vi "Striptest.vi"(1 "Simulation?":bool) -> ()   [LabVIEW 2018]
uses:
  InstrControl/ProbeStationControl/TeslaVelox/TeslaVeloxProbeStation.lvclass
  C:/Users/itkstriplabview4/Documents/itk-strip-sensor-qc/InstrControl/ProbeStationControl/ProbeStationControl.lvclass
  general_VIs/globals/QC_MeasurementSetup.vi
  striptest/ProbePlan/ProbePlanParams.vi
  general_VIs/globals/QC_RunInformation.vi
  InstrControl/InstrumentSetup.vi
  <vilib>/regexp/Match Regular Expression.xnode
  InstrControl/SupplyControl/SupplyControl.lvclass
  InstrControl/Switching/Switching.lvclass
  InstrControl/ProbeStationControl/ProbeStationControl.lvclass
  InstrControl/LCRControl/LCRControl.lvclass
  InstrControl/InstrControl.lvclass
  InstrControl/ArduinoControl/ArduinoControl.lvclass
  <vilib>/Analysis/NI_AALBase.lvlib
  InstrControl/ProbeStationControl/TeslaVelox/TeslaVelox_GlobalConfig.vi
  InstrControl/Switching/Pickering/Pickering.lvclass
  <instrlib>/CascadeProbestation/CascadeProbestation.lvlib
  C:/Users/itkstriplabview4/Documents/itk-strip-sensor-qc/InstrControl/Switching/Switching.lvclass
panel:
  in  "PreSave Data":bool
  out "RH [%]":dbl=35.18 format="%.2f"
  out "Temp [°C]":dbl=22.06 format="%.2f"
  in  "settling\ndelay [ms]":i32=1000
  in  "Auto quit &\nswitch off bias":bool
  in  "Rolling\nCurrent Readout":bool
  out "Status":string="Saving data for Segment\t3T"
  in  "Set display for:":u16(ring)=3
  out "Initiated:":string
  out "Defects":i32[][](graph)=[[0], [1], [1], [1], [1], [1], [1], [1], [1], [1], [1], [1], [1], [1], [1], [1], [1], [1], [1], [1], [1], [1], [1], [1], [1], [1], [1], [1], [1], [1], [1], [1], [1], [1], [1], [1], [1], [1], [1], [1], [1], [1], [1], [1], [1], [1], [1], [1], [1], [1], [1], [1], [1], [1], [1], [1], [1], [1], [1], [1], [1], [1], [1], [1], [1], [1], [1], [1], [1], [1], [1], [1], [1], [1], [1], [1], [1], [1], [1], [1], [1], [1], [1], [1], [1], [1], [1], [1], [1], [1], [1], [1], [1], [1], [1], [1], [1], [1], [1], [1], [1], [1], [1], [1], [1], [1], [1], [1], [1], [1], [1], [1], [1], [1], [1], [1], [1], [1], [1], [1], [1], [1], [1], [1], [1], [1], [1], [1], [1], [1], [1], [1], [1], [1], [1], [1], [1], [1], [1], [1], [1], [1], [1], [1], [1], [1], [1], [1], [1], [1], [1], [1], [1], [1], [1], [1], [1], [1], [1], [1], [1], [1], [1], [1], [1], [1], [1], [1], [1], [1], [1], [1], [1], [1], [1], [1], [1], [1], [1], [1], [1], [1], [1], [1], [1], [1], [1], [1], [1], [1], [1], [1], [1], [1], [1], [1], [1], [1], [1], [1], [1], [1], [1], [1], [1], [1], [1], [1], [1], [1], [1], [1], [1], [1], [1], [1], [1], [1], [1], [1], [1], [1], [1], [1], [1], [1], [1], [1], [1], [1], [1], [1], [1], [1], [1], [1], [1], [1], [1], [1], [1], [1], [1], [1], [1], [1], [1], [1], [1], [1], [1], [1], [1], [1], [1], [1], [1], [1], [1], [1], [1], [1], [1], [1], [1], [1], [1], [1], [1], [1], [1], [1], [1], [1], [1], [1], [1], [1], [1], [1], [1], [1], [1], [1], [1], [1], [1], [1], [1], [1], [1], [1], [1], [1], [1], [1], [1], [1], [1], [1], [1], [1], [1], [1], [1], [1], [1], [1], [1], [1], [1], [1], [1], [1], [1], [1], [1], [1], [1], [1], [1], [1], [1], [1], [1], [1], [1], [1], [1], [1], [1], [1], [1], [1], [1], [1], [1], [1], [1], [1], [1], [1], [1], [1], [1], [1], [1], [1], [1], [1], [1], [1], [1], [1], [1], [1], [1], [1], [1], [1], [1], [1], [1], [1], [1], [1], [1], [1], [1], [1], [1], [1], [1], [1], [1], [1], [1], [1], [1], [1], [1], [1], [1], [1], [1], [1], [1], [1], [1], [1], [1], [1], [1], [1], [1], [1], [1], [1], [1], [1], [1], [1], [1], [1], [1], [1], [1], [1], [1], [1], [1], [1], [1], [1], [1], [1], [1], [1], [1], [1], [1], [1], [1], [1], [1], [1], [1], [1], [1], [1], [1], [1], [1], [1], [1], [1], [1], [1], [1], [1], [1], [1], [1], [1], [1], [1], [1], [1], [1], [1], [1], [1], [1], [1], [1], [1], [1], [1], [1], [1], [1], [1], [1], [1], [1], [1], [1], [1], [1], [1], [1], [1], [1], [1], [1], [1], [1], [1], [1], [1], [1], [1], [1], [1], [1], [1], [1], [1], [1], [1], [1], [1], [1], [1], [1], [1], [1], [1], [1], [1], [1], [1], [1], [1], [1], [1], [1], [1], [1], [1], [1], [1], [1], [1], [1], [1], [1], [1], [1], [1], [1], [1], [1], [1], [1], [1], [1], [1], [1], [1], [1], [1], [1], [1], [1], [1], [1], [1], [1], [1], [1], [1], [1], [1], [1], [1], [1], [1], [1], [1], [1], [1], [1], [1], [1], [1], [1], [1], [1], [1], [1], [1], [1], [1], [1], [1], [1], [1], [1], [1], [1], [1], [1], [1], [1], [1], [1], [1], [1], [1], [1], [1], [1], [1], [1], [1], [1], [1], [1], [1], [1], [1], [1], [1], [1], [1], [1], [1], [1], [1], [1], [1], [1], [1], [1], [1], [1], [1], [1], [1], [1], [1], [1], [1], [1], [1], [1], [1], [1], [1], [1], [1], [1], [1], [1], [1], [1], [1], [1], [1], [1], [1], [1], [1], [1], [1], [1], [1], [1], [1], [1], [1], [1], [1], [1], [1], [1], [1], [1], [1], [1], [1], [1], [1], [1], [1], [1], [1], [1], [1], [1], [1], [1], [1], [1], [1], [1], [1], [1], [1], [1], [1], [1], [1], [1], [1], [1], [1], [1], [1], [1], [1], [1], [1], [1], [1], [1], [1], [1], [1], [1], [1], [1], [1], [1], [1], [1], [1], [1], [1], [1], [1], [1], [1], [1], [1], [1], [1], [1], [1], [1], [1], [1], [1], [1], [1], [1], [1], [1], [1], [1], [1], [1], [1], [1], [1], [1], [1], [1], [1], [1], [1], [1], [1], [1], [1], [1], [1], [1], [1], [1], [1], [1], [1], [1], [1], [1], [1], [1], [1], [1], [1], [1], [1], [1], [1], [1], [1], [1], [1], [1], [1], [1], [1], [1], [1], [1], [1], [1], [1], [1], [1], [1], [1], [1], [1], [1], [1], [1], [1], [1], [1], [1], [1], [1], [1], [1], [1], [1], [1], [1], [1], [1], [1], [1], [1], [1], [1], [1], [1], [1], [1], [1], [1], [1], [1], [1], [1], [1], [1], [1], [1], [1], [1], [1], [1], [1], [1], [1], [1], [1], [1], [1], [1], [1], [1], [1], [1], [1], [1], [1], [1], [1], [1], [1], [1], [1], [1], [1], [1], [1], [1], [1], [1], [1], [1], [1], [1], [1], [1], [1], [1], [1], [1], [1], [1], [1], [1], [1], [1], [1], [1], [1], [1], [1], [1], [1], [1], [1], [1], [1], [1], [1], [1], [1], [1], [1], [1], [1], [1], [1], [1], [1], [1], [1], [1], [1], [1], [1], [1], [1], [1], [1], [1], [1], [1], [1], [1], [1], [1], [1], [1], [1], [1], [1], [1], [1], [1], [1], [1], [1], [1], [1], [1], [1], [1], [1], [1], [1], [1], [1], [1], [1], [1], [1], [1], [1], [1], [1], [1], [1], [1], [1], [1], [1], [1], [1], [1], [1], [1], [1], [1], [1], [1], [1], [1], [1], [1], [1], [1], [1], [1], [1], [1], [1], [1], [1], [1], [1], [1], [1], [1], [1], [1], [1], [1], [1], [1], [1], [1], [1], [1], [1], [1], [1], [1], [1], [1], [1], [1], [1], [1], [1], [1], [1], [1], [1], [1], [1], [1], [1], [1], [1], [1], [1], [1], [1], [1], [1], [1], [1], [1], [1], [1], [1], [1], [1], [1], [1], [1], [1], [1], [1], [1], [1], [1], [1], [1], [1], [1], [1], [1], [1], [1], [1], [1], [1], [1], [1], [1], [1], [1], [1], [1], [1], [1], [1], [1], [1], [1], [1], [1], [1], [1], [1], [1], [1], [1], [1], [1], [1], [1], [1], [1], [1], [1], [1], [1], [1], [1], [1], [1], [1], [1], [1], [1], [1], [1], [1], [1], [1], [1], [1], [1], [1], [1], [1], [1], [1], [1], [1], [1], [1], [1], [1], [1], [1], [1], [1], [1], [1], [1], [1], [1], [1], [1], [1], [1], [1], [1], [1], [1], [1], [1], [1], [1], [1], [1], [1], [1], [1], [1], [1], [1], [1], [1], [1], [1], [1], [1], [1], [1], [1], [1], [1], [1], [1], [1], [1], [1], [1], [1], [1], [1], [1], [1], [1], [1], [1], [1], [1], [1], [1], [1], [1], [1], [1], [1], [1], [1], [1], [1], [1], [1], [1]]
  out "Bias On/Off:":bool=TRUE
  in  "Quit w/o saving":bool
  in  "Abort":bool
  in  "Save Data":bool=TRUE
  in  "ReCheck":bool
  in  "Auto ReCheck":bool
  out "Estimated Completion Time":string="20:44:26"
  out "Run Duration:":string="02:13:30"
  out "Last Probe at:":string="8:44:21 PM"
  out "Reistance [MW]:":dbl=1.4864199999999999
  out "Capacitance [pF]:":dbl=75.3359
  out "Current [nA]:":dbl=0.09
  out "Probe Point:":string="Strip\t1154"
  out "Probing Region:":string="Segment\t3T"
  out "% OK:":dbl=100.0
  out "# total defects:":i32
  out "# probed":i32=1154
  out "Stats:":string="Segment\t3T"
  in  "Display Stats":bool=TRUE
  out "Bad Strip List":i32[](array[numeric])=[-1, -1, -1, -1, -1, -1, -1, -1, -1, -1, -1, -1, -1, -1, -1, -1, -1, -1, -1, -1, -1, -1, -1, -1, -1, -1, -1, -1, -1, -1, -1, -1, -1, -1, -1, -1, -1, -1, -1, -1, -1, -1, -1, -1, -1, -1, -1, -1, -1, -1, -1, -1, -1, -1, -1, -1, -1, -1, -1, -1, -1, -1, -1, -1, -1, -1, -1, -1, -1, -1, -1, -1, -1, -1, -1, -1, -1, -1, -1, -1, -1, -1, -1, -1, -1, -1, -1, -1, -1, -1, -1, -1, -1, -1, -1, -1, -1, -1, -1, -1, -1, -1, -1, -1, -1, -1, -1, -1, -1, -1, -1, -1, -1, -1, -1, -1, -1, -1, -1, -1, -1, -1, -1, -1, -1, -1, -1, -1, -1, -1, -1, -1, -1, -1, -1, -1, -1, -1, -1, -1, -1, -1, -1, -1, -1, -1, -1, -1, -1, -1, -1, -1, -1, -1, -1, -1, -1, -1, -1, -1, -1, -1, -1, -1, -1, -1, -1, -1, -1, -1, -1, -1, -1, -1, -1, -1, -1, -1, -1, -1, -1, -1, -1, -1, -1, -1, -1, -1, -1, -1, -1, -1, -1, -1, -1, -1, -1, -1, -1, -1, -1, -1, -1, -1, -1, -1, -1, -1, -1, -1, -1, -1, -1, -1, -1, -1, -1, -1, -1, -1, -1, -1, -1, -1, -1, -1, -1, -1, -1, -1, -1, -1, -1, -1, -1, -1, -1, -1, -1, -1, -1, -1, -1, -1, -1, -1, -1, -1, -1, -1, -1, -1, -1, -1, -1, -1, -1, -1, -1, -1, -1, -1, -1, -1, -1, -1, -1, -1, -1, -1, -1, -1, -1, -1, -1, -1, -1, -1, -1, -1, -1, -1, -1, -1, -1, -1, -1, -1, -1, -1, -1, -1, -1, -1, -1, -1, -1, -1, -1, -1, -1, -1, -1, -1, -1, -1, -1, -1, -1, -1, -1, -1, -1, -1, -1, -1, -1, -1, -1, -1, -1, -1, -1, -1, -1, -1, -1, -1, -1, -1, -1, -1, -1, -1, -1, -1, -1, -1, -1, -1, -1, -1, -1, -1, -1, -1, -1, -1, -1, -1, -1, -1, -1, -1, -1, -1, -1, -1, -1, -1, -1, -1, -1, -1, -1, -1, -1, -1, -1, -1, -1, -1, -1, -1, -1, -1, -1, -1, -1, -1, -1, -1, -1, -1, -1, -1, -1, -1, -1, -1, -1, -1, -1, -1, -1, -1, -1, -1, -1, -1, -1, -1, -1, -1, -1, -1, -1, -1, -1, -1, -1, -1, -1, -1, -1, -1, -1, -1, -1, -1, -1, -1, -1, -1, -1, -1, -1, -1, -1, -1, -1, -1, -1, -1, -1, -1, -1, -1, -1, -1, -1, -1, -1, -1, -1, -1, -1, -1, -1, -1, -1, -1, -1, -1, -1, -1, -1, -1, -1, -1, -1, -1, -1, -1, -1, -1, -1, -1, -1, -1, -1, -1, -1, -1, -1, -1, -1, -1, -1, -1, -1, -1, -1, -1, -1, -1, -1, -1, -1, -1, -1, -1, -1, -1, -1, -1, -1, -1, -1, -1, -1, -1, -1, -1, -1, -1, -1, -1, -1, -1, -1, -1, -1, -1, -1, -1, -1, -1, -1, -1, -1, -1, -1, -1, -1, -1, -1, -1, -1, -1, -1, -1, -1, -1, -1, -1, -1, -1, -1, -1, -1, -1, -1, -1, -1, -1, -1, -1, -1, -1, -1, -1, -1, -1, -1, -1, -1, -1, -1, -1, -1, -1, -1, -1, -1, -1, -1, -1, -1, -1, -1, -1, -1, -1, -1, -1, -1, -1, -1, -1, -1, -1, -1, -1, -1, -1, -1, -1, -1, -1, -1, -1, -1, -1, -1, -1, -1, -1, -1, -1, -1, -1, -1, -1, -1, -1, -1, -1, -1, -1, -1, -1, -1, -1, -1, -1, -1, -1, -1, -1, -1, -1, -1, -1, -1, -1, -1, -1, -1, -1, -1, -1, -1, -1, -1, -1, -1, -1, -1, -1, -1, -1, -1, -1, -1, -1, -1, -1, -1, -1, -1, -1, -1, -1, -1, -1, -1, -1, -1, -1, -1, -1, -1, -1, -1, -1, -1, -1, -1, -1, -1, -1, -1, -1, -1, -1, -1, -1, -1, -1, -1, -1, -1, -1, -1, -1, -1, -1, -1, -1, -1, -1, -1, -1, -1, -1, -1, -1, -1, -1, -1, -1, -1, -1, -1, -1, -1, -1, -1, -1, -1, -1, -1, -1, -1, -1, -1, -1, -1, -1, -1, -1, -1, -1, -1, -1, -1, -1, -1, -1, -1, -1, -1, -1, -1, -1, -1, -1, -1, -1, -1, -1, -1, -1, -1, -1, -1, -1, -1, -1, -1, -1, -1, -1, -1, -1, -1, -1, -1, -1, -1, -1, -1, -1, -1, -1, -1, -1, -1, -1, -1, -1, -1, -1, -1, -1, -1, -1, -1, -1, -1, -1, -1, -1, -1, -1, -1, -1, -1, -1, -1, -1, -1, -1, -1, -1, -1, -1, -1, -1, -1, -1, -1, -1, -1, -1, -1, -1, -1, -1, -1, -1, -1, -1, -1, -1, -1, -1, -1, -1, -1, -1, -1, -1, -1, -1, -1, -1, -1, -1, -1, -1, -1, -1, -1, -1, -1, -1, -1, -1, -1, -1, -1, -1, -1, -1, -1, -1, -1, -1, -1, -1, -1, -1, -1, -1, -1, -1, -1, -1, -1, -1, -1, -1, -1, -1, -1, -1, -1, -1, -1, -1, -1, -1, -1, -1, -1, -1, -1, -1, -1, -1, -1, -1, -1, -1, -1, -1, -1, -1, -1, -1, -1, -1, -1, -1, -1, -1, -1, -1, -1, -1, -1, -1, -1, -1, -1, -1, -1, -1, -1, -1, -1, -1, -1, -1, -1, -1, -1, -1, -1, -1, -1, -1, -1, -1, -1, -1, -1, -1, -1, -1, -1, -1, -1, -1, -1, -1, -1, -1, -1, -1, -1, -1, -1, -1, -1, -1, -1, -1, -1, -1, -1, -1, -1, -1, -1, -1, -1, -1, -1, -1, -1, -1, -1, -1, -1, -1, -1, -1, -1, -1, -1, -1, -1, -1, -1, -1, -1, -1, -1, -1, -1, -1, -1, -1, -1, -1, -1, -1, -1, -1, -1, -1, -1, -1, -1, -1, -1, -1, -1, -1, -1, -1, -1, -1, -1, -1, -1, -1, -1, -1, -1, -1, -1, -1, -1, -1, -1, -1, -1, -1, -1, -1, -1, -1, -1, -1, -1, -1, -1, -1, -1, -1, -1, -1, -1, -1, -1, -1, -1, -1, -1, -1, -1, -1, -1, -1, -1, -1, -1, -1, -1, -1, -1, -1, -1, -1, -1, -1, -1, -1, -1, -1, -1, -1, -1, -1, -1, -1, -1, -1, -1, -1, -1, -1, -1, -1, -1, -1, -1, -1, -1, -1, -1, -1, -1, -1, -1, -1, -1, -1, -1, -1, -1, -1, -1, -1, -1, -1, -1, -1, -1, -1, -1, -1, -1, -1, -1, -1, -1, -1, -1, -1, -1, -1, -1, -1, -1, -1, -1, -1, -1, -1, -1, -1, -1, -1, -1, -1, -1, -1, -1, -1, -1, -1, -1, -1, -1, -1, -1, -1, -1, -1, -1, -1, -1, -1, -1, -1, -1, -1, -1, -1]
  out "defect type array":i32[](array[numeric])
  out "Probe Card Channels":i32=1
  out "Measurement Details:":string="Striptest"
  out "Operator:":string="Jiri Kv"
  out "DataBase Serial No.:":string="a"
  out "Manufacturer:":string="d"
  out "Device Category:":string="R0"
  out "Manufacturer Serial No.:":string="b56"
  in  "Thresholds":T1={"Current [nA]"=200.0, "Cap_Lo"=40.0, "Cap_Hi"=80.0, "Res_Hi"=1.6, "Res_Lo"=1.4}
  in  "Measurement Parameters":T2={"Base Bias [V]"=10.0, "Base Ramp\n[V/step]"=10.0, "High Bias [V]"=100.0, "High Ramp\n[V/step]"=1000.0, "High Step [ms]"=1000, "Base Step [ms]"=100}
  out "Resistance [MW]":cluster{u32, i32, "Array OUT":dbl[]}(graph)={1, 1, "Array OUT"=[1.52711, 1.52293, 1.52396, 1.52393, 1.5222499999999999, 1.5242, 1.52345, 1.52379, 1.5258099999999999, 1.52363, 1.52382, 1.52563, 1.52209, 1.52356, 1.5226, 1.52237, 1.52264, 1.52417, 1.52287, 1.52781, 1.52466, 1.52754, 1.52693, 1.52583, 1.5253299999999999, 1.52555, 1.52378, 1.52531, 1.5234699999999999, 1.52473, 1.52406, 1.52083, 1.5228, 1.5237399999999999, 1.52483, 1.52155, 1.52711, 1.5725, 1.52568, 1.5246899999999999, 1.5252999999999999, 1.5269, 1.5268199999999998, 1.5264, 1.52649, 1.5247899999999999, 1.52447, 1.52505, 1.52399, 1.52457, 1.52419, 1.52563, 1.52305, 1.52407, 1.5251, 1.52517, 1.52196, 1.52287, 1.52304, 1.52307, 1.52585, 1.5247, 1.52393, 1.52498, 1.52514, 1.52678, 1.52718, 1.52566, 1.52664, 1.5249199999999998, 1.5240099999999999, 1.52674, 1.52684, 1.5244099999999998, 1.5229899999999998, 1.52558, 1.52237, 1.5219399999999998, 1.52393, 1.52315, 1.5225, 1.52606, 1.52349, 1.52693, 1.5254699999999999, 1.52466, 1.5230899999999998, 1.5267899999999999, 1.52634, 1.5265499999999999, 1.52695, 1.5251299999999999, 1.52395, 1.52422, 1.5228199999999998, 1.52664, 1.52495, 1.5229, 1.52515, 1.52393, 1.52352, 1.5228, 1.5234299999999998, 1.52583, 1.52295, 1.52514, 1.5268, 1.5242, 1.52545, 1.5270199999999998, 1.5259099999999999, 1.5259699999999998, 1.54271, 1.52552, 1.5227, 1.5281, 1.52463, 1.52464, 1.5264799999999998, 1.52609, 1.5209599999999999, 1.52386, 1.52439, 1.52639, 1.52341, 1.52294, 1.52338, 1.5223099999999998, 1.52507, 1.5209, 1.5222099999999998, 1.5207499999999998, 1.52485, 1.52223, 1.52216, 1.5245499999999998, 1.5260399999999998, 1.5242099999999998, 1.52745, 1.52773, 1.52415, 1.52264, 1.5251899999999998, 1.52207, 1.5241399999999998, 1.5226, 1.52488, 1.52449, 1.52287, 1.51996, 1.52356, 1.52298, 1.52267, 1.52371, 1.5223799999999998, 1.52657, 1.52752, 1.52758, 1.52738, 1.52563, 1.5270199999999998, 1.52887, 1.52856, 1.5271299999999999, 1.52711, 1.5279699999999998, 1.52781, 1.52986, 1.53087, 1.5320099999999999, 1.5314599999999998, 1.52973, 1.5300799999999999, 1.5303099999999998, 1.53172, 1.5296299999999998, 1.52942, 1.53273, 1.52961, 1.53105, 1.53148, 1.53159, 1.5341, 1.5340099999999999, 1.53294, 1.5323, 1.5328, 1.5339, 1.5311299999999999, 1.5308199999999998, 1.53015, 1.53073, 1.53318, 1.53013, 1.5296699999999999, 1.52894, 1.53203, 1.5299099999999999, 1.53131, 1.53183, 1.5292999999999999, 1.52925, 1.53122, 1.53223, 1.5324799999999998, 1.52837, 1.5303, 1.5288, 1.52874, 1.53083, 1.53181, 1.53003, 1.53168, 1.53304, 1.53063, 1.5310599999999999, 1.53121, 1.53237, 1.53049, 1.53103, 1.53493, 1.53358, 1.53548, 1.53132, 1.5336699999999999, 1.53063, 1.5296699999999999, 1.53317, 1.53117, 1.5313299999999999, 1.52937, 1.52901, 1.52925, 1.52634, 1.52782, 1.5267, 1.5264799999999998, 1.52729, 1.52748, 1.52995, 1.5287899999999999, 1.52555, 1.5282099999999998, 1.52718, 1.52576, 1.52704, 1.52409, 1.52451, 1.5255699999999999, 1.52257, 1.5258699999999998, 1.52406, 1.5243499999999999, 1.52426, 1.52274, 1.52356, 1.52338, 1.52331, 1.522, 1.52202, 1.52307, 1.52338, 1.52565, 1.52312, 1.52087, 1.51999, 1.52071, 1.5174699999999999, 1.51796, 1.51366, 1.5166899999999999, 1.5127899999999999, 1.51336, 1.50841, 1.51291, 1.5096399999999999, 1.5083799999999998, 1.5052999999999999, 1.50748, 1.5097699999999998, 1.50946, 1.51003, 1.5098699999999998, 1.5087, 1.50634, 1.5081, 1.5090299999999999, 1.5063, 1.5092999999999999, 1.5080799999999999, 1.5074299999999998, 1.50707, 1.57999, 1.50362, 1.50529, 1.50658, 1.50779, 1.50758, 1.50799, 1.5098099999999999, 1.50819, 1.50905, 1.51168, 1.50891, 1.50972, 1.51217, 1.5129, 1.5113699999999999, 1.50936, 1.5114299999999998, 1.5125499999999998, 1.51078, 1.5129199999999998, 1.51341, 1.51379, 1.5104, 1.5128899999999998, 1.51014, 1.5134299999999998, 1.5145199999999999, 1.514, 1.51525, 1.5172599999999998, 1.51597, 1.51571, 1.51427, 1.51488, 1.51644, 1.51407, 1.5120399999999998, 1.51273, 1.51392, 1.51595, 1.5161099999999998, 1.51633, 1.51965, 1.5172599999999998, 1.5179799999999999, 1.51799, 1.5188199999999998, 1.51914, 1.51786, 1.51834, 1.51976, 1.51839, 1.5182499999999999, 1.51898, 1.51978, 1.5194699999999999, 1.51667, 1.5179099999999999, 1.51999, 1.5191999999999999, 1.51666, 1.51779, 1.51376, 1.5134299999999998, 1.51349, 1.51329, 1.51227, 1.51044, 1.51378, 1.51471, 1.51599, 1.5194299999999998, 1.5183499999999999, 1.51982, 1.5186, 1.51922, 1.52583, 1.52491, 1.52379, 1.52362, 1.5221799999999999, 1.5227499999999998, 1.52322, 1.52405, 1.52335, 1.5232299999999999, 1.5224199999999999, 1.52363, 1.5244799999999998, 1.52302, 1.5259, 1.5284799999999998, 1.52976, 1.5301099999999999, 1.52951, 1.52878, 1.53294, 1.52972, 1.53206, 1.53054, 1.5354599999999998, 1.53063, 1.5310899999999998, 1.5319099999999999, 1.53439, 1.53165, 1.53467, 1.5302399999999998, 1.53, 1.53139, 1.5327199999999999, 1.53351, 1.5343099999999998, 1.53287, 1.53162, 1.5316999999999998, 1.5326, 1.53118, 1.53334, 1.53165, 1.53324, 1.5285199999999999, 1.5309599999999999, 1.52897, 1.53257, 1.5269599999999999, 1.5299699999999998, 1.53046, 1.53073, 1.52849, 1.5309899999999999, 1.52796, 1.53138, 1.5318699999999998, 1.52911, 1.52971, 1.5297699999999999, 1.52961, 1.52998, 1.5322, 1.53225, 1.5276699999999999, 1.53051, 1.53019, 1.53134, 1.5285799999999998, 1.5326799999999998, 1.53067, 1.5337699999999999, 1.52961, 1.53212, 1.53144, 1.53505, 1.53078, 1.5301, 1.52973, 1.5320799999999999, 1.53054, 1.53423, 1.52982, 1.52979, 1.53137, 1.53301, 1.53049, 1.52979, 1.5332599999999998, 1.5341, 1.53134, 1.52999, 1.53229, 1.5299, 1.5324799999999998, 1.52986, 1.53139, 1.53105, 1.52996, 1.52965, 1.53098, 1.5302099999999998, 1.5309, 1.53225, 1.53107, 1.52939, 1.53046, 1.52887, 1.52887, 1.529, 1.52903, 1.52883, 1.52868, 1.52895, 1.52989, 1.5298699999999998, 1.5296699999999999, 1.5280799999999999, 1.52701, 1.52766, 1.52786, 1.52829, 1.52842, 1.5264199999999999, 1.5279, 1.525, 1.5284, 1.52836, 1.5268199999999998, 1.52388, 1.52829, 1.5239699999999998, 1.52605, 1.52633, 1.52876, 1.52843, 1.5287, 1.5261, 1.52915, 1.5281099999999999, 1.5282799999999999, 1.52576, 1.5301399999999998, 1.52681, 1.52989, 1.52483, 1.5289199999999998, 1.5269899999999998, 1.52504, 1.5237999999999998, 1.52859, 1.52579, 1.52737, 1.52276, 1.52663, 1.52415, 1.52566, 1.52354, 1.52704, 1.52142, 1.52566, 1.5228899999999999, 1.5238699999999998, 1.52005, 1.5251899999999998, 1.521, 1.52346, 1.5200799999999999, 1.5226499999999998, 1.52141, 1.52166, 1.52129, 1.52267, 1.5204499999999999, 1.5217399999999999, 1.5204499999999999, 1.52291, 1.51851, 1.52084, 1.51993, 1.5236999999999998, 1.5180399999999998, 1.52, 1.5205, 1.52264, 1.51959, 1.52417, 1.52156, 1.5224, 1.52027, 1.52254, 1.51938, 1.52234, 1.5196999999999998, 1.52522, 1.52324, 1.52551, 1.52128, 1.52369, 1.52307, 1.5224, 1.52322, 1.52464, 1.52407, 1.52545, 1.52119, 1.52678, 1.5225199999999999, 1.52806, 1.5246899999999999, 1.5235999999999998, 1.5213999999999999, 1.52344, 1.51834, 1.52315, 1.52093, 1.5207199999999998, 1.51985, 1.5229, 1.5197699999999998, 1.52274, 1.5184199999999999, 1.5231, 1.52249, 1.5208899999999999, 1.52205, 1.52223, 1.5195699999999999, 1.52301, 1.51938, 1.5247499999999998, 1.52098, 1.52088, 1.51834, 1.5220399999999998, 1.51802, 1.5206899999999999, 1.51844, 1.51993, 1.51932, 1.52105, 1.51812, 1.51995, 1.51941, 1.52233, 1.51866, 1.52152, 1.51813, 1.52267, 1.52284, 1.5215999999999998, 1.52358, 1.52351, 1.52006, 1.52152, 1.52118, 1.51979, 1.52135, 1.51918, 1.5230899999999998, 1.52308, 1.52046, 1.52599, 1.52078, 1.5223499999999999, 1.52033, 1.52163, 1.52227, 1.5230899999999998, 1.524, 1.5248199999999998, 1.5252299999999999, 1.5232299999999999, 1.52247, 1.52478, 1.52368, 1.52327, 1.52223, 1.52206, 1.52362, 1.52379, 1.5254699999999999, 1.5223799999999998, 1.52849, 1.52609, 1.5252599999999998, 1.52535, 1.5263, 1.5269599999999999, 1.52664, 1.52881, 1.52935, 1.5265199999999999, 1.52996, 1.52815, 1.52603, 1.52761, 1.52843, 1.52859, 1.5258099999999999, 1.52664, 1.52893, 1.52571, 1.52775, 1.5261399999999998, 1.52705, 1.52524, 1.52529, 1.51883, 1.52246, 1.5214699999999999, 1.51878, 1.52056, 1.5214999999999999, 1.52063, 1.52192, 1.52081, 1.5201799999999999, 1.51918, 1.52114, 1.5199799999999999, 1.52144, 1.52196, 1.52216, 1.52171, 1.52047, 1.52209, 1.5247, 1.5230899999999998, 1.52491, 1.52081, 1.52294, 1.52068, 1.52361, 1.5221799999999999, 1.52449, 1.52247, 1.52318, 1.52002, 1.52511, 1.52243, 1.5215699999999999, 1.52178, 1.5226499999999998, 1.5216399999999999, 1.52195, 1.5205, 1.5203799999999998, 1.52003, 1.5227499999999998, 1.52068, 1.5231999999999999, 1.5211299999999999, 1.52363, 1.52229, 1.52322, 1.51942, 1.5211599999999998, 1.51734, 1.5224, 1.51993, 1.52066, 1.52, 1.5183, 1.5174999999999998, 1.51968, 1.51674, 1.51891, 1.51595, 1.51481, 1.5157399999999999, 1.51877, 1.51497, 1.5165199999999999, 1.51588, 1.5143799999999998, 1.51338, 1.51243, 1.51163, 1.5106, 1.50938, 1.51104, 1.50946, 1.50907, 1.5068899999999998, 1.50711, 1.50763, 1.50492, 1.5090599999999998, 1.5064499999999998, 1.5069, 1.50785, 1.50578, 1.50701, 1.5041, 1.50535, 1.5068, 1.50392, 1.50475, 1.5028199999999998, 1.50023, 1.49949, 1.50206, 1.5008899999999998, 1.5008, 1.4994399999999999, 1.4993299999999998, 1.501, 1.50064, 1.50129, 1.5021, 1.50373, 1.50542, 1.5032999999999999, 1.50623, 1.5056399999999999, 1.50814, 1.50623, 1.50734, 1.5057, 1.50512, 1.5046599999999999, 1.5038399999999998, 1.5016399999999999, 1.4990999999999999, 1.49776, 1.49857, 1.49423, 1.4946, 1.49524, 1.49776, 1.4951599999999998, 1.4971999999999999, 1.49343, 1.49705, 1.49446, 1.4919399999999998, 1.49162, 1.4912699999999999, 1.4884, 1.4895399999999999, 1.48565, 1.48603, 1.4886199999999998, 1.48939, 1.48861, 1.48836, 1.48868, 1.48806, 1.48616, 1.48451, 1.48194, 1.48244, 1.4832299999999998, 1.48067, 1.48094, 1.48253, 1.47816, 1.47758, 1.4764599999999999, 1.47821, 1.4795, 1.4781199999999999, 1.47826, 1.4771999999999998, 1.4752399999999999, 1.47424, 1.4751699999999999, 1.4743899999999999, 1.47447, 1.4751699999999999, 1.47016, 1.4728299999999999, 1.47281, 1.47325, 1.47074, 1.4701199999999999, 1.46904, 1.4720499999999999, 1.46976, 1.4730299999999998, 1.47126, 1.47244, 1.4701499999999998, 1.4744899999999999, 1.4715399999999998, 1.47184, 1.4743199999999999, 1.4747899999999998, 1.47399, 1.47288, 1.47375, 1.47426, 1.47291, 1.47538, 1.47491, 1.47184, 1.47367, 1.47433, 1.5337699999999999, 1.47133, 1.47206, 1.47257, 1.4750299999999998, 1.47372, 1.4762, 1.4777099999999999, 1.47634, 1.47834, 1.47881, 1.47908, 1.48031, 1.47967, 1.48104, 1.4784199999999998, 1.47994, 1.47844, 1.47933, 1.47777, 1.4798799999999999, 1.4792399999999999, 1.48219, 1.47874, 1.4792299999999998, 1.4787299999999999, 1.4790999999999999, 1.48038, 1.4798799999999999, 1.48007, 1.47729, 1.4773699999999999, 1.4807599999999999, 1.47996, 1.48281, 1.4807599999999999, 1.48016, 1.48054, 1.4810699999999999, 1.48092, 1.48068, 1.48155, 1.48376, 1.48454, 1.4829999999999999, 1.48363, 1.48365, 1.48438, 1.4802499999999998, 1.48396, 1.48122, 1.48295, 1.4825899999999999, 1.48338, 1.50033, 1.48145, 1.48336, 1.4813699999999999, 1.4820099999999998, 1.48003, 1.4795399999999999, 1.4816099999999999, 1.4823, 1.48179, 1.47878, 1.4785, 1.4790999999999999, 1.48121, 1.47872, 1.4807, 1.47878, 1.48053, 1.47783, 1.48169, 1.47877, 1.48085, 1.4804899999999999, 1.4793999999999998, 1.47877, 1.48118, 1.4807299999999999, 1.48095, 1.4795099999999999, 1.4822199999999999, 1.4790999999999999, 1.47986, 1.48091, 1.48055, 1.4809599999999998, 1.4785599999999999, 1.48116, 1.47972, 1.4798799999999999, 1.4775099999999999, 1.4767899999999998, 1.47952, 1.4775699999999998, 1.4775099999999999, 1.4782899999999999, 1.4763499999999998, 1.47603, 1.47848, 1.47714, 1.47857, 1.4758099999999998, 1.4778799999999999, 1.47723, 1.4792699999999999, 1.4779099999999998, 1.47996, 1.4777, 1.47892, 1.4780099999999998, 1.4760799999999998, 1.47972, 1.4804, 1.4804599999999999, 1.4793699999999999, 1.4797, 1.47833, 1.47773, 1.47884, 1.47573, 1.4773399999999999, 1.47884, 1.47499, 1.47755, 1.47521, 1.47687, 1.47434, 1.4767299999999999, 1.47516, 1.47614, 1.47531, 1.4738, 1.47494, 1.4742899999999999, 1.47609, 1.47819, 1.47467, 1.4781499999999999, 1.47576, 1.47593, 1.47366, 1.4740499999999999, 1.4751699999999999, 1.47305, 1.47325, 1.47068, 1.4741, 1.4704899999999999, 1.47373, 1.47159, 1.4714699999999998, 1.47057, 1.47001, 1.46894, 1.46945, 1.4702199999999999, 1.54735, 1.46894, 1.46956, 1.47001, 1.46821, 1.46906, 1.46865, 1.46899, 1.4718799999999999, 1.47009, 1.4674399999999999, 1.46655, 1.46948, 1.46728, 1.4676, 1.4667599999999998, 1.46935, 1.46753, 1.4677399999999998, 1.4665599999999999, 1.46441, 1.46587, 1.46606, 1.46715, 1.46538, 1.4665199999999998, 1.4654099999999999, 1.46687, 1.46488, 1.4675099999999999, 1.46589, 1.4659499999999999, 1.46482, 1.46522, 1.4646299999999999, 1.4654, 1.46418, 1.4683199999999998, 1.4665599999999999, 1.4638499999999999, 1.46624, 1.4648999999999999, 1.46572, 1.46367, 1.46291, 1.46474, 1.4639499999999999, 1.4627, 1.46279, 1.46311, 1.4623, 1.46301, 1.46932, 1.4654399999999999, 1.4651399999999999, 1.46759, 1.46372, 1.4657799999999999, 1.52171, 1.46444, 1.4655099999999999, 1.46807, 1.46461, 1.46423, 1.46867, 1.46684, 1.4688299999999999, 1.47026, 1.46662, 1.46804, 1.47, 1.46946, 1.4686299999999999, 1.4682199999999999, 1.46689, 1.4688999999999999, 1.4671299999999998, 1.46977, 1.47145, 1.46905, 1.47112, 1.47238, 1.47528, 1.47672, 1.47502, 1.4771999999999998, 1.47851, 1.47853, 1.55694, 1.47845, 1.47782, 1.47695, 1.47521, 1.4773699999999999, 1.4753699999999998, 1.47511, 1.48021, 1.4780799999999998, 1.48004, 1.4767899999999998, 1.4750999999999999, 1.48217, 1.4817099999999999, 1.4794699999999998, 1.48141, 1.48061, 1.48187, 1.4776399999999998, 1.47759, 1.4766, 1.47444, 1.47542, 1.4759099999999998, 1.4770299999999998, 1.47536, 1.47404, 1.4754099999999999, 1.4765199999999998, 1.4771699999999999, 1.47925, 1.47853, 1.48094, 1.48116, 1.48647, 1.48116, 1.4864199999999999]}
  out "Capacitance [pF]":cluster{u32, i32, "Array OUT":dbl[]}(graph)={1, 1, "Array OUT"=[78.2209, 77.9252, 78.32770000000001, 77.88539999999999, 78.2512, 77.9528, 78.3006, 77.9378, 78.2109, 77.8529, 78.2129, 77.8404, 78.2108, 77.8278, 78.1837, 77.8529, 78.24080000000001, 77.89150000000001, 78.2397, 77.8195, 78.1539, 77.7573, 78.1866, 77.7789, 78.1768, 77.77210000000001, 78.0845, 77.7162, 78.0454, 77.7192, 78.03009999999999, 77.68830000000001, 78.0875, 77.6277, 78.00540000000001, 77.6648, 78.0889, 77.6065, 77.98249999999999, 77.6073, 77.9807, 77.66499999999999, 78.0153, 77.6588, 78.03609999999999, 77.6417, 78.0979, 77.5894, 77.9482, 77.7332, 77.9853, 77.6366, 77.9385, 77.6673, 77.90350000000001, 77.53229999999999, 77.90639999999999, 77.52749999999999, 77.8685, 77.5809, 77.849, 77.4997, 77.9096, 77.57, 77.92370000000001, 77.54780000000001, 77.8275, 77.4745, 77.8372, 77.51549999999999, 77.8856, 77.4494, 77.8745, 77.53, 77.92569999999999, 77.4515, 77.89800000000001, 77.5569, 77.9251, 77.4756, 77.86880000000001, 77.4476, 77.8666, 77.4453, 77.85749999999999, 77.4517, 77.8706, 77.4824, 77.8431, 77.484, 77.8082, 77.499, 77.8552, 77.48780000000001, 77.8117, 77.4026, 77.7512, 77.4247, 77.733, 77.4631, 77.816, 77.4425, 77.8178, 77.3586, 77.7935, 77.40599999999999, 77.705, 77.40520000000001, 77.7598, 77.3942, 77.7013, 77.3463, 77.8239, 77.41199999999999, 77.7495, 77.3603, 77.7026, 77.3866, 77.6905, 77.38149999999999, 77.76249999999999, 77.3254, 77.7549, 77.3361, 77.661, 77.381, 77.7512, 77.3806, 77.81200000000001, 77.3156, 77.70439999999999, 77.3634, 77.64670000000001, 77.284, 77.7017, 77.3621, 77.7239, 77.3762, 77.7148, 77.3079, 77.6194, 77.2645, 77.6006, 77.344, 77.6185, 77.3121, 77.6067, 77.27619999999999, 77.66250000000001, 77.2496, 77.66329999999999, 77.2154, 77.65350000000001, 77.25, 77.66499999999999, 77.2506, 77.5924, 77.2399, 77.599, 77.2507, 77.594, 77.2025, 77.55879999999999, 77.2075, 77.57039999999999, 77.1956, 77.6203, 77.15809999999999, 77.51679999999999, 77.1955, 77.5834, 77.24080000000001, 77.6185, 77.2339, 77.5749, 77.2397, 77.5926, 77.14519999999999, 77.5595, 77.2499, 77.6012, 77.25389999999999, 77.5459, 77.15910000000001, 77.5226, 77.2292, 77.4983, 77.19449999999999, 77.4729, 77.16669999999999, 77.5119, 77.18509999999999, 77.4763, 77.16839999999999, 77.4846, 77.13550000000001, 77.41709999999999, 77.1081, 77.4749, 77.0975, 77.5149, 77.06880000000001, 77.448, 77.07910000000001, 77.4818, 77.157, 77.4534, 77.06670000000001, 77.4792, 77.04379999999999, 77.44900000000001, 77.07870000000001, 77.4483, 77.0942, 77.426, 77.06219999999999, 77.43209999999999, 77.1544, 77.4774, 77.0874, 77.43379999999999, 77.0613, 77.4451, 77.1253, 77.4765, 77.0413, 77.4088, 77.09309999999999, 77.4692, 77.0898, 77.3933, 77.1312, 77.40440000000001, 77.06139999999999, 77.3968, 77.1167, 77.381, 77.0138, 77.3755, 77.03960000000001, 77.4353, 77.0102, 77.3629, 77.03150000000001, 77.41510000000001, 77.0286, 77.3661, 77.05030000000001, 77.31739999999999, 77.0385, 77.3246, 77.0522, 77.34030000000001, 76.95219999999999, 77.3151, 76.93090000000001, 77.37950000000001, 76.932, 77.3181, 77.024, 77.3656, 76.9723, 77.3453, 76.9617, 77.2657, 76.97109999999999, 77.316, 76.89989999999999, 77.26480000000001, 76.9031, 77.2587, 76.83019999999999, 77.2268, 76.8764, 77.2554, 76.874, 77.19239999999999, 76.8456, 77.2372, 76.9592, 77.1974, 76.8763, 77.2203, 76.90589999999999, 77.20179999999999, 76.865, 77.24080000000001, 76.8344, 77.1738, 76.8697, 77.154, 76.835, 77.14949999999999, 76.93169999999999, 77.1352, 76.956, 77.2452, 76.7964, 77.2113, 76.7853, 77.1517, 76.7801, 77.1653, 76.7761, 77.1281, 76.7763, 77.16810000000001, 76.7409, 77.1978, 76.7519, 77.1213, 76.7722, 77.131, 76.828, 77.1285, 76.8086, 77.09779999999999, 76.8172, 77.0908, 76.82480000000001, 77.1066, 76.81410000000001, 77.1619, 76.7745, 77.0801, 76.7827, 77.1781, 76.8344, 77.0974, 76.8163, 77.09609999999999, 76.69850000000001, 77.14989999999999, 76.8077, 77.0989, 76.7735, 77.1764, 76.7677, 77.1341, 76.7588, 77.0758, 76.7226, 77.03580000000001, 76.7739, 77.0769, 76.7794, 77.0402, 76.76350000000001, 77.1208, 76.791, 77.0995, 76.6888, 77.1061, 76.7203, 77.02810000000001, 76.7311, 77.0952, 76.7152, 77.0098, 76.7396, 77.0823, 76.7401, 77.02080000000001, 76.7537, 77.075, 76.7567, 77.03309999999999, 76.6583, 77.07469999999999, 76.6684, 77.02449999999999, 76.69069999999999, 76.9815, 76.68430000000001, 77.01180000000001, 76.69879999999999, 77.03779999999999, 76.6288, 77.0723, 76.6717, 77.05550000000001, 76.6953, 76.9793, 76.6828, 76.9562, 76.70110000000001, 76.948, 76.6196, 76.9749, 76.65650000000001, 77.0583, 76.6013, 77.0119, 76.6879, 76.9997, 76.6293, 76.9896, 76.6329, 76.9876, 76.6923, 77.0078, 76.66749999999999, 76.9888, 76.6107, 77.0115, 76.6437, 76.9653, 76.6478, 77.0068, 76.5904, 76.9856, 76.67, 77.0323, 76.7302, 77.0799, 76.5993, 76.9449, 76.6364, 77.0183, 76.58940000000001, 76.9676, 76.56219999999999, 77.0124, 76.57469999999999, 76.93419999999999, 76.5703, 76.9401, 76.56880000000001, 76.96679999999999, 76.55919999999999, 77.0051, 76.56389999999999, 76.9602, 76.5424, 76.9639, 76.5564, 76.91080000000001, 76.6437, 76.91720000000001, 76.5863, 76.8758, 76.5473, 76.9268, 76.5603, 76.8784, 76.5637, 76.92779999999999, 76.6144, 76.9137, 76.6066, 76.9888, 76.55879999999999, 76.9667, 76.5724, 76.897, 76.57480000000001, 76.8712, 76.5353, 76.9097, 76.56349999999999, 76.94109999999999, 76.5202, 76.8816, 76.60379999999999, 76.91460000000001, 76.5889, 76.8948, 76.57889999999999, 76.94080000000001, 76.54119999999999, 76.93639999999999, 76.57820000000001, 76.866, 76.56920000000001, 76.8592, 76.56620000000001, 76.9014, 76.48649999999999, 76.93440000000001, 76.56389999999999, 76.8644, 76.58789999999999, 76.8599, 76.58619999999999, 76.91810000000001, 76.4857, 76.8897, 76.5013, 76.915, 76.4869, 76.84970000000001, 76.4836, 76.8905, 76.4743, 76.80789999999999, 76.4987, 76.80850000000001, 76.44279999999999, 76.8074, 76.5488, 76.81089999999999, 76.46310000000001, 76.9088, 76.43220000000001, 76.8403, 76.4971, 76.773, 76.5169, 76.7679, 76.5146, 76.83319999999999, 76.53129999999999, 76.8183, 76.5002, 76.82979999999999, 76.4332, 76.7593, 76.42190000000001, 76.7967, 76.47640000000001, 76.855, 76.515, 76.7873, 76.4614, 76.7643, 76.4434, 76.7539, 76.4469, 76.80420000000001, 76.5054, 76.7596, 76.45519999999999, 76.8439, 76.4905, 76.84009999999999, 76.4083, 76.838, 76.497, 76.8233, 76.4791, 76.82780000000001, 76.409, 76.7394, 76.4921, 76.7535, 76.4919, 76.77980000000001, 76.4679, 76.7257, 76.4001, 76.767, 76.43759999999999, 76.7957, 76.4134, 76.72749999999999, 76.44760000000001, 76.7543, 76.4182, 76.7214, 76.4808, 76.7392, 76.3838, 76.70920000000001, 76.3756, 76.7814, 76.4087, 76.7579, 76.3266, 76.7709, 76.3343, 76.7255, 76.4027, 76.7246, 76.3657, 76.7173, 76.36319999999999, 76.70920000000001, 76.3618, 76.6836, 76.3685, 76.657, 76.3479, 76.665, 76.34280000000001, 76.7345, 76.3584, 76.6618, 76.3227, 76.7427, 76.3356, 76.65459999999999, 76.3206, 76.70920000000001, 76.30189999999999, 76.7299, 76.32130000000001, 76.6409, 76.3783, 76.70779999999999, 76.3534, 76.6643, 76.2786, 76.69, 76.31620000000001, 76.7205, 76.2918, 76.69749999999999, 76.38419999999999, 76.6203, 76.35419999999999, 76.6476, 76.2702, 76.6091, 76.32939999999999, 76.5967, 76.31490000000001, 76.57169999999999, 76.2366, 76.6634, 76.31150000000001, 76.6694, 76.2295, 76.5927, 76.3424, 76.67450000000001, 76.29329999999999, 76.616, 76.23410000000001, 76.58980000000001, 76.2852, 76.5371, 76.2629, 76.5943, 76.184, 76.5377, 76.20280000000001, 76.5363, 76.1935, 76.562, 76.2454, 76.56360000000001, 76.18329999999999, 76.6081, 76.18, 76.5814, 76.19149999999999, 76.5816, 76.21090000000001, 76.56, 76.1558, 76.4879, 76.19579999999999, 76.4923, 76.1383, 76.4765, 76.17299999999999, 76.552, 76.1141, 76.476, 76.18, 76.48179999999999, 76.1598, 76.4872, 76.142, 76.46390000000001, 76.11449999999999, 76.45609999999999, 76.1576, 76.5346, 76.18159999999999, 76.4646, 76.1104, 76.5033, 76.1653, 76.478, 76.0762, 76.492, 76.1351, 76.4846, 76.16699999999999, 76.4761, 76.09320000000001, 76.441, 76.09859999999999, 76.4832, 76.0476, 76.4128, 76.09819999999999, 76.40990000000001, 76.0654, 76.4263, 76.1396, 76.3874, 76.1324, 76.45909999999999, 76.0718, 76.4767, 76.1206, 76.3823, 76.0847, 76.3908, 76.0314, 76.3797, 76.0279, 76.3901, 76.1141, 76.46379999999999, 76.0943, 76.4494, 76.078, 76.4487, 76.1195, 76.374, 76.06620000000001, 76.4118, 76.0597, 76.4321, 76.08879999999999, 76.3564, 76.0158, 76.4212, 76.0367, 76.3387, 76.07159999999999, 76.4267, 76.0418, 76.4332, 75.98389999999999, 76.3903, 76.0104, 76.3984, 76.0633, 76.3322, 75.9841, 76.4054, 76.06230000000001, 76.34060000000001, 76.0391, 76.3739, 76.0634, 76.31559999999999, 76.0519, 76.3107, 75.975, 76.3871, 76.0035, 76.2962, 75.98689999999999, 76.34519999999999, 76.0367, 76.3766, 75.96560000000001, 76.33, 75.97789999999999, 76.4224, 75.97420000000001, 76.28920000000001, 75.9478, 76.34150000000001, 75.9411, 76.3348, 75.9919, 76.4045, 75.9674, 76.3078, 75.9957, 76.3464, 75.99719999999999, 76.3147, 76.0091, 76.3044, 75.9748, 76.2825, 75.9306, 76.3237, 75.9561, 76.35, 75.9348, 76.3558, 76.0395, 76.3414, 76.0185, 76.3604, 75.96350000000001, 76.2983, 75.9537, 76.3228, 75.9932, 76.3457, 76.041, 76.3846, 75.99780000000001, 76.32050000000001, 76.0628, 76.33359999999999, 75.9814, 76.3261, 76.0202, 76.34389999999999, 75.962, 76.45779999999999, 75.9533, 76.2897, 75.9524, 76.2898, 76.0161, 76.306, 75.9488, 76.3187, 76.0052, 76.3607, 75.9465, 76.3594, 76.0078, 76.287, 76.0306, 76.2721, 75.9588, 76.3384, 75.9414, 76.3297, 75.9971, 76.34989999999999, 76.0294, 76.3544, 76.0075, 76.3424, 75.98989999999999, 76.31559999999999, 75.981, 76.2599, 75.97890000000001, 76.2951, 75.97659999999999, 76.3001, 75.9974, 76.285, 75.9797, 76.2713, 75.9145, 76.293, 75.93629999999999, 76.3377, 75.9208, 76.30489999999999, 75.9135, 76.2631, 76.0009, 76.3098, 76.0135, 76.3258, 76.001, 76.3516, 76.0016, 76.3424, 75.9359, 76.2685, 75.9375, 76.379, 76.0071, 76.3701, 75.9145, 76.3231, 75.9353, 76.3813, 75.9149, 76.30330000000001, 75.93430000000001, 76.2729, 76.0903, 76.3054, 75.9538, 76.2588, 75.9923, 76.3172, 75.93759999999999, 76.263, 75.9679, 76.2483, 75.865, 76.2866, 75.9709, 76.31, 75.8553, 76.3048, 75.9349, 76.313, 75.9172, 76.2261, 75.9396, 76.2582, 75.8446, 76.2324, 75.8939, 76.1825, 75.8557, 76.20320000000001, 75.9213, 76.2654, 75.8308, 76.2714, 75.8258, 76.2748, 75.8038, 76.1834, 75.8374, 76.1634, 75.8357, 76.254, 75.7943, 76.2338, 75.9064, 76.2011, 75.7807, 76.1402, 75.8202, 76.215, 75.7963, 76.11250000000001, 75.7902, 76.1574, 75.7733, 76.20779999999999, 75.7376, 76.1411, 75.7736, 76.099, 75.7487, 76.1675, 75.7719, 76.0897, 75.7516, 76.08630000000001, 75.83330000000001, 76.1758, 75.7432, 76.07730000000001, 75.8053, 76.1455, 75.75019999999999, 76.10820000000001, 75.8053, 76.1547, 75.7854, 76.0617, 75.8067, 76.0753, 75.7789, 76.1487, 75.7488, 76.06960000000001, 75.71719999999999, 76.1758, 75.72070000000001, 76.16720000000001, 75.775, 76.04069999999999, 75.72579999999999, 76.1417, 75.6895, 76.0464, 75.789, 76.0496, 75.7584, 76.0711, 75.7044, 76.07090000000001, 75.6954, 76.0321, 75.7248, 76.1148, 75.7737, 76.1118, 75.7785, 76.1309, 75.68069999999999, 76.0236, 75.67660000000001, 76.0167, 75.72189999999999, 76.0266, 75.81960000000001, 76.1193, 75.6979, 76.0285, 75.6805, 76.0274, 75.7466, 76.0364, 75.7265, 76.1185, 75.71640000000001, 76.0783, 75.70689999999999, 76.0402, 75.7274, 76.0737, 75.7491, 76.0976, 75.63119999999999, 76.0427, 75.729, 75.974, 75.7244, 76.0908, 75.6779, 75.96900000000001, 75.6727, 76.0648, 75.6604, 76.0312, 75.6469, 75.9808, 75.6361, 75.94630000000001, 75.62490000000001, 76.0207, 75.59020000000001, 75.94189999999999, 75.6151, 75.95360000000001, 75.56790000000001, 76.0066, 75.6633, 75.9977, 75.6531, 76.0012, 75.5659, 76.0357, 75.5372, 75.91869999999999, 75.6642, 75.8988, 75.627, 75.8667, 75.5796, 75.8974, 75.5607, 75.89189999999999, 75.5945, 75.93759999999999, 75.4948, 75.9408, 75.5172, 75.86160000000001, 75.57969999999999, 75.8601, 75.5163, 75.9408, 75.52029999999999, 75.8917, 75.5272, 75.9167, 75.4891, 75.8223, 75.4769, 75.8952, 75.4701, 75.911, 75.5195, 75.8561, 75.50420000000001, 75.8421, 75.47269999999999, 75.8523, 75.5037, 75.8313, 75.4316, 75.8111, 75.4662, 75.85759999999999, 75.4525, 75.8717, 75.5051, 75.7492, 75.4008, 75.8024, 75.4439, 75.8288, 75.4594, 75.75789999999999, 75.4855, 75.82459999999999, 75.5121, 75.8208, 75.48270000000001, 75.8015, 75.4183, 75.84150000000001, 75.3978, 75.7833, 75.47540000000001, 75.8228, 75.4838, 75.7848, 75.4642, 75.8519, 75.4225, 75.76859999999999, 75.4511, 75.74990000000001, 75.393, 75.7552, 75.4464, 75.8017, 75.4394, 75.801, 75.4622, 75.7836, 75.35600000000001, 75.7104, 75.4245, 75.7071, 75.3424, 75.6658, 75.4251, 75.69829999999999, 75.3711, 75.6793, 75.3462, 75.70519999999999, 75.36449999999999, 75.71220000000001, 75.3234, 75.6762, 75.299, 75.6943, 75.28359999999999, 75.6483, 75.2813, 75.5441, 75.1941, 75.4721, 75.0783, 75.4709, 75.0247, 75.3853, 74.9382, 75.2681, 74.9164, 75.2881, 74.9225, 75.34129999999999, 74.9642, 75.2917, 75.0349, 75.2983, 74.98100000000001, 75.4195, 75.12360000000001, 75.46300000000001, 75.1888, 75.60119999999999, 75.3359]}
  out "Current [nA]":cluster{u32, i32, "Array OUT":dbl[]}(graph)={1, 1, "Array OUT"=[0.09, 0.09, 0.06, 0.08, 0.08, 0.08, 0.08, 0.08, 0.07, 0.06, 0.07, 0.07, 0.07, 0.07, 0.07, 0.07, 0.07, 0.07, 0.07, 0.07, 0.07, 0.07, 0.07, 0.07, 0.07, 0.07, 0.07, 0.07, 0.07, 0.07, 0.07, 0.07, 0.07, 0.07, 0.07, 0.08, 0.07, 0.07, 0.08, 0.07, 0.08, 0.05, 0.04, 0.06, 0.08, 0.07, 0.08, 0.06, 0.07, 0.08, 0.08, 0.07, 0.07, 0.07, 0.07, 0.05, 0.08, 0.05, 0.05, 0.07, 0.08, 0.07, 0.07, 0.07, 0.07, 0.08, 0.07, 0.08, 0.07, 0.08, 0.07, 0.08, 0.08, 0.08, 0.08, 0.07, 0.07, 0.07, 0.07, 0.07, 0.07, 0.07, 0.08, 0.07, 0.06, 0.08, 0.08, 0.07, 0.08, 0.07, 0.06, 0.07, 0.08, 0.07, 0.07, 0.08, 0.08, 0.08, 0.06, 0.08, 0.08, 0.08, 0.07, 0.07, 0.07, 0.07, 0.08, 0.08, 0.07, 0.07, 0.07, 0.07, 0.07, 0.07, 0.08, 0.07, 0.07, 0.07, 0.07, 0.07, 0.08, 0.07, 0.07, 0.07, 0.07, 0.08, 0.08, 0.08, 0.07, 0.07, 0.08, 0.08, 0.08, 0.07, 0.08, 0.08, 0.08, 0.08, 0.08, 0.08, 0.08, 0.07, 0.08, 0.07, 0.07, 0.08, 0.08, 0.08, 0.07, 0.07, 0.07, 0.08, 0.08, 0.08, 0.08, 0.07, 0.08, 0.08, 0.08, 0.08, 0.08, 0.08, 0.07, 0.07, 0.07, 0.07, 0.07, 0.08, 0.08, 0.08, 0.07, 0.08, 0.08, 0.08, 0.07, 0.08, 0.08, 0.07, 0.08, 0.09, 0.08, 0.07, 0.08, 0.08, 0.07, 0.08, 0.08, 0.07, 0.08, 0.08, 0.08, 0.08, 0.07, 0.08, 0.07, 0.08, 0.08, 0.08, 0.08, 0.07, 0.08, 0.07, 0.08, 0.08, 0.08, 0.08, 0.08, 0.07, 0.07, 0.08, 0.07, 0.08, 0.08, 0.07, 0.07, 0.08, 0.08, 0.07, 0.07, 0.07, 0.08, 0.07, 0.08, 0.07, 0.07, 0.07, 0.07, 0.08, 0.07, 0.08, 0.08, 0.08, 0.08, 0.08, 0.08, 0.08, 0.08, 0.07, 0.07, 0.08, 0.07, 0.07, 0.07, 0.07, 0.07, 0.08, 0.07, 0.07, 0.08, 0.08, 0.08, 0.08, 0.08, 0.07, 0.08, 0.08, 0.1, 0.07, 0.11, 0.08, 0.09, 0.09, 0.08, 0.09, 0.08, 0.08, 0.07, 0.1, 0.08, 0.08, 0.08, 0.08, 0.05, 0.06, 0.1, 0.06, 0.08, 0.08, 0.08, 0.08, 0.08, 0.08, 0.08, 0.08, 0.07, 0.08, 0.08, 0.06, 0.07, 0.07, 0.08, 0.07, 0.07, 0.07, 0.08, 0.07, 0.07, 0.07, 0.07, 0.07, 0.08, 0.08, 0.08, 0.07, 0.07, 0.07, 0.07, 0.07, 0.07, 0.07, 0.08, 0.08, 0.08, 0.07, 0.08, 0.08, 0.08, 0.07, 0.08, 0.07, 0.08, 0.08, 0.07, 0.08, 0.07, 0.08, 0.08, 0.08, 0.08, 0.08, 0.07, 0.07, 0.07, 0.07, 0.08, 0.08, 0.07, 0.08, 0.08, 0.08, 0.08, 0.08, 0.08, 0.07, 0.08, 0.08, 0.08, 0.08, 0.08, 0.07, 0.08, 0.08, 0.08, 0.08, 0.08, 0.07, 0.08, 0.08, 0.08, 0.08, 0.08, 0.07, 0.08, 0.07, 0.08, 0.08, 0.07, 0.08, 0.08, 0.08, 0.06, 0.07, 0.07, 0.07, 0.07, 0.08, 0.08, 0.08, 0.07, 0.07, 0.08, 0.08, 0.08, 0.08, 0.08, 0.07, 0.07, 0.06, 0.07, 0.04, 0.08, 0.07, 0.05, 0.07, 0.08, 0.08, 0.05, 0.08, 0.08, 0.07, 0.09, 0.08, 0.07, 0.08, 0.07, 0.07, 0.08, 0.08, 0.08, 0.07, 0.06, 0.07, 0.08, 0.09, 0.08, 0.07, 0.08, 0.08, 0.07, 0.07, 0.07, 0.08, 0.08, 0.07, 0.08, 0.07, 0.08, 0.06, 0.08, 0.06, 0.07, 0.09, 0.07, 0.08, 0.05, 0.08, 0.07, 0.08, 0.08, 0.08, 0.07, 0.08, 0.07, 0.07, 0.08, 0.08, 0.08, 0.08, 0.07, 0.08, 0.07, 0.07, 0.08, 0.07, 0.07, 0.07, 0.07, 0.08, 0.07, 0.08, 0.08, 0.07, 0.07, 0.07, 0.08, 0.08, 0.08, 0.07, 0.07, 0.08, 0.07, 0.08, 0.08, 0.08, 0.07, 0.07, 0.08, 0.07, 0.08, 0.05, 0.08, 0.07, 0.05, 0.08, 0.08, 0.1, 0.07, 0.09, 0.08, 0.08, 0.07, 0.08, 0.08, 0.08, 0.07, 0.07, 0.07, 0.08, 0.08, 0.08, 0.07, 0.08, 0.08, 0.09, 0.1, 0.1, 0.09, 0.09, 0.09, 0.08, 0.08, 0.07, 0.08, 0.08, 0.05, 0.08, 0.08, 0.08, 0.09, 0.08, 0.07, 0.07, 0.08, 0.08, 0.08, 0.08, 0.08, 0.07, 0.05, 0.07, 0.07, 0.05, 0.07, 0.07, 0.07, 0.08, 0.08, 0.07, 0.07, 0.07, 0.07, 0.07, 0.07, 0.06, 0.08, 0.08, 0.07, 0.07, 0.07, 0.08, 0.08, 0.07, 0.08, 0.08, 0.08, 0.07, 0.07, 0.06, 0.08, 0.07, 0.07, 0.08, 0.07, 0.08, 0.07, 0.07, 0.07, 0.08, 0.07, 0.08, 0.08, 0.08, 0.08, 0.08, 0.08, 0.08, 0.08, 0.08, 0.08, 0.08, 0.08, 0.08, 0.08, 0.07, 0.08, 0.07, 0.08, 0.07, 0.08, 0.07, 0.08, 0.08, 0.08, 0.07, 0.08, 0.08, 0.08, 0.07, 0.08, 0.07, 0.08, 0.08, 0.07, 0.08, 0.07, 0.07, 0.08, 0.1, 0.08, 0.08, 0.08, 0.08, 0.07, 0.08, 0.07, 0.08, 0.08, 0.08, 0.08, 0.08, 0.08, 0.08, 0.08, 0.07, 0.08, 0.08, 0.08, 0.07, 0.08, 0.07, 0.08, 0.07, 0.08, 0.08, 0.07, 0.07, 0.07, 0.07, 0.07, 0.08, 0.07, 0.07, 0.07, 0.08, 0.08, 0.08, 0.08, 0.07, 0.07, 0.07, 0.07, 0.08, 0.07, 0.08, 0.08, 0.08, 0.07, 0.07, 0.07, 0.07, 0.08, 0.08, 0.07, 0.07, 0.06, 0.07, 0.07, 0.07, 0.07, 0.07, 0.07, 0.07, 0.07, 0.07, 0.08, 0.07, 0.07, 0.07, 0.07, 0.08, 0.07, 0.07, 0.08, 0.07, 0.07, 0.08, 0.08, 0.05, 0.08, 0.08, 0.07, 0.07, 0.08, 0.07, 0.07, 0.07, 0.08, 0.08, 0.07, 0.07, 0.08, 0.07, 0.07, 0.07, 0.07, 0.07, 0.08, 0.06, 0.08, 0.07, 0.07, 0.07, 0.07, 0.08, 0.07, 0.07, 0.07, 0.07, 0.07, 0.07, 0.07, 0.07, 0.07, 0.07, 0.07, 0.07, 0.07, 0.07, 0.07, 0.07, 0.07, 0.05, 0.07, 0.07, 0.07, 0.07, 0.07, 0.07, 0.07, 0.07, 0.08, 0.07, 0.07, 0.07, 0.07, 0.07, 0.08, 0.07, 0.1, 0.07, 0.08, 0.07, 0.07, 0.07, 0.07, 0.07, 0.07, 0.08, 0.15, 0.07, 0.07, 0.07, 0.07, 0.07, 0.08, 0.07, 0.07, 0.07, 0.07, 0.07, 0.07, 0.07, 0.07, 0.07, 0.07, 0.08, 0.08, 0.08, 0.07, 0.07, 0.07, 0.06, 0.08, 0.07, 0.08, 0.08, 0.08, 0.07, 0.07, 0.07, 0.08, 0.08, 0.08, 0.07, 0.07, 0.07, 0.08, 0.08, 0.08, 0.07, 0.07, 0.08, 0.08, 0.07, 0.08, 0.07, 0.07, 0.08, 0.07, 0.09, 0.08, 0.08, 0.07, 0.07, 0.08, 0.07, 0.08, 0.08, 0.07, 0.07, 0.08, 0.08, 0.09, 0.07, 0.07, 0.08, 0.08, 0.08, 0.08, 0.07, 0.07, 0.08, 0.08, 0.08, 0.07, 0.07, 0.08, 0.07, 0.08, 0.08, 0.08, 0.07, 0.07, 0.07, 0.08, 0.07, 0.07, 0.07, 0.07, 0.08, 0.08, 0.07, 0.07, 0.07, 0.08, 0.07, 0.07, 0.08, 0.08, 0.08, 0.09, 0.07, 0.08, 0.07, 0.07, 0.08, 0.07, 0.08, 0.07, 0.07, 0.07, 0.08, 0.08, 0.08, 0.08, 0.07, 0.07, 0.07, 0.07, 0.07, 0.07, 0.07, 0.07, 0.07, 0.08, 0.08, 0.08, 0.08, 0.07, 0.08, 0.07, 0.08, 0.07, 0.07, 0.07, 0.07, 0.07, 0.07, 0.07, 0.07, 0.08, 0.07, 0.08, 0.09, 0.08, 0.07, 0.07, 0.07, 0.07, 0.07, 0.07, 0.07, 0.08, 0.07, 0.08, 0.07, 0.07, 0.08, 0.07, 0.07, 0.07, 0.07, 0.07, 0.07, 0.08, 0.08, 0.08, 0.07, 0.07, 0.07, 0.07, 0.07, 0.08, 0.07, 0.07, 0.07, 0.07, 0.07, 0.07, 0.07, 0.07, 0.07, 0.07, 0.07, 0.07, 0.07, 0.07, 0.07, 0.07, 0.07, 0.08, 0.08, 0.07, 0.08, 0.09, 0.07, 0.07, 0.08, 0.07, 0.07, 0.07, 0.07, 0.07, 0.07, 0.07, 0.07, 0.08, 0.09, 0.07, 0.07, 0.07, 0.07, 0.07, 0.08, 0.07, 0.07, 0.07, 0.07, 0.07, 0.07, 0.07, 0.07, 0.07, 0.07, 0.07, 0.07, 0.07, 0.07, 0.08, 0.08, 0.07, 0.08, 0.07, 0.07, 0.07, 0.07, 0.07, 0.1, 0.07, 0.08, 0.07, 0.08, 0.07, 0.1, 0.07, 0.07, 0.07, 0.07, 0.07, 0.07, 0.07, 0.07, 0.07, 0.08, 0.12, 0.07, 0.07, 0.07, 0.07, 0.07, 0.07, 0.08, 0.07, 0.09, 0.07, 0.07, 0.08, 0.07, 0.07, 0.07, 0.07, 0.07, 0.07, 0.07, 0.07, 0.07, 0.07, 0.07, 0.07, 0.07, 0.07, 0.07, 0.07, 0.07, 0.07, 0.06, 0.08, 0.07, 0.07, 0.06, 0.07, 0.07, 0.07, 0.09, 0.08, 0.07, 0.07, 0.07, 0.07, 0.07, 0.07, 0.07, 0.08, 0.07, 0.07, 0.07, 0.07, 0.07, 0.07, 0.07, 0.07, 0.07, 0.07, 0.07, 0.07, 0.07, 0.07, 0.07, 0.07, 0.07, 0.07, 0.07, 0.07, 0.08, 0.07, 0.07, 0.07, 0.07, 0.07, 0.07, 0.07, 0.07, 0.07, 0.07, 0.07, 0.07, 0.05, 0.07, 0.07, 0.07, 0.07, 0.07, 0.07, 0.07, 0.07, 0.08, 0.07, 0.05, 0.04, 0.07, 0.07, 0.07, 0.07, 0.07, 0.07, 0.07, 0.07, 0.07, 0.07, 0.07, 0.07, 0.07, 0.07, 0.07, 0.06, 0.07, 0.07, 0.07, 0.07, 0.07, 0.07, 0.06, 0.07, 0.07, 0.07, 0.07, 0.07, 0.07, 0.07, 0.07, 0.07, 0.08, 0.07, 0.08, 0.08, 0.07, 0.07, 0.08, 0.08, 0.08, 0.08, 0.08, 0.08, 0.09]}
  out "Current Reference 100V":dbl[](array[numeric])
  out "Current Reference 10V":dbl[](array[numeric])
  out "Single Needle":bool=TRUE
  out "Z profile":i32[][](array[numeric])
  out "Start Temperature [°C]":dbl
  out "Last Temperature [°C]":dbl=21.98
  out "disabled channels":i32[](array[numeric])
  out "Module failed/passed":bool=TRUE
  out "probe points per region":i32[](array[numeric])=[0, 0, 0, 1154]
  out "min scale array":i32[](array[numeric])=[-1, -1, -1, 0]
  out "max scale array":i32[](array[numeric])=[-1, -1, -1, 1153]
  out "total strip number":u32=1154
  out "Region Indices":i32[](array[numeric])=[0, 1, 2, 3]
  out "Current Bias Voltage [V]":dbl
  out "Temperature Progression":T3={"Time Array"=["00:00:03", "00:00:10", "00:00:17", "00:00:23", "00:00:30", "00:00:37", "00:00:44", "00:00:51", "00:00:58", "00:01:05", "00:01:12", "00:01:19", "00:01:25", "00:01:32", "00:01:39", "00:01:46", "00:01:53", "00:01:60", "00:02:07", "00:02:14", "00:02:21", "00:02:28", "00:02:35", "00:02:42", "00:02:48", "00:02:55", "00:03:02", "00:03:09", "00:03:16", "00:03:23", "00:03:30", "00:03:37", "00:03:44", "00:03:51", "00:03:58", "00:04:05", "00:04:11", "00:04:18", "00:04:25", "00:04:32", "00:04:39", "00:04:46", "00:04:52", "00:04:59", "00:05:07", "00:05:13", "00:05:20", "00:05:27", "00:05:34", "00:05:41", "00:05:48", "00:05:55", "00:06:01", "00:06:09", "00:06:15", "00:06:22", "00:06:29", "00:06:36", "00:06:43", "00:06:50", "00:06:57", "00:07:03", "00:07:11", "00:07:17", "00:07:24", "00:07:31", "00:07:38", "00:07:45", "00:07:52", "00:07:59", "00:08:06", "00:08:13", "00:08:19", "00:08:26", "00:08:33", "00:08:40", "00:08:47", "00:08:54", "00:09:01", "00:09:08", "00:09:15", "00:09:22", "00:09:28", "00:09:35", "00:09:42", "00:09:49", "00:09:56", "00:10:03", "00:10:10", "00:10:17", "00:10:24", "00:10:31", "00:10:37", "00:10:44", "00:10:51", "00:10:58", "00:11:05", "00:11:12", "00:11:19", "00:11:26", "00:11:32", "00:11:39", "00:11:46", "00:11:53", "00:12:00", "00:12:07", "00:12:14", "00:12:21", "00:12:27", "00:12:34", "00:12:41", "00:12:48", "00:12:55", "00:13:02", "00:13:09", "00:13:16", "00:13:22", "00:13:29", "00:13:36", "00:13:43", "00:13:50", "00:13:57", "00:14:04", "00:14:11", "00:14:18", "00:14:25", "00:14:31", "00:14:38", "00:14:45", "00:14:52", "00:14:59", "00:15:06", "00:15:13", "00:15:19", "00:15:26", "00:15:33", "00:15:40", "00:15:47", "00:15:54", "00:16:01", "00:16:08", "00:16:15", "00:16:22", "00:16:29", "00:16:35", "00:16:42", "00:16:49", "00:16:56", "00:17:03", "00:17:10", "00:17:17", "00:17:24", "00:17:31", "00:17:38", "00:17:45", "00:17:52", "00:17:58", "00:18:05", "00:18:12", "00:18:19", "00:18:26", "00:18:33", "00:18:40", "00:18:47", "00:18:54", "00:19:00", "00:19:07", "00:19:14", "00:19:21", "00:19:28", "00:19:35", "00:19:41", "00:19:48", "00:19:55", "00:20:02", "00:20:09", "00:20:16", "00:20:23", "00:20:30", "00:20:37", "00:20:44", "00:20:50", "00:20:57", "00:21:04", "00:21:11", "00:21:18", "00:21:25", "00:21:32", "00:21:39", "00:21:46", "00:21:52", "00:21:59", "00:22:06", "00:22:13", "00:22:20", "00:22:27", "00:22:33", "00:22:41", "00:22:47", "00:22:54", "00:23:01", "00:23:08", "00:23:15", "00:23:22", "00:23:29", "00:23:36", "00:23:43", "00:23:50", "00:23:57", "00:24:04", "00:24:11", "00:24:17", "00:24:24", "00:24:31", "00:24:38", "00:24:45", "00:24:53", "00:24:60", "00:25:07", "00:25:14", "00:25:20", "00:25:27", "00:25:34", "00:25:41", "00:25:48", "00:25:55", "00:26:02", "00:26:09", "00:26:16", "00:26:23", "00:26:30", "00:26:37", "00:26:43", "00:26:51", "00:26:57", "00:27:04", "00:27:11", "00:27:18", "00:27:25", "00:27:32", "00:27:39", "00:27:46", "00:27:53", "00:27:60", "00:28:07", "00:28:14", "00:28:20", "00:28:27", "00:28:34", "00:28:41", "00:28:48", "00:28:55", "00:29:02", "00:29:09", "00:29:16", "00:29:23", "00:29:30", "00:29:37", "00:29:44", "00:29:51", "00:29:58", "00:30:05", "00:30:11", "00:30:19", "00:30:25", "00:30:32", "00:30:39", "00:30:46", "00:30:53", "00:31:00", "00:31:07", "00:31:14", "00:31:21", "00:31:28", "00:31:35", "00:31:42", "00:31:49", "00:31:56", "00:32:03", "00:32:10", "00:32:17", "00:32:24", "00:32:31", "00:32:38", "00:32:45", "00:32:52", "00:32:58", "00:33:06", "00:33:12", "00:33:19", "00:33:26", "00:33:33", "00:33:40", "00:33:47", "00:33:54", "00:34:01", "00:34:08", "00:34:15", "00:34:22", "00:34:29", "00:34:35", "00:34:42", "00:34:50", "00:34:56", "00:35:03", "00:35:10", "00:35:17", "00:35:24", "00:35:31", "00:35:38", "00:35:45", "00:35:52", "00:35:59", "00:36:05", "00:36:12", "00:36:19", "00:36:26", "00:36:33", "00:36:40", "00:36:47", "00:36:54", "00:37:01", "00:37:08", "00:37:15", "00:37:22", "00:37:29", "00:37:36", "00:37:43", "00:37:50", "00:37:57", "00:38:04", "00:38:10", "00:38:18", "00:38:24", "00:38:31", "00:38:38", "00:38:45", "00:38:52", "00:38:59", "00:39:06", "00:39:13", "00:39:20", "00:39:27", "00:39:34", "00:39:41", "00:39:48", "00:39:55", "00:40:02", "00:40:08", "00:40:15", "00:40:22", "00:40:29", "00:40:36", "00:40:43", "00:40:50", "00:40:57", "00:41:04", "00:41:11", "00:41:18", "00:41:25", "00:41:32", "00:41:39", "00:41:46", "00:41:53", "00:41:59", "00:42:07", "00:42:14", "00:42:20", "00:42:27", "00:42:34", "00:42:41", "00:42:48", "00:42:55", "00:43:02", "00:43:09", "00:43:16", "00:43:23", "00:43:30", "00:43:37", "00:43:44", "00:43:51", "00:43:58", "00:44:04", "00:44:12", "00:44:18", "00:44:25", "00:44:33", "00:44:39", "00:44:46", "00:44:53", "00:44:60", "00:45:07", "00:45:14", "00:45:21", "00:45:28", "00:45:35", "00:45:42", "00:45:49", "00:45:56", "00:46:02", "00:46:09", "00:46:16", "00:46:23", "00:46:30", "00:46:37", "00:46:44", "00:46:51", "00:46:58", "00:47:05", "00:47:12", "00:47:19", "00:47:26", "00:47:33", "00:47:40", "00:47:47", "00:47:53", "00:48:00", "00:48:07", "00:48:14", "00:48:21", "00:48:28", "00:48:35", "00:48:42", "00:48:49", "00:48:56", "00:49:03", "00:49:10", "00:49:17", "00:49:24", "00:49:31", "00:49:37", "00:49:45", "00:49:52", "00:49:58", "00:50:05", "00:50:12", "00:50:19", "00:50:26", "00:50:33", "00:50:40", "00:50:47", "00:50:54", "00:51:01", "00:51:08", "00:51:15", "00:51:22", "00:51:29", "00:51:36", "00:51:43", "00:51:50", "00:51:56", "00:52:03", "00:52:10", "00:52:17", "00:52:24", "00:52:31", "00:52:38", "00:52:45", "00:52:52", "00:52:59", "00:53:06", "00:53:13", "00:53:20", "00:53:27", "00:53:34", "00:53:41", "00:53:47", "00:53:55", "00:54:01", "00:54:08", "00:54:15", "00:54:22", "00:54:29", "00:54:36", "00:54:43", "00:54:50", "00:54:57", "00:55:04", "00:55:11", "00:55:18", "00:55:25", "00:55:32", "00:55:39", "00:55:46", "00:55:52", "00:55:60", "00:56:06", "00:56:13", "00:56:20", "00:56:27", "00:56:34", "00:56:41", "00:56:48", "00:56:55", "00:57:02", "00:57:09", "00:57:16", "00:57:23", "00:57:30", "00:57:37", "00:57:44", "00:57:51", "00:57:57", "00:58:05", "00:58:11", "00:58:18", "00:58:25", "00:58:32", "00:58:39", "00:58:46", "00:58:53", "00:58:60", "00:59:07", "00:59:14", "00:59:21", "00:59:28", "00:59:35", "00:59:42", "00:59:49", "00:59:56", "01:00:02", "01:00:10", "01:00:17", "01:00:23", "01:00:30", "01:00:37", "01:00:44", "01:00:51", "01:00:58", "01:01:05", "01:01:12", "01:01:19", "01:01:26", "01:01:33", "01:01:39", "01:01:46", "01:01:54", "01:02:00", "01:02:07", "01:02:14", "01:02:21", "01:02:28", "01:02:35", "01:02:42", "01:02:49", "01:02:56", "01:03:03", "01:03:10", "01:03:17", "01:03:24", "01:03:31", "01:03:38", "01:03:45", "01:03:51", "01:03:59", "01:04:05", "01:04:12", "01:04:19", "01:04:26", "01:04:33", "01:04:40", "01:04:47", "01:04:54", "01:05:01", "01:05:08", "01:05:15", "01:05:22", "01:05:29", "01:05:36", "01:05:43", "01:05:50", "01:05:57", "01:06:04", "01:06:11", "01:06:17", "01:06:24", "01:06:31", "01:06:38", "01:06:45", "01:06:52", "01:06:59", "01:07:06", "01:07:13", "01:07:20", "01:07:27", "01:07:34", "01:07:41", "01:07:48", "01:07:54", "01:08:01", "01:08:08", "01:08:15", "01:08:22", "01:08:29", "01:08:36", "01:08:43", "01:08:50", "01:08:57", "01:09:04", "01:09:11", "01:09:18", "01:09:25", "01:09:32", "01:09:39", "01:09:46", "01:09:53", "01:09:60", "01:10:07", "01:10:14", "01:10:20", "01:10:27", "01:10:34", "01:10:41", "01:10:48", "01:10:55", "01:11:02", "01:11:09", "01:11:16", "01:11:23", "01:11:30", "01:11:37", "01:11:43", "01:11:50", "01:11:57", "01:12:04", "01:12:11", "01:12:18", "01:12:25", "01:12:32", "01:12:39", "01:12:46", "01:12:53", "01:13:00", "01:13:07", "01:13:14", "01:13:21", "01:13:28", "01:13:35", "01:13:42", "01:13:49", "01:13:56", "01:14:03", "01:14:10", "01:14:16", "01:14:23", "01:14:30", "01:14:37", "01:14:44", "01:14:51", "01:14:58", "01:15:05", "01:15:12", "01:15:19", "01:15:26", "01:15:33", "01:15:40", "01:15:47", "01:15:54", "01:16:01", "01:16:08", "01:16:15", "01:16:22", "01:16:29", "01:16:36", "01:16:43", "01:16:50", "01:16:57", "01:17:04", "01:17:11", "01:17:17", "01:17:24", "01:17:31", "01:17:38", "01:17:45", "01:17:52", "01:17:59", "01:18:06", "01:18:13", "01:18:20", "01:18:27", "01:18:34", "01:18:41", "01:18:48", "01:18:55", "01:19:02", "01:19:09", "01:19:16", "01:19:23", "01:19:30", "01:19:37", "01:19:44", "01:19:51", "01:19:58", "01:20:04", "01:20:11", "01:20:18", "01:20:25", "01:20:32", "01:20:39", "01:20:46", "01:20:53", "01:21:00", "01:21:07", "01:21:14", "01:21:21", "01:21:28", "01:21:35", "01:21:42", "01:21:49", "01:21:56", "01:22:03", "01:22:10", "01:22:17", "01:22:24", "01:22:30", "01:22:37", "01:22:44", "01:22:51", "01:22:58", "01:23:05", "01:23:12", "01:23:19", "01:23:26", "01:23:33", "01:23:40", "01:23:47", "01:23:54", "01:24:00", "01:24:08", "01:24:15", "01:24:22", "01:24:29", "01:24:35", "01:24:42", "01:24:49", "01:24:56", "01:25:03", "01:25:10", "01:25:17", "01:25:24", "01:25:31", "01:25:38", "01:25:45", "01:25:52", "01:25:59", "01:26:06", "01:26:13", "01:26:20", "01:26:26", "01:26:33", "01:26:40", "01:26:47", "01:26:54", "01:27:01", "01:27:08", "01:27:15", "01:27:22", "01:27:29", "01:27:36", "01:27:43", "01:27:50", "01:27:57", "01:28:04", "01:28:11", "01:28:18", "01:28:25", "01:28:31", "01:28:39", "01:28:45", "01:28:52", "01:28:59", "01:29:06", "01:29:13", "01:29:20", "01:29:27", "01:29:34", "01:29:41", "01:29:48", "01:29:55", "01:30:03", "01:30:10", "01:30:17", "01:30:24", "01:30:31", "01:30:38", "01:30:45", "01:30:52", "01:30:58", "01:31:06", "01:31:12", "01:31:19", "01:31:26", "01:31:33", "01:31:40", "01:31:47", "01:31:54", "01:32:01", "01:32:08", "01:32:15", "01:32:22", "01:32:29", "01:32:36", "01:32:43", "01:32:50", "01:32:57", "01:33:04", "01:33:11", "01:33:18", "01:33:25", "01:33:32", "01:33:39", "01:33:46", "01:33:53", "01:34:00", "01:34:07", "01:34:14", "01:34:21", "01:34:28", "01:34:35", "01:34:42", "01:34:49", "01:34:56", "01:35:03", "01:35:10", "01:35:17", "01:35:23", "01:35:30", "01:35:37", "01:35:44", "01:35:51", "01:35:58", "01:36:05", "01:36:12", "01:36:19", "01:36:26", "01:36:33", "01:36:40", "01:36:47", "01:36:54", "01:37:01", "01:37:08", "01:37:14", "01:37:21", "01:37:28", "01:37:35", "01:37:42", "01:37:49", "01:37:56", "01:38:03", "01:38:10", "01:38:17", "01:38:24", "01:38:31", "01:38:38", "01:38:45", "01:38:52", "01:38:59", "01:39:06", "01:39:13", "01:39:19", "01:39:26", "01:39:33", "01:39:40", "01:39:48", "01:39:54", "01:40:01", "01:40:08", "01:40:15", "01:40:22", "01:40:29", "01:40:36", "01:40:43", "01:40:50", "01:40:57", "01:41:04", "01:41:11", "01:41:18", "01:41:25", "01:41:32", "01:41:38", "01:41:45", "01:41:52", "01:41:59", "01:42:06", "01:42:13", "01:42:20", "01:42:27", "01:42:34", "01:42:41", "01:42:48", "01:42:55", "01:43:02", "01:43:08", "01:43:16", "01:43:22", "01:43:29", "01:43:36", "01:43:43", "01:43:50", "01:43:57", "01:44:04", "01:44:11", "01:44:18", "01:44:25", "01:44:32", "01:44:39", "01:44:46", "01:44:52", "01:44:59", "01:45:06", "01:45:13", "01:45:20", "01:45:27", "01:45:34", "01:45:41", "01:45:48", "01:45:55", "01:46:02", "01:46:09", "01:46:16", "01:46:23", "01:46:29", "01:46:36", "01:46:43", "01:46:50", "01:46:57", "01:47:04", "01:47:11", "01:47:18", "01:47:25", "01:47:32", "01:47:39", "01:47:46", "01:47:53", "01:47:60", "01:48:07", "01:48:14", "01:48:21", "01:48:28", "01:48:35", "01:48:42", "01:48:49", "01:48:56", "01:49:03", "01:49:10", "01:49:16", "01:49:23", "01:49:30", "01:49:37", "01:49:44", "01:49:51", "01:49:58", "01:50:05", "01:50:12", "01:50:19", "01:50:26", "01:50:33", "01:50:40", "01:50:47", "01:50:54", "01:51:01", "01:51:08", "01:51:15", "01:51:22", "01:51:28", "01:51:35", "01:51:42", "01:51:49", "01:51:56", "01:52:03", "01:52:10", "01:52:17", "01:52:24", "01:52:31", "01:52:38", "01:52:45", "01:52:52", "01:52:59", "01:53:06", "01:53:13", "01:53:20", "01:53:27", "01:53:34", "01:53:41", "01:53:48", "01:53:55", "01:54:02", "01:54:09", "01:54:16", "01:54:23", "01:54:30", "01:54:36", "01:54:43", "01:54:51", "01:54:57", "01:55:04", "01:55:11", "01:55:18", "01:55:25", "01:55:32", "01:55:39", "01:55:46", "01:55:53", "01:56:00", "01:56:07", "01:56:14", "01:56:21", "01:56:28", "01:56:35", "01:56:41", "01:56:49", "01:56:55", "01:57:02", "01:57:09", "01:57:16", "01:57:23", "01:57:30", "01:57:37", "01:57:44", "01:57:51", "01:57:58", "01:58:05", "01:58:12", "01:58:19", "01:58:26", "01:58:33", "01:58:40", "01:58:47", "01:58:54", "01:59:01", "01:59:08", "01:59:15", "01:59:22", "01:59:28", "01:59:36", "01:59:43", "01:59:49", "01:59:57", "02:00:03", "02:00:10", "02:00:17", "02:00:24", "02:00:31", "02:00:38", "02:00:45", "02:00:52", "02:00:59", "02:01:06", "02:01:13", "02:01:20", "02:01:27", "02:01:34", "02:01:42", "02:01:49", "02:01:56", "02:02:03", "02:02:10", "02:02:16", "02:02:24", "02:02:30", "02:02:37", "02:02:44", "02:02:51", "02:02:58", "02:03:05", "02:03:12", "02:03:19", "02:03:26", "02:03:33", "02:03:40", "02:03:47", "02:03:54", "02:04:00", "02:04:07", "02:04:14", "02:04:21", "02:04:28", "02:04:35", "02:04:42", "02:04:49", "02:04:56", "02:05:03", "02:05:10", "02:05:17", "02:05:24", "02:05:31", "02:05:38", "02:05:45", "02:05:52", "02:05:59", "02:06:06", "02:06:13", "02:06:20", "02:06:26", "02:06:33", "02:06:40", "02:06:47", "02:06:54", "02:07:01", "02:07:08", "02:07:15", "02:07:22", "02:07:29", "02:07:36", "02:07:43", "02:07:50", "02:07:57", "02:08:04", "02:08:11", "02:08:18", "02:08:25", "02:08:32", "02:08:39", "02:08:46", "02:08:53", "02:08:60", "02:09:06", "02:09:13", "02:09:21", "02:09:27", "02:09:34", "02:09:42", "02:09:48", "02:09:55", "02:10:03", "02:10:10", "02:10:16", "02:10:24", "02:10:30", "02:10:37", "02:10:44", "02:10:51", "02:10:58", "02:11:05", "02:11:12", "02:11:19", "02:11:26", "02:11:33", "02:11:40", "02:11:47", "02:11:54", "02:12:01", "02:12:08", "02:12:15", "02:12:21", "02:12:28", "02:12:35", "02:12:42", "02:12:49", "02:12:56", "02:13:03", "02:13:10", "02:13:17", "02:13:24", "02:13:30"], "Temperature Array [°C]"=array[1155 elements], "Humidity Array [RH %]"=array[1155 elements]}
  # "Striptest"
  # "Current [nA]"
  # "Capacitance [pF]"
  # "Resistance [MW]"
  # "Ok  Pinhole at base  Pinhole after ramp  Short  Open  Rbias"
  # "University of Cambridge"
  # "Current status"
  # "Statistical information"
  # "Measurement parameters"
  # "Pinholes:"
  # "Punchthroughs:"
  # "Shorts:"
  # "Opens:"
  # "Thresholds"
  # "Rpoly:"
  # "Current segment:"
  # "Implant:"
  # "DUT & test description"
  # "Current [nA]:"
  # "Capacitance [pF]:"
  # "Resistance [MW]:"
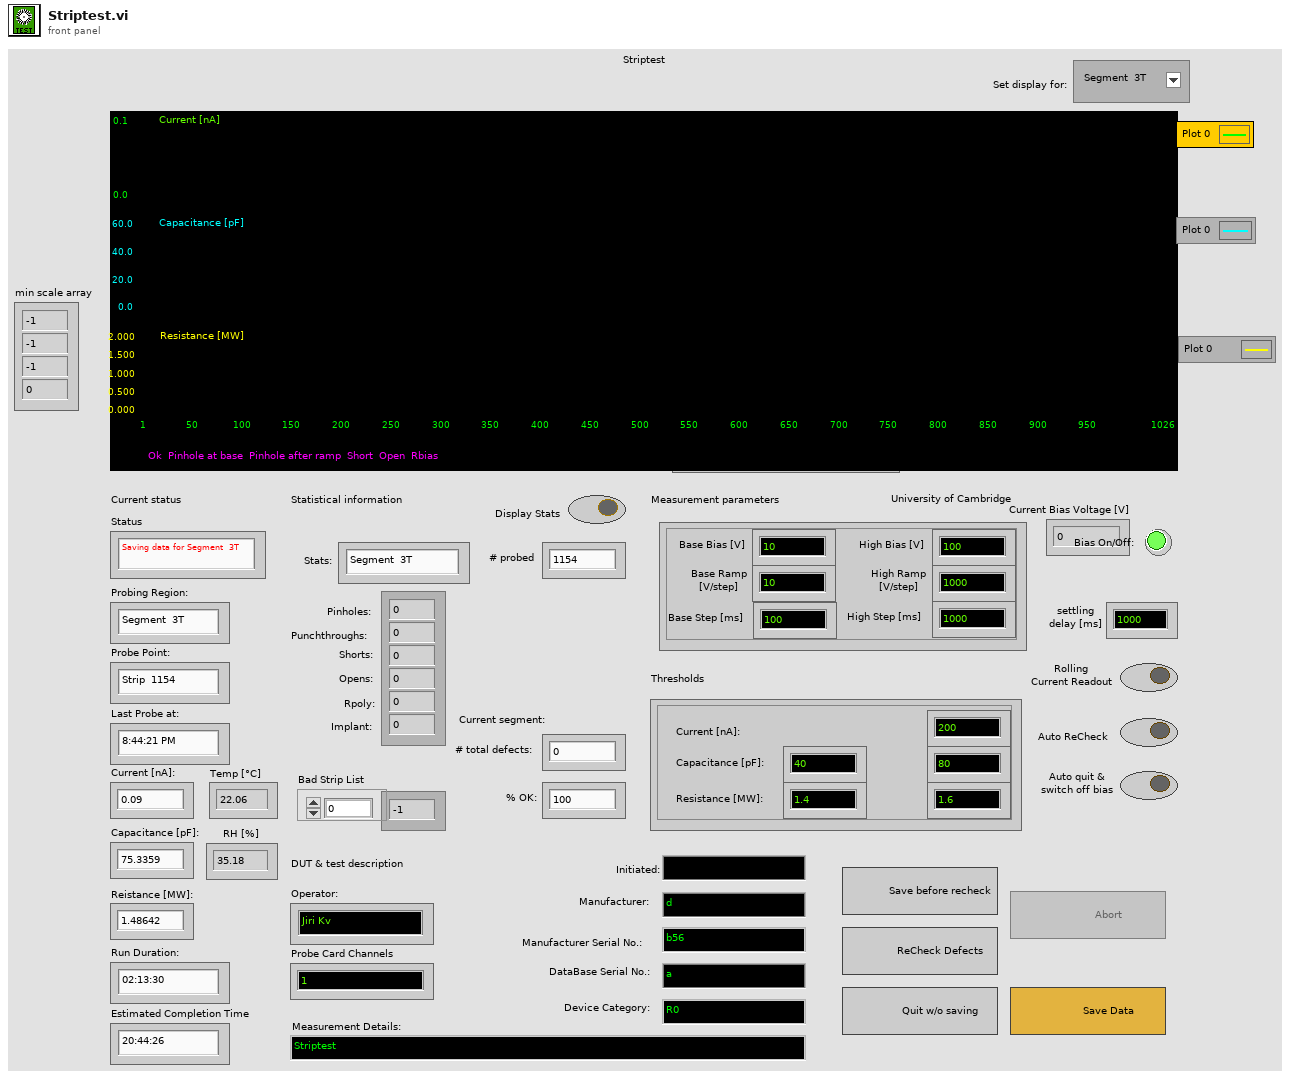
[diagram p1: front panel]
types:
  T1 = cluster{"Current [nA]":dbl, "Cap_Lo":dbl, "Cap_Hi":dbl, "Res_Hi":dbl, "Res_Lo":dbl}
  T2 = cluster{"Base Bias [V]":dbl, "Base Ramp\n[V/step]":dbl, "High Bias [V]":dbl, "High Ramp\n[V/step]":dbl, "High Step [ms]":i32, "Base Step [ms]":i32}
  T3 = cluster{"Time Array":string[], "Temperature Array [°C]":dbl[], "Humidity Array [RH %]":dbl[]}
  T4 = enum16{"Supply", "LCR", "Multimeter", "Switching"}
  T5 = enum16{"Reset", "Ground", "Striptest SMU", "Striptest LCR", "IV", "CV", "Interstrip Cap", "Interstrip Res"}
  T6 = enum16{"Reference measurement", "Baseline correcetion 10V", "Baseline correcetion 100V", "Nothing"}
  T7 = enum16{"Reset", "Read Array", "Read Element", "Write Element", "Write Array", "Add Element", "Add Array"}
  T8 = enum16{"open", "replace", "create", "open or create", "replace or create", "replace or create with confirmation"}
  T9 = cluster{"Bias Supply":refnum<class "SupplyControl.lvclass">, "SMU":refnum<class "SupplyControl.lvclass">, "LCR":refnum<class "LCRControl.lvclass">, "Probe Card Channels":i32, "Bias Voltage [V]":dbl, "First strip":i32, "Last strip":i32, "Base Voltage [V]":dbl, "Base Ramp Step [V]":dbl, "Base Ramp Interval [ms]":u32, "High Voltage [V]":dbl, "High Ramp Step [V]":dbl, "High Ramp Interval [ms]":u32, "Single Needle":bool, "Temperature Readout":enum16{"Read Arduino", "Enter manually"}, "Arduino":refnum<class "ArduinoControl.lvclass">, "Fraction of good strips [%]":dbl, "ProbeStation":refnum<class "ProbeStationControl.lvclass">, "AC frequency [Hz]":i32, "Switching":refnum<class "Switching.lvclass">, "Matrix used?":bool, "Matrix X Channels":cluster{"Bias Supply / SMU LO":i32, "Bias Supply / SMU HI":i32, "CV Box LO":i32, "CV Box HI":i32, "CV Box LO IN":i32, "CV Box HI IN":i32, "Volt meter LO":i32, "Volt meter HI":i32, "Mux1 C1":i32, "Mux1 C2":i32, "Mux2 C1":i32, "Mux2 C2":i32}, "Pinholes Y/N":bool, "Capacitance Y/N":bool, "Resistance Y/N":bool}
  T10 = cluster{"Strip Number OUT":i32, "X0":i32, "Y0":i32, "X1":i32, "Y1":i32, "Xref":dbl, "Yref":dbl, "ProbePlan type":u32, "Inner pads offset":ext, "Outer pads offset":ext, "l_inner":ext, "l_outer":ext, "strip numbering":u16, "Device Orientation":ext, "Stagger offset":i32, "Yoffset":dbl, "Strip pitch":dbl, "Fiducail separation":dbl, "Radius":ext, "Relative strip angles":dbl, "Probeplan description":string, "ProbePlan array":cluster{"Region":string, "ProbePoints":cluster{"X":dbl, "Y":dbl, "Label":string, "CardViable?":bool}[]}[], "Test ProbePoints":cluster{"Regions Enabled":bool[], "From index":u32[], "To index":u32[]}}
  T11 = cluster{"Region":string, "ProbePoints":cluster{"X":dbl, "Y":dbl, "Label":string, "CardViable?":bool}[]}[]
  T12 = cluster{"Sensor Serial No.:":string, "Wafer Serial No.:":string, "Batch:":string, "Manufacturer:":string, "Device Category:":string, "Database Serial No.:":string, "Initiated:":string, "Test":string, "Instruments used:":string, "Probeplan used:":string, "End of Run comment:":string, "User:":string}
  T13 = cluster{"VISA address":refnum<visa-resource-name>, "T sensor":enum16{"SHT", "DS"}, "Arduino":refnum<class "ArduinoControl.lvclass">}
  T14 = cluster{"X":dbl, "Y":dbl, "Label":string, "CardViable?":bool}[]
  T15 = cluster{"X":dbl, "Y":dbl, "Label":string, "CardViable?":bool}
  T16 = cluster{"pass Rate in %":dbl, "Bad channel list":i32[], "No of bad strips":i32, "Defect description list":i32[], "Number of defects per category":i32[], "Defect lists":string[], "No of channels":i32, "Defect Flag array OUT":i32[][]}
  T17 = cluster{"Hi Cap":dbl, "Lo Cap":dbl, "Current threshold":dbl, "Lo R":dbl, "Hi R":dbl}
  T18 = cluster{"Institute":string, "Manufacturers":string[], "Devices":string[], "Serialnumbers Lookup DB":string, "Data directory":string, "Backup & screenshot directory":string, "List of known users":string[]}
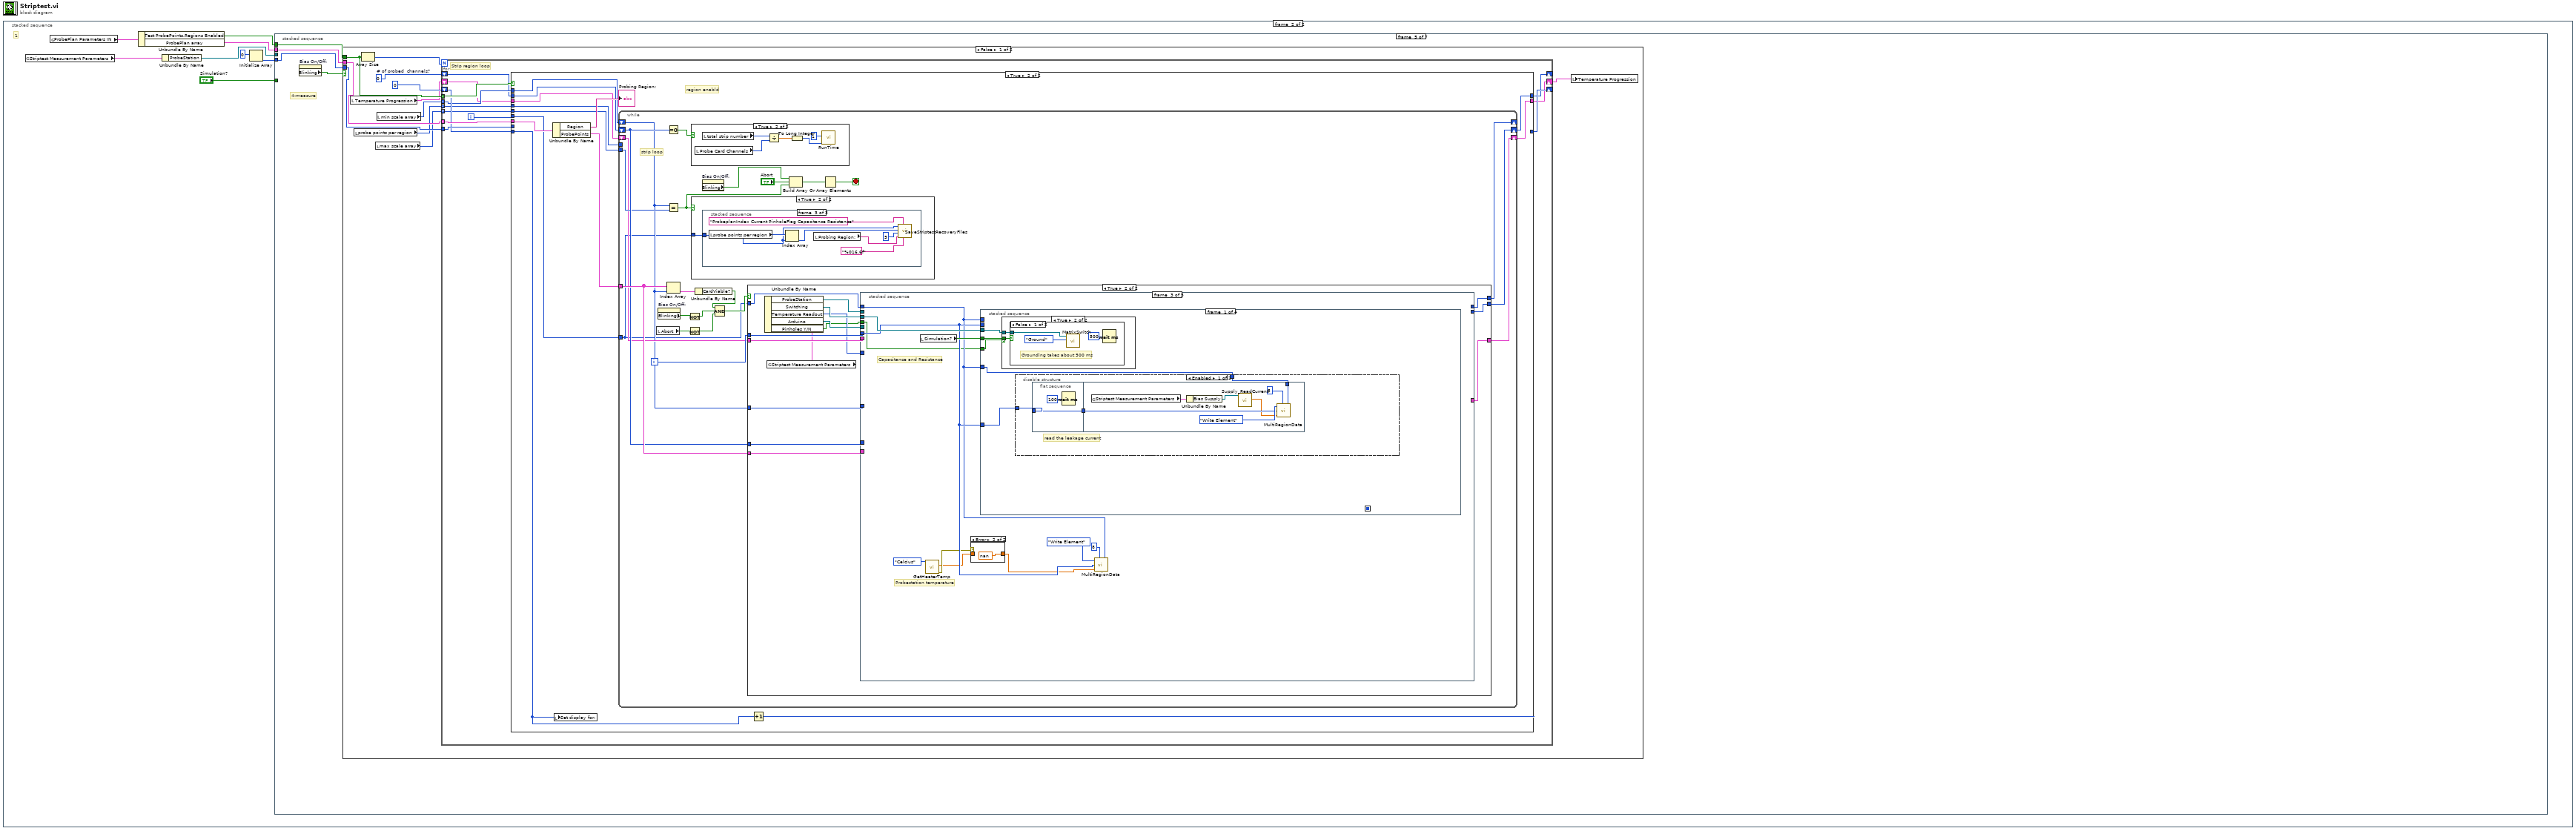
[diagram p0: block diagram]
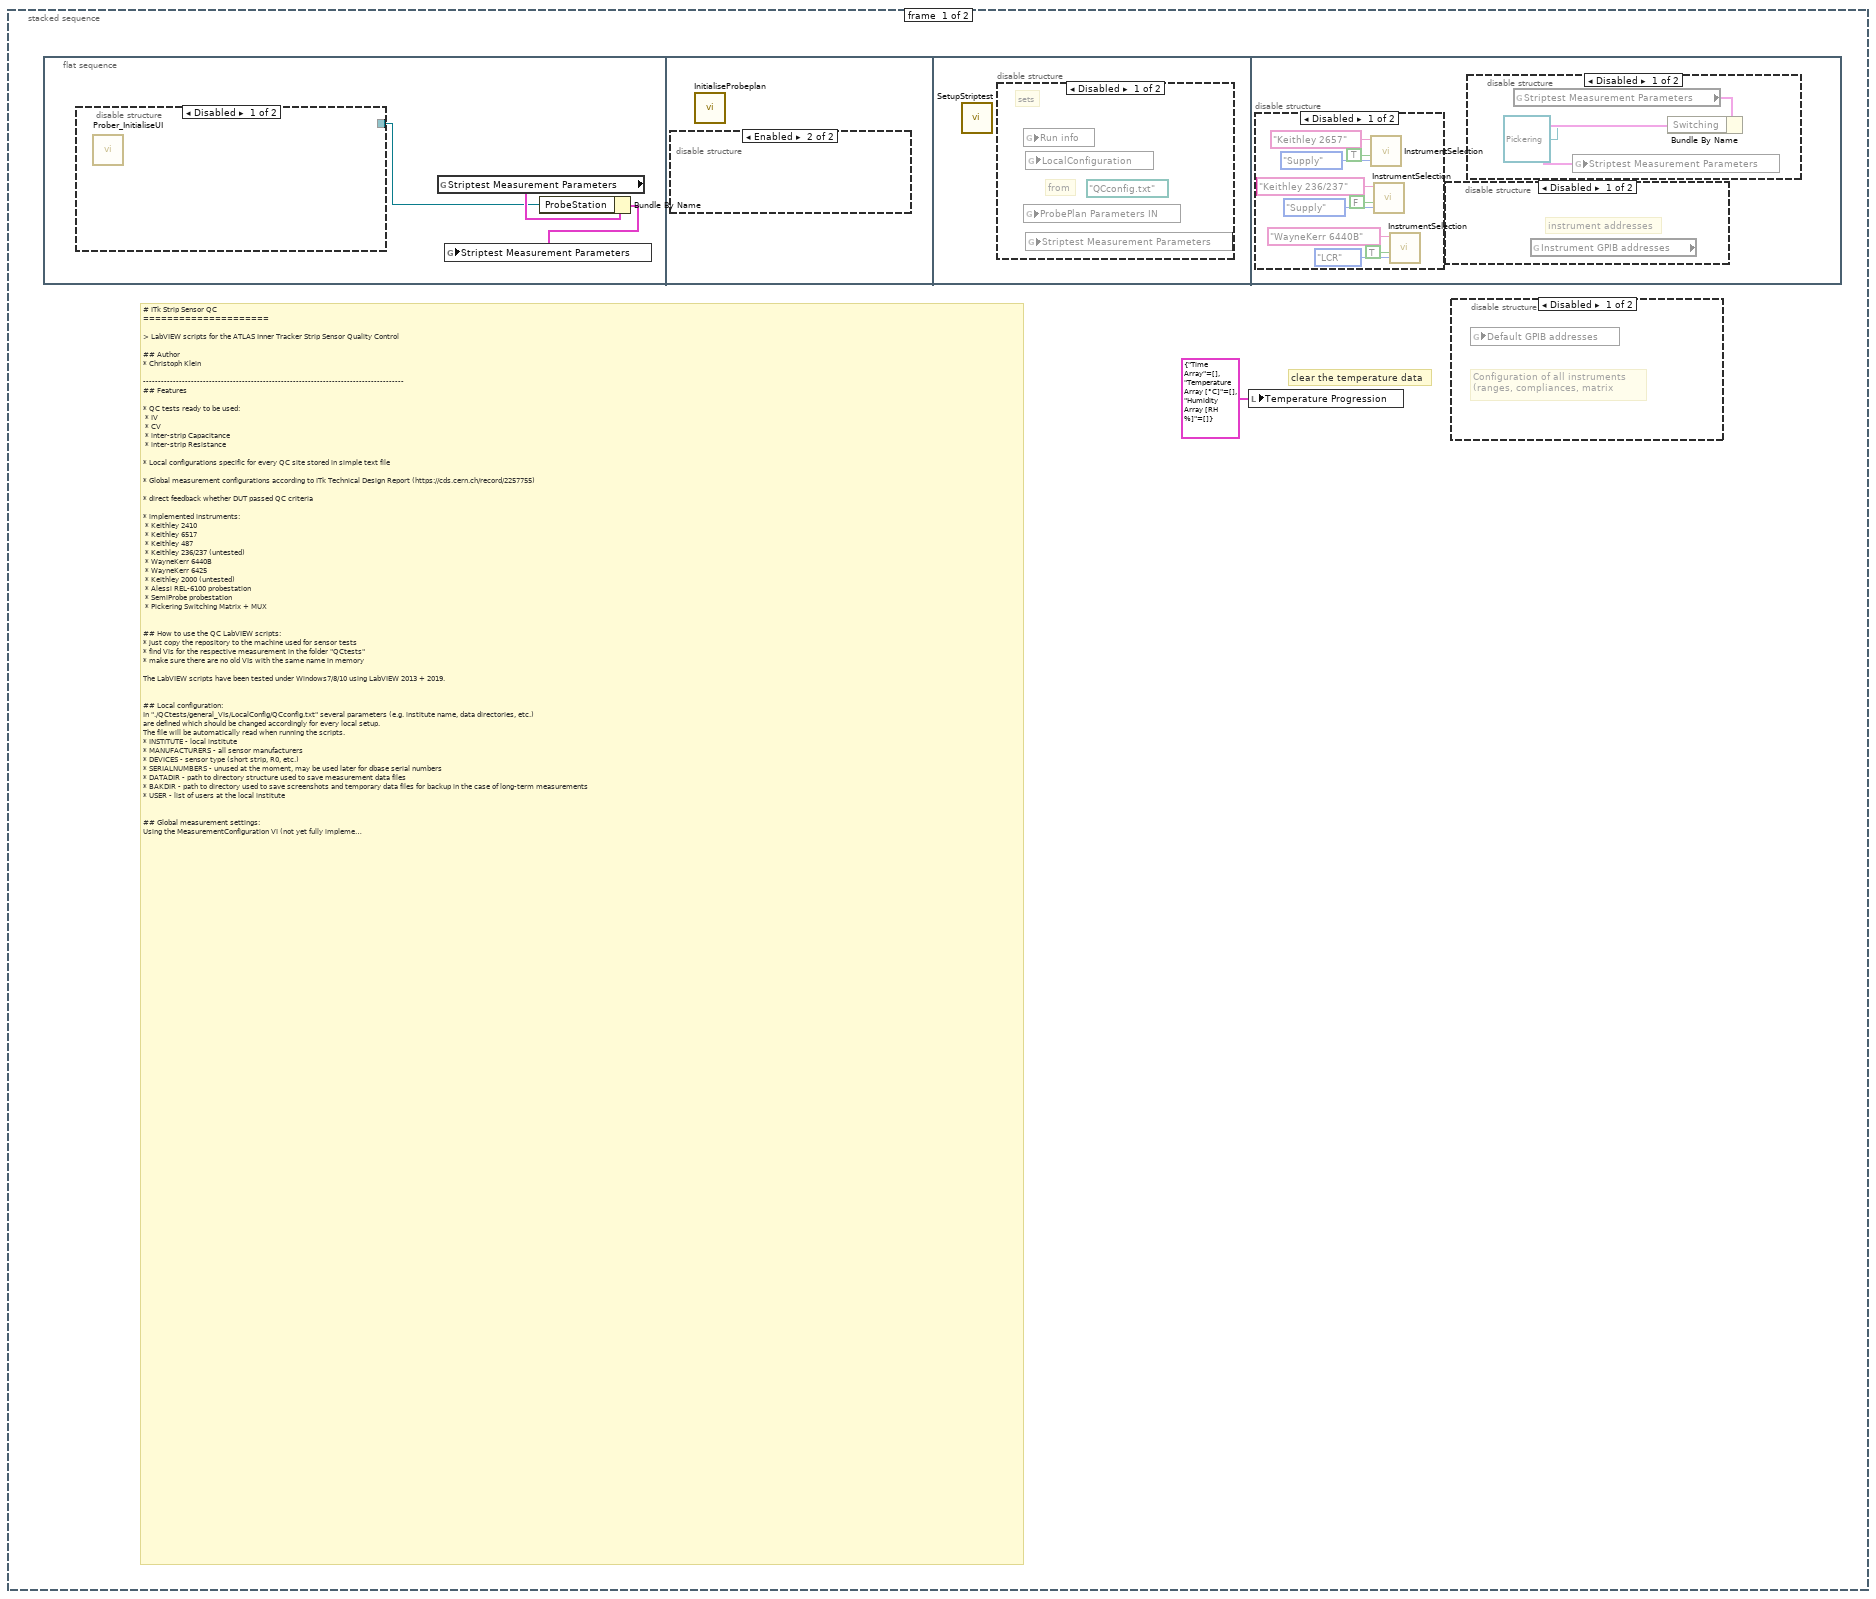
[diagram p2: hidden frame]
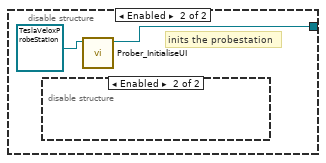
[diagram p4: hidden frame]
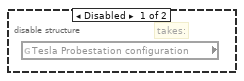
[diagram p5: hidden frame]
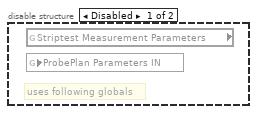
[diagram p6: hidden frame]
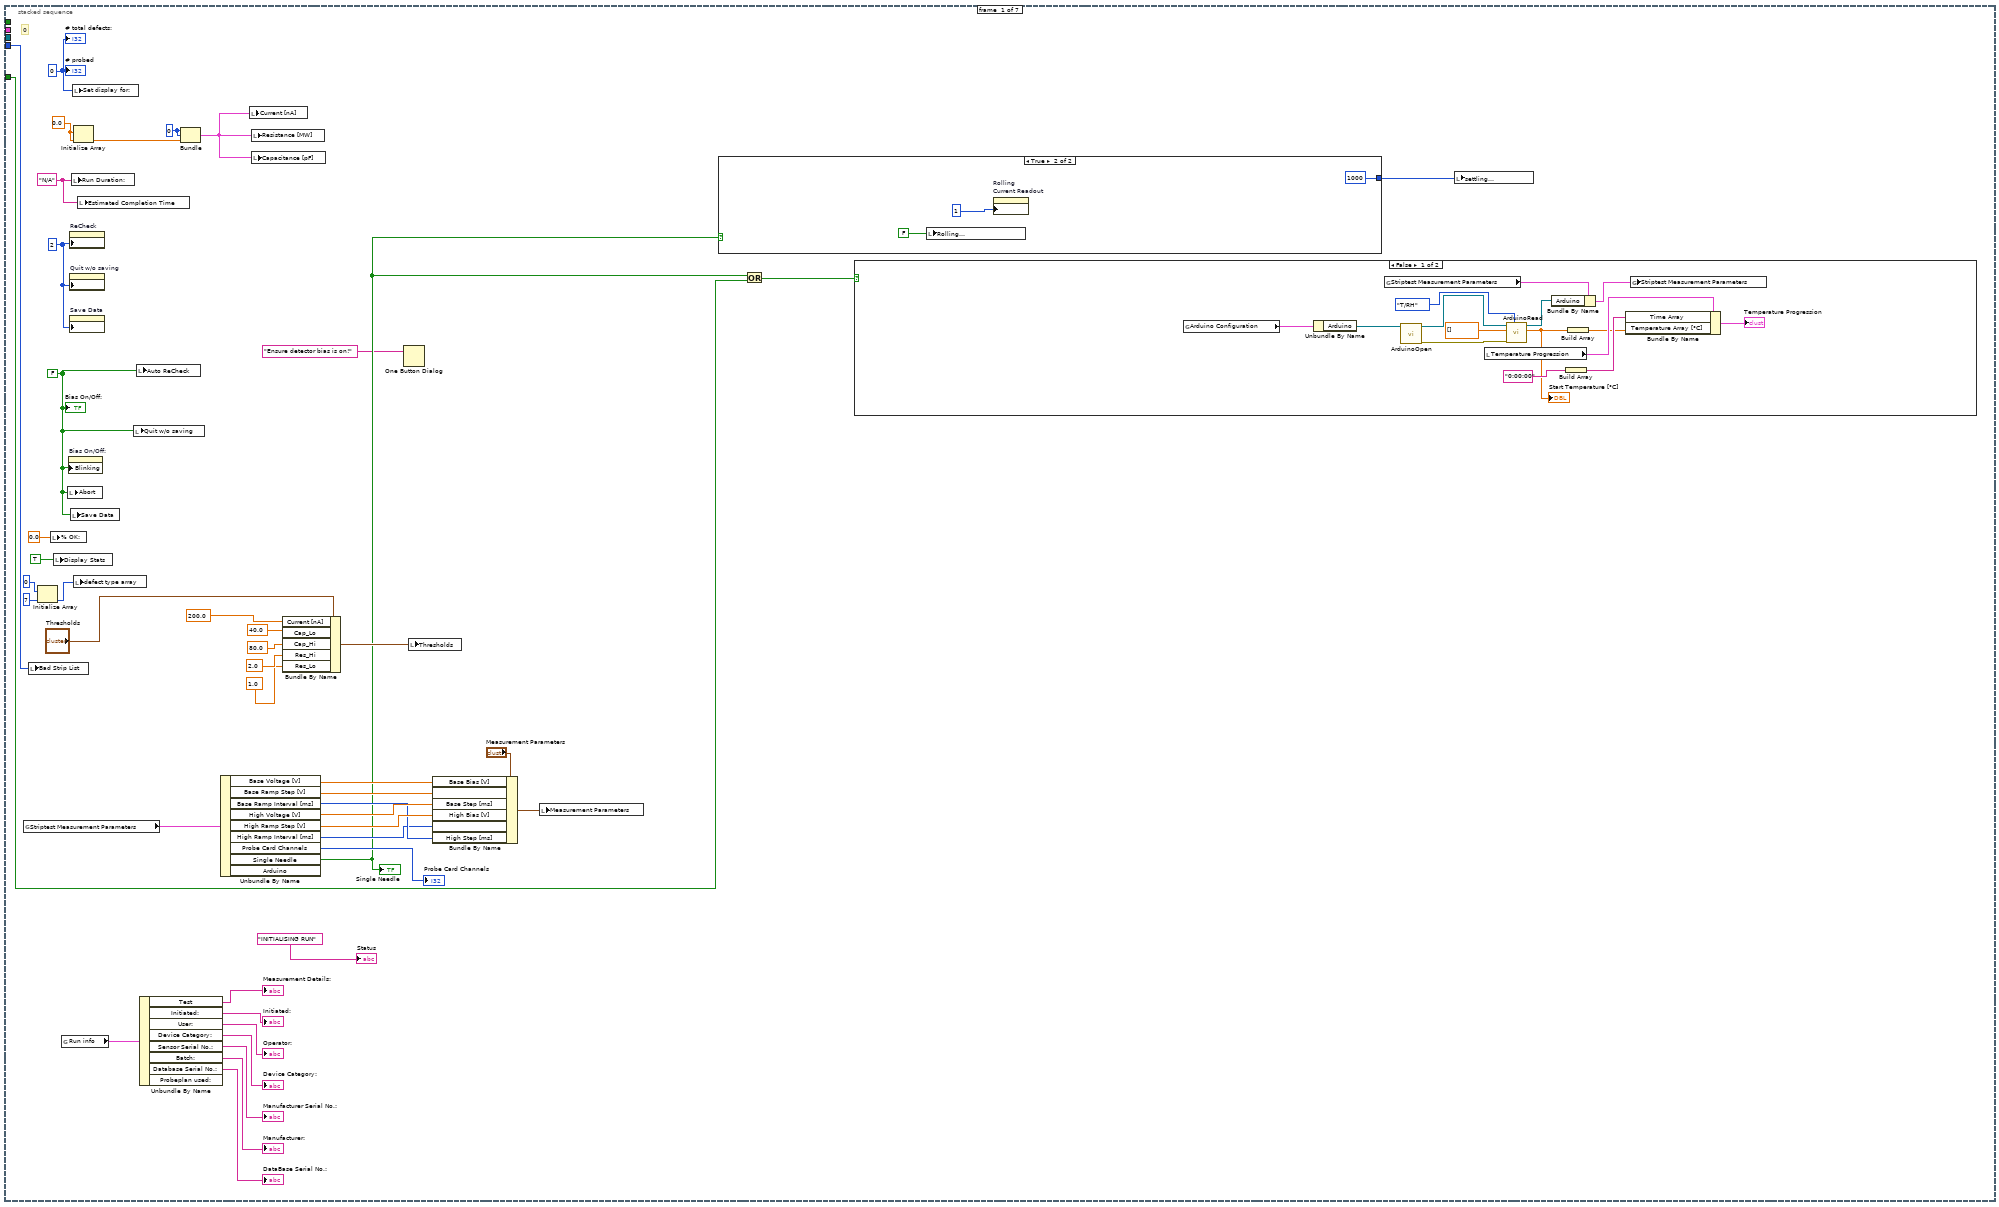
[diagram p11: hidden frame]
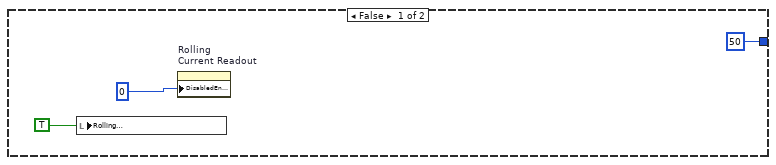
[diagram p12: hidden frame]
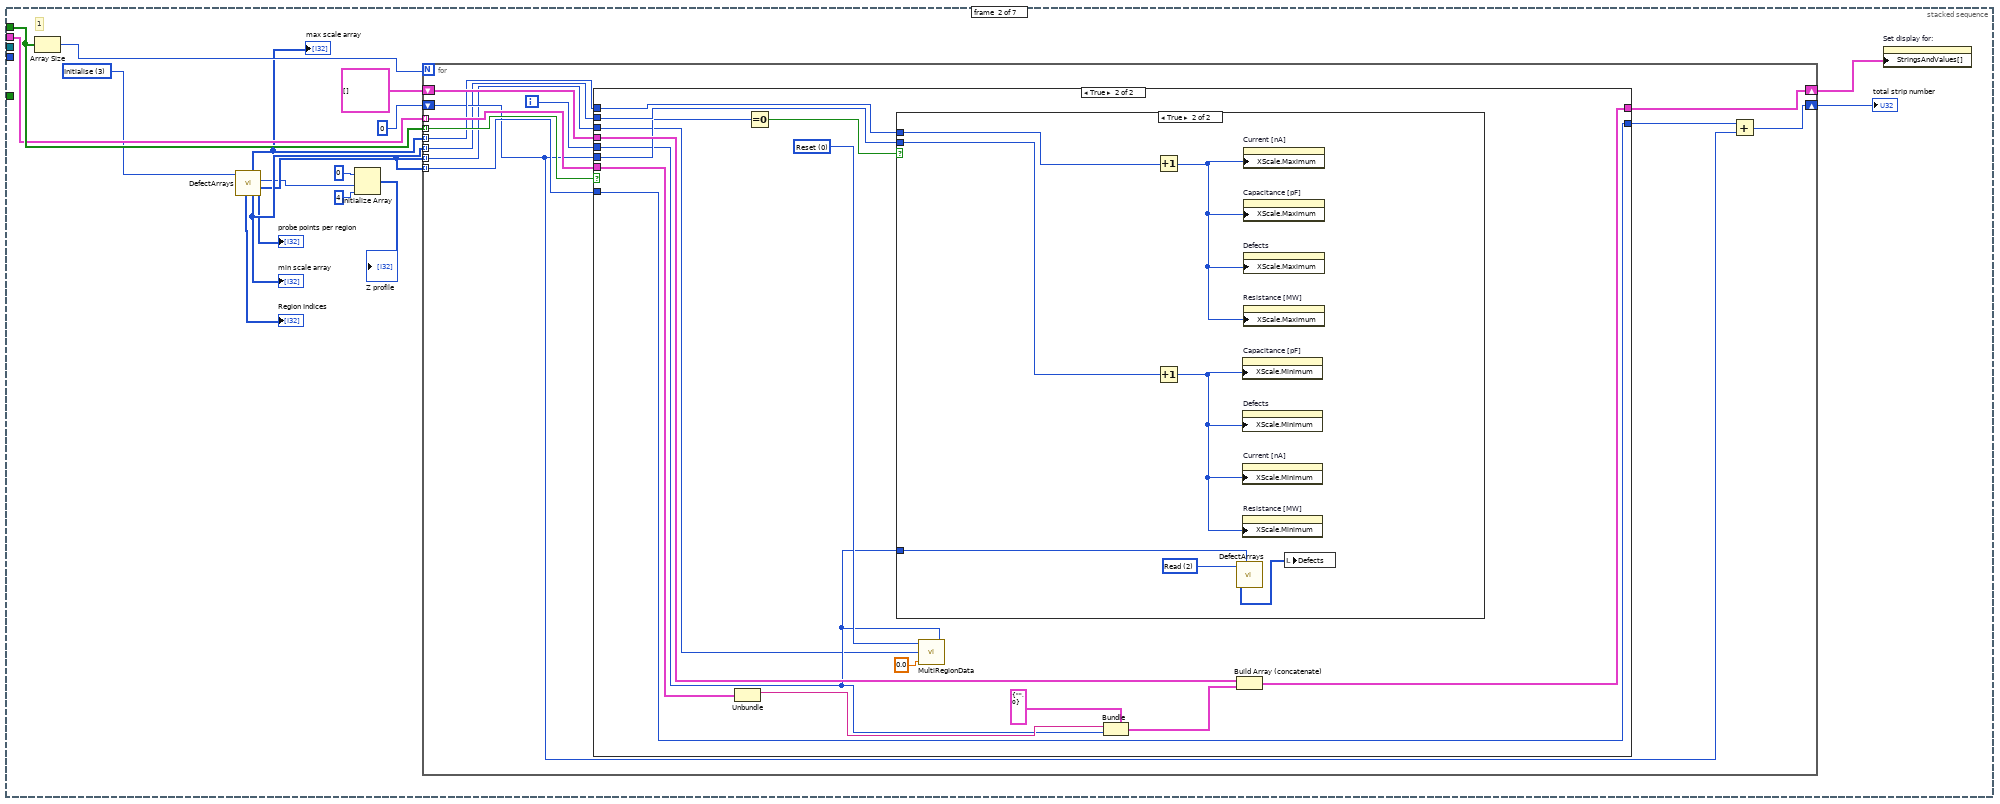
[diagram p14: hidden frame]
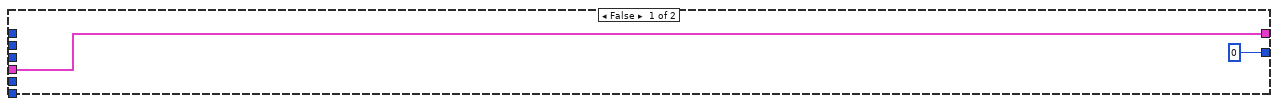
[diagram p15: hidden frame]
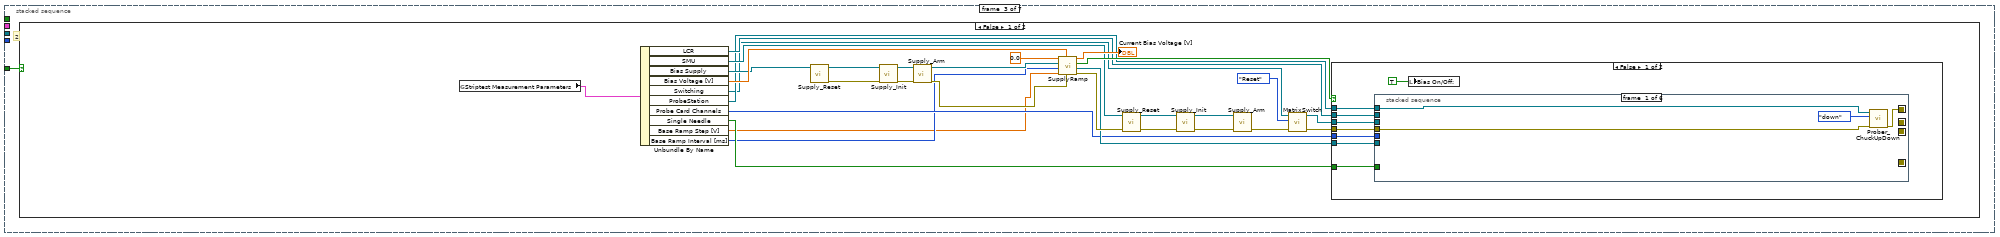
[diagram p17: hidden frame]
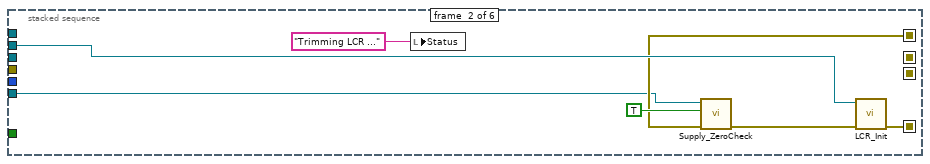
[diagram p18: hidden frame]
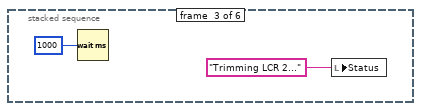
[diagram p19: hidden frame]
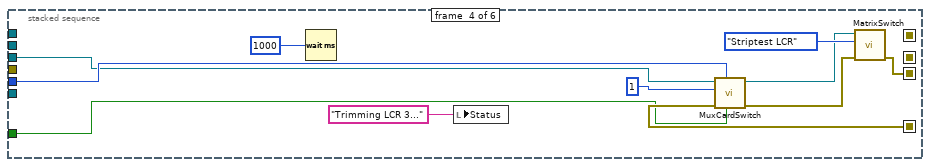
[diagram p20: hidden frame]
diagram:
  n1 = stacked-sequence {
    frame #0 {
      # "clear the temperature data"
      # "# ITk Strip Sensor QC\n=====================\n\n> LabVIEW scripts for the ATLAS Inner Tracker Strip Sensor Quality Control\n\n## Author\n*\tChristoph Klein\n\n---------------------------------------------------------------------------------------\n## Features\n\n*\tQC tests ready to be used: \n\t*\tIV\n\t*\tCV\n\t*\tinter-strip Capacitance\n\t*\tinter-strip Resistance\n\n*\tLocal configurations specific for every QC site stored in simple text file\n\n*\tGlobal measurement configurations according to ITk Technical Design Report (https://cds.cern.ch/record/2257755)\n\n*\tdirect feedback whether DUT passed QC criteria\n\n*\timplemented instruments:\n\t*\tKeithley 2410\n\t*\tKeithley 6517\n\t*\tKeithley 487\n\t*\tKeithley 236/237\t(untested)\n\t*\tWayneKerr 6440B\n\t*\tWayneKerr 6425\n\t*\tKeithley 2000\t(untested)\n\t*\tAlessi REL-6100 probestation\n\t*\tSemiProbe probestation\n\t*\tPickering Switching Matrix + MUX\n\t\n\n## How to use the QC LabVIEW scripts:\n*\tjust copy the repository to the machine used for sensor tests\n*\tfind VIs for the respective measurement in the folder \"QCtests\"\n*\tmake sure there are no old VIs with the same name in memory\n\nThe LabVIEW scripts have been tested under Windows7/8/10 using LabVIEW 2013 + 2019.\n\n\n## Local configuration:\nIn \"./QCtests/general_VIs/LocalConfig/QCconfig.txt\" several parameters (e.g. institute name, data directories, etc.) \nare defined which should be changed accordingly for every local setup.\nThe file will be automatically read when running the scripts.\n*\tINSTITUTE - local institute\n*\tMANUFACTURERS - all sensor manufacturers\n*\tDEVICES - sensor type (short strip, R0, etc.)\n*\tSERIALNUMBERS - unused at the moment, may be used later for dbase serial numbers\n*\tDATADIR - path to directory structure used to save measurement data files\n*\tBAKDIR - path to directory used to save screenshots and temporary data files for backup in the case of long-term measurements\n*\tUSER - list of users at the local institute\n\n\n## Global measurement settings:\nUsing the MeasurementConfiguration VI (not yet fully implemented) or the text files in \"./QCtests/general_VIs/globals/\" default measurement settings can be changed.\nHowever, do not alter crucial aspects of the measurement procedure during sensor QC unless approved or only if scripts are used for R&D purposes.\nWhen changing the default instrument, enter the name in the same way as in the list of implemented instruments above.\n\n## How to include new instrument types:\n*\topen \"InstrControl.lvproj\" from the \"InstrControl\" folder\n*\tcreate a new class (New -> Other Files -> Class) or copy an existing one (preferably of the same type as new instrument, e.g. supply) and \nthen add to the project (Right-click on existing class -> Save As... -> check \"add copy to InstrControl.lvproj\")\n*\tset inheritance appropriately (Right-click on new class -> Properties -> Inheritance)\n*\tadd/change VIs of new class and create global with instrument commands\n*\ttest that everything works properly (example test scripts available for most implemented intruments, just copy what has been done there)\n*\tadd instrument settings in global variable \"InstrControl.lvclass:InstrumentSetup.vi\"\n*\tadd case of new instrument in \"InstrControl.lvclass:InstrumentSelection.vi\"\n*\tadd tabs in \"HardwareConfiguration.vi\" and case in block diagram similar to existing instruments\n*\tmultiple instances of the same instrument (but with different GPIB addresses obviously) can be added by just creating an additional cluster with \ninstrument settings and add GPIB address in global \"InstrControl.lvclass:InstrumentSetup.vi\" + \nadding case in \"InstrControl.lvclass:InstrumentSelection.vi\"\n\n\n## Missing LabVIEW libraries in some versions\n*\tsome versions of LV do not have certain libraries included (anymore)\n*\tto date known issues arise for:\n\t*\tDDE communication protocol (needed for Alessi probestation)\n*\tcopies of missing libraries can be found in \"./InstrControl/additional LV libraries/\"\n*\tcopy files to\n\t*\tDDE: \"[LabVIEW version]/vi.lib/Platform/\""
      n2 = flat-sequence {
        frame #0 {
          n3 = disable-structure shown="Disabled" {
            disable-tunnel: [_ w5] -> w2
            frame Disabled {
              n4 = call-dynamic "Prober_InitialiseUI.vi"() -> ()  [unwired: 9 in, 3 out]
            }
            frame Enabled {
              # "inits the probestation"
              n5 = disable-structure shown="Enabled" {
                frame Disabled {
                  # "takes:"
                  n6 = global read "TeslaVelox_GlobalConfig.vi" "Tesla Probestation configuration"() -> ()  [unwired: 1 out]
                }
                frame Enabled {
                }
              }
              n7 = call-dynamic "Prober_InitialiseUI.vi"("TeslaVeloxProbeStation in"=refnum<class "TeslaVeloxProbeStation.lvclass"> refnum ("TeslaVeloxProbeStation.lvclass")) -> ("TeslaVeloxProbeStation out"=w5:refnum<class "TeslaVeloxProbeStation.lvclass">)  [unwired: 8 in, 2 out]
            }
          }
          n8 = global read "QC_MeasurementSetup.vi" "Striptest Measurement Parameters"() -> (w3:T9)
          n9 = Bundle By Name(cluster=w3, "ProbeStation"=w2) -> (w4:T9)
          n10 = global write "QC_MeasurementSetup.vi" "Striptest Measurement Parameters"(w4) -> ()
        }
        frame #1 {
          n11 = disable-structure shown="Enabled" {
            frame Disabled {
              # "uses following globals"
              n12 = global read "QC_MeasurementSetup.vi" "Striptest Measurement Parameters"() -> ()  [unwired: 1 out]
              n13 = global read "ProbePlanParams.vi" "ProbePlan Parameters IN"() -> ()  [unwired: 1 in]
            }
            frame Enabled {
            }
          }
          n14 = call "InitialiseProbeplan.vi"() -> ()  [unwired: 2 in]
        }
        frame #2 {
          n15 = call "SetupStriptest.vi"() -> ()  [unwired: 6 in, 1 out]
          n16 = disable-structure shown="Disabled" {
            frame Disabled {
              (unwired) path "QCconfig.txt"
              # "from"
              # "sets"
              n17 = global read "QC_RunInformation.vi" "Run info"() -> ()  [unwired: 1 in]
              n18 = global read "ProbePlanParams.vi" "ProbePlan Parameters IN"() -> ()  [unwired: 1 in]
              n19 = global read "QC_RunInformation.vi" "LocalConfiguration"() -> ()  [unwired: 1 in]
              n20 = global read "QC_MeasurementSetup.vi" "Striptest Measurement Parameters"() -> ()  [unwired: 1 in]
            }
            frame Enabled {
            }
          }
        }
        frame #3 {
          n21 = disable-structure shown="Disabled" {
            frame Disabled {
              n22 = call "InstrumentSelection.vi"("Verify GPIB address"=TRUE, "Instrument type"=T4."Supply", "Instrument name IN"="Keithley 2657") -> ()  [unwired: 3 in, 6 out]
              n23 = call "InstrumentSelection.vi"("Verify GPIB address"=FALSE, "Instrument type"=T4."Supply", "Instrument name IN"="Keithley 236/237") -> ()  [unwired: 3 in, 6 out]
              n24 = call "InstrumentSelection.vi"("Verify GPIB address"=TRUE, "Instrument type"=T4."LCR", "Instrument name IN"="WayneKerr 6440B") -> ()  [unwired: 3 in, 6 out]
            }
            frame Enabled {
            }
          }
          n25 = disable-structure shown="Disabled" {
            frame Disabled {
              # "instrument addresses"
              n26 = global read "InstrumentSetup.vi" "Instrument GPIB addresses"() -> ()  [unwired: 1 out]
            }
            frame Enabled {
            }
          }
          n27 = disable-structure shown="Disabled" {
            frame Disabled {
              n28 = global read "QC_MeasurementSetup.vi" "Striptest Measurement Parameters"() -> (w9:T9)
              n29 = Bundle By Name(cluster=w9, "Switching"=refnum<class "Pickering.lvclass"> refnum ("Pickering.lvclass")) -> (w8:T9)
              n30 = global write "QC_MeasurementSetup.vi" "Striptest Measurement Parameters"(w8) -> ()
            }
            frame Enabled {
            }
          }
        }
      }
      n31 = local write "Temperature Progression"(T3 {"Time Array"=[], "Temperature Array [°C]"=[], "Humidity Array [RH %]"=[]} ("Temperature Progression")) -> ()
      n32 = disable-structure shown="Disabled" {
        frame Disabled {
          # "Configuration of all instruments \n(ranges, compliances, matrix"
          n33 = global read "InstrumentSetup.vi" "Default GPIB addresses"() -> ()  [unwired: 1 in]
        }
        frame Enabled {
        }
      }
    }
    frame #1 {
      # "1"
      n34 = global read "QC_MeasurementSetup.vi" "Striptest Measurement Parameters"() -> (w19:T9)
      n35 = global read "ProbePlanParams.vi" "ProbePlan Parameters IN"() -> (w26:T10)
      n36 = Unbundle By Name(w26) -> ("Test ProbePoints.Regions Enabled"=w22:bool[], "ProbePlan array"=w21:T11)
      n37 = Unbundle By Name(w19) -> ("ProbeStation"=w20:refnum<class "ProbeStationControl.lvclass">)
      n38 = Initialize Array(0) -> (w24:i32[])  [unwired: 1 in]
      n39 = stacked-sequence {
        tunnel: w24 -> [w47 _ _ _ w262 _ _]
        tunnel: "Simulation?" -> [w41 _ w145 w240 _ w942 w1000]
        tunnel: w22 -> [_ w107 _ _ w265 _ w999]
        tunnel: w21 -> [_ w106 _ _ w263 _ _]
        tunnel: w20 -> [_ _ _ w238 _ w941 _]
        frame #0 {
          w49 = "N/A"
          w44 = FALSE
          w57 = 2
          w50 = 0
          w70 = 0
          w69 = 0.0
          # "0"
          n40 = global read "QC_MeasurementSetup.vi" "Striptest Measurement Parameters"() -> (w29:T9)
          n41 = local write "Bad Strip List"(w47) -> ()
          n42 = Initialize Array(0, 7 ("Dimension Size")) -> (w45:i32[])
          n43 = local write "% OK:"(0.0) -> ()
          n44 = local write "Display Stats"(TRUE) -> ()
          n45 = global read "QC_RunInformation.vi" "Run info"() -> (w67:T12)
          n46 = local write "Abort"(w44) -> ()
          n47 = property on="Bias On/Off:" class="Bool (strict)"("Blinking"=w44) -> ()  [unwired: 2 in, 2 out]
          n48 = property on="ReCheck" class="Bool"("DisabledEnum"=w57) -> ()  [unwired: 2 in, 2 out]
          n49 = property on="Quit w/o saving" class="Bool (strict)"("DisabledEnum"=w57) -> ()  [unwired: 2 in, 2 out]
          n50 = property on="Save Data" class="Bool (strict)"("DisabledEnum"=w57) -> ()  [unwired: 2 in, 2 out]
          n51 = local write "Save Data"(w44) -> ()
          n52 = local write "Run Duration:"(w49) -> ()
          n53 = local write "Set display for:"(w50) -> ()
          n54 = Initialize Array(w69, w69) -> (w71:dbl[])
          n55 = local write "defect type array"(w45) -> ()
          n56 = local write "Estimated Completion Time"(w49) -> ()
          n57 = local write "Quit w/o saving"(w44) -> ()
          n58 = local write "Auto ReCheck"(w44) -> ()
          n59 = Unbundle By Name(w67) -> ("Test"=→"Measurement Details:":string, "Initiated:"=→"Initiated:":string, "User:"=→"Operator:":string, "Device Category:"=→"Device Category:":string, "Sensor Serial No.:"=→"Manufacturer Serial No.:":string, "Batch:"=→"Manufacturer:":string, "Database Serial No.:"=→"DataBase Serial No.:":string)  [unwired: 1 out]
          n60 = Bundle(w70, w70, w71) -> (w68:cluster{i32, i32, dbl[]})  [unwired: 1 in]
          n61 = Unbundle By Name(w29) -> ("Base Voltage [V]"=w37:dbl, "Base Ramp Step [V]"=w38:dbl, "Base Ramp Interval [ms]"=w34:u32, "High Voltage [V]"=w35:dbl, "High Ramp Step [V]"=w36:dbl, "High Ramp Interval [ms]"=w33:u32, "Probe Card Channels"=→"Probe Card Channels":i32, "Single Needle"=w28:bool)  [unwired: 1 out]
          "Single Needle" <- w28
          n62 = local write "Current [nA]"(w68) -> ()
          n63 = local write "Resistance [MW]"(w68) -> ()
          n64 = local write "Capacitance [pF]"(w68) -> ()
          n65 = Bundle By Name(cluster="Thresholds", "Current [nA]"=200.0 ("CapLo"), "Cap_Lo"=40.0 ("CapLo"), "Cap_Hi"=80.0 ("CapHi"), "Res_Hi"=2.0 ("Rpolyhi"), "Res_Lo"=1.0 ("RpolyLo")) -> (w55:T1)
          n66 = One Button Dialog(message="Ensure detector bias is on!") -> ()  [unwired: 1 in, 1 out]
          n67 = local write "Thresholds"(w55) -> ()
          n68 = Bundle By Name(cluster="Measurement Parameters", "Base Bias [V]"=w37, "Base Ramp\n[V/step]"=w38, "Base Step [ms]"=w35, "High Bias [V]"=w36, "High Ramp\n[V/step]"=w33, "High Step [ms]"=w34) -> (w39:T2)
          n69 = local write "Measurement Parameters"(w39) -> ()
          n70 = case shown="True" w28 {
            tunnel: [50 1000] -> w30
            frame False {
              n71 = local write "Rolling\nCurrent Readout"(TRUE) -> ()
              n72 = property on="Rolling\nCurrent Readout" class="Bool (strict)"("DisabledEnum"=0) -> ()  [unwired: 2 in, 2 out]
            }
            frame True {
              n73 = local write "Rolling\nCurrent Readout"(FALSE) -> ()
              n74 = property on="Rolling\nCurrent Readout" class="Bool (strict)"("DisabledEnum"=1) -> ()  [unwired: 2 in, 2 out]
            }
          }
          n75 = Or(x=w28, y=w41) -> (x .or. y?=w40:bool)
          n76 = case shown="False" w40 {
            frame False {
              n77 = global read "InstrumentSetup.vi" "Arduino Configuration"() -> (w92:T13)
              n78 = Unbundle By Name(w92) -> ("Arduino"=w84:refnum<class "ArduinoControl.lvclass">)
              n79 = global read "QC_MeasurementSetup.vi" "Striptest Measurement Parameters"() -> (w80:T9)
              n80 = call "ArduinoOpen.vi"("ArduinoControl in"=w84) -> ("error out"=w82:errorcluster, "ArduinoControl out"=w83:refnum<class "ArduinoControl.lvclass">)  [unwired: 9 in]
              n81 = local read "Temperature Progression"() -> (w91:T3)
              n82 = call "ArduinoRead.vi"("Arduino function"=enum16{"T/RH", "Interlock", "Edgesense"}."T/RH", "error in (no error)"=w82, "Temperature IN"=dbl[] [], "ArduinoControl in"=w83) -> ("Temperature [°C]"=w86:dbl, "ArduinoControl out"=w78:refnum<class "ArduinoControl.lvclass">)  [unwired: 2 in, 4 out]
              "Start Temperature [°C]" <- w86
              n83 = Bundle By Name(cluster=w80, "Arduino"=w78) -> (w79:T9)
              n84 = Build Array("0:00:00") -> (w87:string[])
              n85 = Build Array(w86) -> (w85:dbl[])
              n86 = Bundle By Name(cluster=w91, "Time Array"=w87, "Temperature Array [°C]"=w85) -> (→"Temperature Progression":T3)
              n87 = global write "QC_MeasurementSetup.vi" "Striptest Measurement Parameters"(w79) -> ()
            }
            frame True {
            }
          }
          n88 = local write "settling\ndelay [ms]"(w30) -> ()
          "# total defects:" <- w50
          "# probed" <- w50
          "Status" <- "INITIALISING RUN"
          "Bias On/Off:" <- w44
        }
        frame #1 {
          w102 = u16 3 items=["Nothing", "Write", "Read", "Initialise"] ("action")
          # "1"
          n89 = Array Size(array=w107) -> (size(s)=w108:i32)
          n90 = call "DefectArrays.vi"("action"=w102) -> ("Region Indices"=→"Region Indices":i32[], "To"=w101:i32[], "max. No. of points in region"=w93:i32, "From"=w100:i32[], "No. of points in region"=w95:i32[])  [unwired: 2 in, 3 out]
          "max scale array" <- w101
          "min scale array" <- w100
          "probe points per region" <- w95
          n91 = Initialize Array(0, w93, 4) -> (→"Z profile":i32[][])
          n92 = for {
            N: w108 -> [_]
            tunnel: w107 -> [w120] mode=indexing
            shift-right: [w119] -> w105
            shift-left: cluster{string, i32}[] [] -> [w118]
            tunnel: w106 -> [w117] mode=indexing
            tunnel: w95 -> [w112] mode=indexing
            tunnel: w101 -> [w113] mode=indexing
            tunnel: w100 -> [w110] mode=indexing
            shift-right: [w114] -> w104
            shift-left: 0 -> [w111]
            tunnel: w95 -> [w109] mode=indexing
            i -> [w115]
            n93 = case shown="True" w120 {
              tunnel: w118 -> [w121 w136]
              tunnel: [w121 w135] -> w119
              tunnel: w117 -> [_ w137]
              tunnel: [0 w131] -> w116
              tunnel: w115 -> [_ w126]
              tunnel: w113 -> [_ w133]
              tunnel: w110 -> [_ w132]
              tunnel: w112 -> [_ w131]
              tunnel: w111 -> [_ w130]
              tunnel: w109 -> [_ w124]
              frame False {
              }
              frame True {
                w128 = u32 0 items=["Reset", "Read Array", "Read Element", "Write Element", "Write Array"] ("Action")
                n94 = Unbundle(w137) -> ("Region"=w127:string)  [unwired: 1 out]
                n95 = Equal To 0?(x=w130) -> (x = 0?=w134:bool)
                n96 = case shown="True" w134 {
                  tunnel: w133 -> [_ w139]
                  tunnel: w132 -> [_ w141]
                  tunnel: w126 -> [_ w142]
                  frame False {
                  }
                  frame True {
                    w144 = u16 2 items=["Nothing", "Write", "Read", "Initialise"] ("action")
                    n97 = Increment(x=w139) -> (x+1=w138:i32)
                    n98 = Increment(x=w141) -> (x+1=w140:i32)
                    n99 = call "DefectArrays.vi"("action"=w144, "Region Index"=w142) -> ("Defect array OUT"=w143:i32[][])  [unwired: 1 in, 7 out]
                    n100 = property on="Capacitance [pF]" class="WFGraph (strict)"("XScale.Minimum"=w140) -> ()  [unwired: 2 in, 2 out]
                    n101 = property on="Defects" class="IntGraph (strict)"("XScale.Minimum"=w140) -> ()  [unwired: 2 in, 2 out]
                    n102 = property on="Current [nA]" class="WFGraph (strict)"("XScale.Minimum"=w140) -> ()  [unwired: 2 in, 2 out]
                    n103 = property on="Resistance [MW]" class="WFGraph (strict)"("XScale.Minimum"=w140) -> ()  [unwired: 2 in, 2 out]
                    n104 = property on="Current [nA]" class="WFGraph (strict)"("XScale.Maximum"=w138) -> ()  [unwired: 2 in, 2 out]
                    n105 = property on="Capacitance [pF]" class="WFGraph (strict)"("XScale.Maximum"=w138) -> ()  [unwired: 2 in, 2 out]
                    n106 = property on="Defects" class="IntGraph (strict)"("XScale.Maximum"=w138) -> ()  [unwired: 2 in, 2 out]
                    n107 = property on="Resistance [MW]" class="WFGraph (strict)"("XScale.Maximum"=w138) -> ()  [unwired: 2 in, 2 out]
                    n108 = local write "Defects"(w143) -> ()
                  }
                }
                n109 = call "MultiRegionData.vi"("Action"=w128, "Array Size / Index"=w124, "Data IN"=0.0, "Region index"=w126) -> ()  [unwired: 2 in, 2 out]
                n110 = Bundle(cluster=cluster{string, i32} {"", 0}, w127, w126) -> (w125:cluster{string, i32})
                n111 = Build Array (concatenate)(w136, w125) -> (w135:cluster{string, i32}[])
              }
            }
            n112 = Add(x=w116, y=w111) -> (x+y=w114:i32)
          }
          "total strip number" <- w104
          n113 = property on="Set display for:" class="Ring (strict)"("StringsAndValues[]"=w105) -> ()  [unwired: 2 in, 2 out]
        }
        frame #2 {
          # "2"
          n114 = case shown="False" w145 {
            frame False {
              n115 = global read "QC_MeasurementSetup.vi" "Striptest Measurement Parameters"() -> (w174:T9)
              n116 = Unbundle By Name(w174) -> ("LCR"=w153:refnum<class "LCRControl.lvclass">, "SMU"=w154:refnum<class "SupplyControl.lvclass">, "Bias Supply"=w155:refnum<class "SupplyControl.lvclass">, "Bias Voltage [V]"=w165:dbl, "Switching"=w150:refnum<class "Switching.lvclass">, "ProbeStation"=w152:refnum<class "ProbeStationControl.lvclass">, "Probe Card Channels"=w149:i32, "Single Needle"=w148:bool, "Base Ramp Step [V]"=w146:dbl, "Base Ramp Interval [ms]"=w147:u32)
              n117 = call-dynamic "Supply_Reset.vi"("SupplyControl in"=w155) -> ("error out"=w169:errorcluster, "SupplyControl out"=w172:refnum<class "SupplyControl.lvclass">)  [unwired: 9 in]
              n118 = call-dynamic "Supply_Init.vi"("error in (no error)"=w169, "SupplyControl in"=w172) -> ("error out"=w170:errorcluster, "SupplyControl out"=w171:refnum<class "SupplyControl.lvclass">)  [unwired: 8 in]
              n119 = call-dynamic "Supply_Arm.vi"("error in (no error)"=w170, "SupplyControl in"=w171) -> ("error out"=w167:errorcluster, "SupplyControl out"=w168:refnum<class "SupplyControl.lvclass">)  [unwired: 8 in]
              n120 = call "SupplyRamp.vi"("error in"=w167, "Requested Voltage"=w165, "Step Size"=w146, "Step Delay"=w147, "Supply IN"=w168, "Starting Voltage"=0.0) -> ("error out"=w166:errorcluster, "Supply OUT"=w151:refnum<class "SupplyControl.lvclass">, "Compliance exceeded"=w159:bool, "Current Voltage"=→"Current Bias Voltage [V]":dbl)  [unwired: 2 in]
              n121 = call-dynamic "Supply_Reset.vi"("error in (no error)"=w166, "SupplyControl in"=w154) -> ("error out"=w163:errorcluster, "SupplyControl out"=w162:refnum<class "SupplyControl.lvclass">)  [unwired: 8 in]
              n122 = call-dynamic "Supply_Init.vi"("error in (no error)"=w163, "SupplyControl in"=w162) -> ("error out"=w164:errorcluster, "SupplyControl out"=w161:refnum<class "SupplyControl.lvclass">)  [unwired: 8 in]
              n123 = call-dynamic "Supply_Arm.vi"("error in (no error)"=w164, "SupplyControl in"=w161) -> ("error out"=w175:errorcluster)  [unwired: 8 in, 1 out]
              n124 = call-dynamic "MatrixSwitch.vi"("error in (no error)"=w175, "Action"=T5."Reset", "Switching in"=w150) -> ("error out"=w156:errorcluster, "Switching out"=w157:refnum<class "Switching.lvclass">)  [unwired: 6 in, 1 out]
              n125 = case shown="False" w159 {
                selector: w159 -> [_ w237]
                tunnel: w157 -> [w182 _]
                tunnel: w156 -> [w181 _]
                tunnel: w153 -> [w180 _]
                tunnel: w152 -> [w179 _]
                tunnel: w151 -> [w178 _]
                tunnel: w149 -> [w177 _]
                tunnel: w148 -> [w176 _]
                frame False {
                  n126 = stacked-sequence {
                    seq-local: [w185 _ _ _ _ _] -> [_ w190 _ _ _ _]
                    seq-local: [_ w194 _ _ _ _] -> [_ _ _ w202 _ _]
                    seq-local: [_ _ _ w203 _ _] -> [_ _ _ _ w211 _]
                    seq-local: [_ _ _ _ w209 _] -> [_ _ _ _ _ w217]
                    tunnel: w182 -> [_ _ _ w199 _ w218]
                    tunnel: w181 -> [w186 _ _ _ _ _]
                    tunnel: w180 -> [_ w193 _ _ w210 _]
                    tunnel: w179 -> [w184 _ _ _ _ _]
                    tunnel: w178 -> [_ w188 _ _ _ w219]
                    tunnel: w177 -> [_ _ _ w200 _ w214]
                    tunnel: w176 -> [_ _ _ w201 _ w213]
                    frame #0 {
                      n127 = call-dynamic "Prober_ChuckUpDown.vi"("error in (no error)"=w186, "Direction"=enum16{"up", "down"}."down", "ProbeStationControl in"=w184) -> ("error out"=w185:errorcluster)  [unwired: 6 in, 2 out]
                    }
                    frame #1 {
                      n128 = local write "Status"("Trimming LCR ..." ("STATUS 1")) -> ()
                      n129 = call-dynamic "Supply_ZeroCheck.vi"("error in (no error)"=w190, "enable/disable"=TRUE, "SupplyControl in"=w188) -> ("error out"=w189:errorcluster)  [unwired: 7 in, 1 out]
                      n130 = call-dynamic "LCR_Init.vi"("error in (no error)"=w189, "LCRControl in"=w193) -> ("error out"=w194:errorcluster)  [unwired: 8 in, 1 out]
                    }
                    frame #2 {
                      n131 = Wait (ms)(milliseconds to wait=u32 1000) -> ()  [unwired: 1 out]
                      n132 = local write "Status"("Trimming LCR 2..." ("STATUS 1")) -> ()
                    }
                    frame #3 {
                      n133 = Wait (ms)(milliseconds to wait=1000) -> ()  [unwired: 1 out]
                      n134 = local write "Status"("Trimming LCR 3..." ("STATUS 1")) -> ()
                      n135 = call-dynamic "MuxCardSwitch.vi"("Single Needle"=w201, "Probe Card Channels"=w200, "error in (no error)"=w202, "Switch to channel"=1, "Switching in"=w199) -> ("error out"=w204:errorcluster, "Switching out"=w198:refnum<class "Switching.lvclass">)  [unwired: 4 in, 1 out]
                      n136 = call-dynamic "MatrixSwitch.vi"("error in (no error)"=w204, "Action"=T5."Striptest LCR", "Switching in"=w198) -> ("error out"=w203:errorcluster)  [unwired: 6 in, 2 out]
                    }
                    frame #4 {
                      n137 = local write "Status"("Trimming LCR 4..." ("STATUS 1")) -> ()
                      n138 = call-dynamic "LCR_TrimOC.vi"("error in (no error)"=w211, "LCRControl in"=w210) -> ("error out"=w209:errorcluster)  [unwired: 8 in, 1 out]
                    }
                    frame #5 {
                      n139 = local write "Status"("Trimming LCR done" ("Status")) -> ()
                      n140 = call-dynamic "Supply_ZeroCheck.vi"("error in (no error)"=w217, "enable/disable"=TRUE, "SupplyControl in"=w219) -> ("error out"=w216:errorcluster)  [unwired: 7 in, 1 out]
                      n141 = disable-structure shown="Disabled" {
                        disable-tunnel: [w226 w234] -> w220
                        disable-tunnel: w218 -> [w225 w235]
                        disable-tunnel: w216 -> [w224 w234]
                        disable-tunnel: [w223 w235] -> w215
                        frame Disabled {
                          w229 = u16 0 items=["Open", "Close"] ("Switch action")
                          n142 = call-dynamic "MatrixSwitchSingle.vi"("Switch action"=w229, "error in (no error)"=w224, "Matrix Y"=1, "Matrix X"=3, "Switching in"=w225) -> ("error out"=w227:errorcluster, "Switching out"=w228:refnum<class "Switching.lvclass">)  [unwired: 4 in, 1 out]
                          n143 = call-dynamic "MatrixSwitchSingle.vi"("Switch action"=w229, "error in (no error)"=w227, "Matrix Y"=2, "Matrix X"=4, "Switching in"=w228) -> ("error out"=w226:errorcluster, "Switching out"=w223:refnum<class "Switching.lvclass">)  [unwired: 4 in, 1 out]
                        }
                        frame Enabled {
                        }
                      }
                      n144 = call-dynamic "MuxCardSwitch.vi"("Single Needle"=w213, "Probe Card Channels"=w214, "error in (no error)"=w220, "Switch to channel"=-1, "Switching in"=w215) -> ()  [unwired: 4 in, 3 out]
                    }
                  }
                  n145 = local write "Bias On/Off:"(TRUE ("Bias On?")) -> ()
                }
                frame True {
                  n146 = property on="Bias On/Off:" class="Bool (strict)"("Blinking"=w237) -> ()  [unwired: 2 in, 2 out]
                  n147 = local write "Status"("Compliance exceeded\nRUN ABORTED") -> ()
                }
              }
            }
            frame True {
            }
          }
        }
        frame #3 {
          # "3"
          n148 = property on="Bias On/Off:" class="Bool (strict)"() -> ("Blinking"=w239:bool)  [unwired: 2 in, 2 out]
          n149 = case shown="False" w239 {
            tunnel: w240 -> [w244 _]
            tunnel: w238 -> [w241 _]
            frame False {
              w245 = 0
              n150 = property on="Abort" class="Bool (strict)"("DisabledEnum"=w245) -> ()  [unwired: 2 in, 2 out]
              n151 = local read "Single Needle"() -> (w243:bool)
              n152 = property on="Auto ReCheck" class="Bool (strict)"("DisabledEnum"=w245) -> ()  [unwired: 2 in, 2 out]
              n153 = Or(x=w243, y=w244) -> (x .or. y?=w242:bool)
              n154 = case shown="False" w242 {
                tunnel: [w248 FALSE] -> w246
                tunnel: w241 -> [w247 _]
                frame False {
                  n155 = stacked-sequence {
                    tunnel: [_ w257] -> w248
                    tunnel: w247 -> [_ _]
                    frame #0 {
                      n156 = global read "QC_MeasurementSetup.vi" "Striptest Measurement Parameters"() -> (w249:T9)
                      n157 = local write "Status"("Reference measurement") -> ()
                      n158 = Unbundle By Name(w249) -> ("Switching"=w250:refnum<class "Switching.lvclass">)
                      n159 = call-dynamic "MatrixSwitch.vi"("Action"=T5."Striptest SMU", "Switching in"=w250) -> ()  [unwired: 7 in, 3 out]
                    }
                    frame #1 {
                      # "Controls the MUX!"
                      n160 = local read "settling\ndelay [ms]"() -> (w256:i32)
                      n161 = call "CurrentCorrection.vi"("Action"=T6."Reference measurement", "settling\ndelay"=w256) -> ("Compliance exceeded?"=w257:bool, "Current Reference 100V"=→"Current Reference 100V":dbl[], "Current Reference 10V"=→"Current Reference 10V":dbl[])  [unwired: 3 in, 2 out]
                    }
                  }
                }
                frame True {
                }
              }
              n162 = case shown="False" w246 {
                frame False {
                  n163 = local write "Status"("RUN IN PROGRESS" ("STATUS 1")) -> ()
                }
                frame True {
                  n164 = property on="Bias On/Off:" class="Bool (strict)"("Blinking"=TRUE ("Compliance?")) -> ()  [unwired: 2 in, 2 out]
                  n165 = local write "Status"("Compliance exceeded\nRUN ABORTED") -> ()
                }
              }
            }
            frame True {
            }
          }
        }
        frame #4 {
          # "4-measure"
          n166 = property on="Bias On/Off:" class="Bool (strict)"() -> ("Blinking"=w264:bool)  [unwired: 2 in, 2 out]
          n167 = case shown="False" w264 {
            tunnel: w265 -> [w275 _]
            tunnel: w263 -> [w274 _]
            tunnel: w262 -> [w273 _]
            frame False {
              w269 = 0  # # of probed  channels?
              n168 = local read "Temperature Progression"() -> (w267:T3)
              n169 = local read "probe points per region"() -> (w268:i32[])
              n170 = Array Size(array=w275) -> (size(s)=w276:i32)
              n171 = local read "max scale array"() -> (w271:i32[])
              n172 = local read "min scale array"() -> (w270:i32[])
              n173 = for {
                N: w276 -> [_]
                tunnel: w275 -> [w289] mode=indexing
                tunnel: w274 -> [w288] mode=indexing
                tunnel: w273 -> [w287]
                shift-right: [w281] -> _
                shift-left: 0 -> [w286]
                tunnel: w271 -> [w284] mode=indexing
                tunnel: w270 -> [w285] mode=indexing
                shift-right: [w280] -> _
                shift-left: w269 -> [w282]
                tunnel: w268 -> [w279] mode=indexing
                shift-right: [w277] -> w266
                shift-left: w267 -> [w278]
                i -> [w283]
                # "Strip region loop"
                n174 = case shown="True" w289 {
                  tunnel: w288 -> [_ w305]
                  tunnel: w287 -> [_ _]
                  tunnel: w286 -> [w291 w306]
                  tunnel: w285 -> [_ w301]
                  tunnel: w284 -> [_ w298]
                  tunnel: w283 -> [_ w303]
                  tunnel: w282 -> [w293 w300]
                  tunnel: [w290 w299] -> w281
                  tunnel: [w293 w297] -> w280
                  tunnel: w279 -> [_ w296]
                  tunnel: w278 -> [w292 w295]
                  tunnel: [w292 w294] -> w277
                  frame False {
                    # "Region disabled"
                    n175 = Increment(x=w291) -> (x+1=w290:i32)
                  }
                  frame True {
                    # "region enabld"
                    n176 = Unbundle By Name(w305) -> ("Region"=→"Probing Region:":string, "ProbePoints"=w302:T14)
                    n177 = local write "Set display for:"(w306) -> ()
                    n178 = while {
                      tunnel: w303 -> [w307]
                      tunnel: w302 -> [w327]
                      shift-right: [w320] -> _
                      shift-left: w301 -> [w309]
                      shift-right: [w321] -> w297
                      shift-left: w300 -> [w322]
                      tunnel: w298 -> [w319]
                      tunnel: w296 -> [_]
                      shift-right: [w317] -> w294
                      shift-left: w295 -> [w318]
                      i -> [w323]
                      stop <- w326 stop-if-true
                      # "strip loop"
                      n179 = local read "Abort"() -> (w312:bool)
                      n180 = property on="Bias On/Off:" class="Bool (strict)"() -> ("Blinking"=w316:bool)  [unwired: 2 in, 2 out]
                      n181 = Equal To 0?(x=w322) -> (x = 0?=w329:bool)
                      n182 = Equal?(x=w309, y=w319) -> (x = y?=w308:bool)
                      n183 = Index Array(array=w327, index=w309) -> (element=w328:T15)
                      n184 = Not(x=w316) -> (.not. x?=w315:bool)
                      n185 = Not(x=w312) -> (.not. x?=w311:bool)
                      n186 = case shown="True" w329 {
                        frame False {
                        }
                        frame True {
                          n187 = local read "Probe Card Channels"() -> (w938:i32)
                          n188 = local read "total strip number"() -> (w939:u32)
                          n189 = Divide(x=w939, y=w938) -> (x/y=w937:dbl)
                          n190 = To Long Integer(number=w937) -> (32bit integer=w936:i32)
                          n191 = call "RunTime.vi"("no. measurements"=w936, "Flag"=1) -> ()  [unwired: 2 in, 4 out]
                        }
                      }
                      n192 = case shown="True" w308 {
                        tunnel: w307 -> [_ w330]
                        frame False {
                        }
                        frame True {
                          n193 = stacked-sequence {
                            tunnel: w330 -> [_ w333 w339]
                            frame #0 {
                              n194 = Wait (ms)(milliseconds to wait=100) -> ()  [unwired: 1 out]
                            }
                            frame #1 {
                              n195 = Increment(x=w333) -> (x+1=w336:i32)
                              n196 = Multiply(x=w336, y=111) -> (x*y=w334:i32)
                              n197 = call "SaveJPEG.vi"("Picture No."=w334, "Test"="Striptest") -> ()  [unwired: 1 in, 2 out]
                            }
                            frame #2 {
                              n198 = local read "probe points per region"() -> (w343:i32[])
                              n199 = Index Array(array=w343, index=w339) -> (element=w340:i32)
                              n200 = local read "Probing Region:"() -> (w338:string)
                              n201 = call "SaveStriptestRecoveryFiles.vi"("Arrays format"="%016.6f", "Array Titles"="ProbeplanIndex Current PinholeFlag Capacitance Resistance", "Strip Segment"=w338, "no. of arrays"=5, "Actual array lengths"=w340, "Region #"=w339) -> ()  [unwired: 2 out]
                            }
                          }
                        }
                      }
                      n202 = Unbundle By Name(w328) -> ("CardViable?"=w314:bool)
                      n203 = property on="Bias On/Off:" class="Bool (strict)"() -> ("Blinking"=w324:bool)  [unwired: 2 in, 2 out]
                      n204 = Compound Arithmetic op=AND(w314, w315, w311) -> (w313:bool)
                      n205 = case shown="True" w313 {
                        tunnel: w307 -> [_ w362]
                        tunnel: w327 -> [_ w361]
                        tunnel: w309 -> [w344 w356]
                        tunnel: w323 -> [_ w360]
                        tunnel: w322 -> [w347 w359]
                        tunnel: [w347 w358] -> w321
                        tunnel: [w345 w357] -> w320
                        tunnel: w318 -> [w346 w355]
                        tunnel: [w346 w354] -> w317
                        frame False {
                          n206 = Increment(x=w344) -> (x+1=w345:i32)
                        }
                        frame True {
                          n207 = global read "QC_MeasurementSetup.vi" "Striptest Measurement Parameters"() -> (w349:T9)
                          n208 = Unbundle By Name(w349) -> ("ProbeStation"=w352:refnum<class "ProbeStationControl.lvclass">, "Switching"=w353:refnum<class "Switching.lvclass">, "Temperature Readout"=w350:enum16{"Read Arduino", "Enter manually"}, "Arduino"=w351:refnum<class "ArduinoControl.lvclass">, "Pinholes Y/N"=w348:bool)
                          n209 = stacked-sequence {
                            tunnel: w362 -> [w377 w659 w780 w896 _]
                            tunnel: w361 -> [w366 _ _ _ _]
                            tunnel: w356 -> [w365 _ _ _ w923]
                            tunnel: w359 -> [_ _ _ _ w934]
                            tunnel: w360 -> [w363 w657 w781 w895 w921]
                            tunnel: [_ _ _ _ w924] -> w358
                            tunnel: [_ _ _ _ w933] -> w357
                            tunnel: w355 -> [_ w664 _ _ _]
                            tunnel: [_ w661 _ _ _] -> w354
                            tunnel: w353 -> [_ w665 w785 _ _]
                            tunnel: w352 -> [w364 _ _ _ _]
                            tunnel: w351 -> [_ w662 _ _ _]
                            tunnel: w350 -> [_ w663 _ _ _]
                            tunnel: w348 -> [_ w651 w776 _ _]
                            frame #0 {
                              w376 = u32 4 items=["Reset", "Read Array", "Read Element", "Write Element", "Write Array"] ("Action")
                              # "move to strip"
                              n210 = Index Array(array=w366, index=w365) -> (element=w384:T15)
                              n211 = local write "disabled channels"(i32[] []) -> ()
                              n212 = Unbundle(w384) -> ("Label"=w380:string)  [unwired: 3 out]
                              "Probe Point:" <- w380
                              n213 = local read "Simulation?"() -> (w370:bool)
                              n214 = local read "Abort"() -> (w372:bool)
                              n215 = Format Into String(format string="Moving to %s", w380) -> (resulting string=w383:string)  [unwired: 2 in, 1 out]
                              n216 = local write "Status"(w383) -> ()
                              n217 = local read "Probe Card Channels"() -> (w373:i32)
                              n218 = xnode "Match Regular Expression"("input string"=w380, "regular expression"="(Strip|Channel)\\s+(\\d+)", "ignore case? (F)"=TRUE) -> ("submatch 2"=w369:string)  [unwired: 3 in, 6 out]
                              n219 = Or(x=w372, y=w370) -> (x .or. y?=w371:bool)
                              n220 = Empty String/Path?(string/path=w369) -> (empty?=w368:bool)
                              n221 = Not(x=w368) -> (.not. x?=w367:bool)
                              n222 = case shown="False" w371 {
                                tunnel: w377 -> [w643 _]
                                tunnel: w365 -> [w644 _]
                                tunnel: w373 -> [w645 _]
                                tunnel: w364 -> [w641 _]
                                frame False {
                                # "Move to Strip"
                                n223 = local read "Single Needle"() -> (w647:bool)
                                n224 = call "MoveToStrip.vi"("Single Needle"=w647, "Strip No."=w644, "Region"=w643, "ProbeStationControl in"=w641) -> ("Z [µm]"=w642:i32)  [unwired: 5 in, 2 out]
                                n225 = local read "Z profile"() -> (w650:i32[][])
                                n226 = Initialize Array(w642, w645, 1) -> (w648:i32[][])
                                n227 = Replace Array Subset(array=w650, new element=w648, index (row)=w644, index (col)=w643) -> (w649:i32[][])
                                n228 = local write "Z profile"(w649) -> ()
                                }
                                frame True {
                                }
                              }
                              n229 = case shown="True" w367 {
                                tunnel: [w386 w396] -> w378
                                tunnel: w365 -> [w388 w394]
                                tunnel: w373 -> [w387 w395]
                                tunnel: w366 -> [_ w393]
                                frame False {
                                n230 = for {
                                N: w387 -> [_]
                                tunnel: w388 -> [w391]
                                tunnel: [w389] -> w386 mode=indexing
                                i -> [w392]
                                # "Actually use the probepoint\nindex"
                                n231 = Add(x=w391, y=w392) -> (x+y=w390:i32)
                                n232 = Increment(x=w390) -> (x+1=w389:i32)
                                }
                                }
                                frame True {
                                # "If probepoint label defined as Strip or Channel, use\nthat as the channel number in the data array."
                                n233 = for {
                                N: w395 -> [_]
                                tunnel: [w405] -> w396 mode=indexing
                                tunnel: w394 -> [w402]
                                tunnel: w393 -> [w400]
                                i -> [w403]
                                n234 = Add(x=w402, y=w403) -> (x+y=w401:i32)
                                n235 = Index Array(array=w400, index=w401) -> (element=w399:T15)
                                n236 = Unbundle By Name(w399) -> ("Label"=w398:string)
                                n237 = xnode "Match Regular Expression"("input string"=w398, "regular expression"="(Strip|Channel)\\s+(\\d+)") -> ("submatch 2"=w397:string)  [unwired: 4 in, 6 out]
                                n238 = Scan From String(format string="%d", input string=w397) -> (output 1=w405:i32)  [unwired: 3 in, 3 out]
                                }
                                }
                              }
                              n239 = To Double Precision Float(number=w378) -> (double precision float=w374:dbl[])
                              n240 = call "MultiRegionData.vi"("Action"=w376, "Array No."=0 ("Array Size / Index"), "Array Size / Index"=w363, "Array IN"=w374, "Region index"=w377) -> ()  [unwired: 1 in, 2 out]
                            }
                            frame #1 {
                              # "Pinholes"
                              n241 = local read "Simulation?"() -> (w666:bool)
                              n242 = flat-sequence {
                                tunnel: w664 -> [w734]
                                tunnel: w663 -> [w731]
                                tunnel: w662 -> [w730]
                                tunnel: [w729] -> w661
                                tunnel: w659 -> [w726]
                                tunnel: w657 -> [w725]
                                frame #0 {
                                # "read temperature"
                                n243 = Unbundle By Name(w734) -> ("Time Array"=w735:string[], "Temperature Array [°C]"=w738:dbl[], "Humidity Array [RH %]"=w739:dbl[])
                                n244 = case shown="\"Read Arduino\"" w731 {
                                tunnel: w730 -> [w758 _]
                                tunnel: [w757 _] -> _
                                tunnel: w738 -> [w755 w771]
                                tunnel: w739 -> [w756 w772]
                                tunnel: [w754 w770] -> w740
                                tunnel: [w753 w769] -> w741
                                tunnel: [w752 _] -> w728
                                tunnel: [w751 _] -> w727
                                frame "Read Arduino" {
                                n245 = for {
                                N: 3 -> [_]
                                tunnel: enum16{"T/RH", "Interlock", "Edgesense"}."T/RH" ("Arduino function") -> [w767]
                                tunnel: w758 -> [w766]
                                tunnel: [w765] -> w757
                                tunnel: [w763] -> w752
                                tunnel: [w764] -> w751
                                stop <- w760 continue-if-true
                                # "retry"
                                n246 = call "ArduinoRead.vi"("Arduino function"=w767, "ArduinoControl in"=w766) -> ("error out"=w765:errorcluster, "rel. Humidity [%]"=w764:dbl, "Temperature [°C]"=w763:dbl)  [unwired: 4 in, 3 out]
                                n247 = Absolute Value(x=w763) -> (abs(x)=w762:dbl)
                                n248 = Less?(x=w762, y=0.1) -> (x < y?=w760:bool)
                                }
                                n249 = Build Array (concatenate)(w755, w752) -> (w754:dbl[])
                                n250 = Build Array (concatenate)(w756, w751) -> (w753:dbl[])
                                }
                                frame "Enter manually", Default {
                                n251 = Index Array(array=w771, index=0) -> (element=w768:dbl)
                                n252 = Index Array(array=w772, index=0) -> (element=w773:dbl)
                                n253 = Build Array (concatenate)(w771, w768) -> (w770:dbl[])
                                n254 = Build Array (concatenate)(w772, w773) -> (w769:dbl[])
                                }
                                }
                                "Temp [°C]" <- w728
                                "RH [%]" <- w727
                                n255 = call "RunTime.vi"("Probing done - new estimation"=FALSE, "Flag"=0) -> ("Time so far"=w736:string)  [unwired: 2 in, 3 out]
                                n256 = Build Array (concatenate)(w735, w736) -> (w737:string[])
                                n257 = Bundle By Name(cluster=w734, "Time Array"=w737, "Temperature Array [°C]"=w740, "Humidity Array [RH %]"=w741) -> (w729:T3)
                                n258 = disable-structure shown="Enabled" {
                                disable-tunnel: w728 -> [w747 _]
                                disable-tunnel: w727 -> [w744 _]
                                disable-tunnel: w726 -> [w743 _]
                                disable-tunnel: w725 -> [w742 _]
                                frame Enabled {
                                n259 = call "MultiRegionData.vi"("Action"=T7."Write Element", "Array No."=u32 6, "Array Size / Index"=w742, "Data IN"=w747, "Region index"=w743) -> ()  [unwired: 1 in, 2 out]
                                n260 = call "MultiRegionData.vi"("Action"=T7."Write Element", "Array No."=u32 7, "Array Size / Index"=w742, "Data IN"=w744, "Region index"=w743) -> ()  [unwired: 1 in, 2 out]
                                }
                                frame Disabled {
                                }
                                }
                                }
                              }
                              n261 = case shown="True" w651 {
                                tunnel: w666 -> [_ w670]
                                tunnel: w665 -> [_ w669]
                                tunnel: w659 -> [_ w668]
                                tunnel: w657 -> [_ w667]
                                frame False {
                                }
                                frame True {
                                n262 = stacked-sequence {
                                tunnel: w670 -> [w672 w675]
                                tunnel: w668 -> [_ w677]
                                tunnel: w667 -> [_ w676]
                                tunnel: w669 -> [w671 _]
                                frame #0 {
                                n263 = case shown="False" w672 {
                                tunnel: w671 -> [w673 _]
                                frame False {
                                w674 = u16 2 items=["Reset", "Ground", "Striptest IV", "Striptest LCR", "IV", "CV", "Interstrip Cap", "Interstrip Res"] ("Action")
                                # "Switch the Matrix to pinhole config"
                                # "not in simulation"
                                n264 = call-dynamic "MatrixSwitch.vi"("Action"=w674, "Switching in"=w673) -> ()  [unwired: 7 in, 3 out]
                                }
                                frame True {
                                }
                                }
                                }
                                frame #1 {
                                n265 = local read "Abort"() -> (w678:bool)
                                n266 = case shown="False" w678 {
                                tunnel: w677 -> [w688 _]
                                tunnel: w676 -> [w687 _]
                                tunnel: w675 -> [w679 _]
                                frame False {
                                w684 = u32 4 items=["Reset", "Read Array", "Read Element", "Write Element", "Write Array"] ("Action")
                                w685 = u32 4 items=["Reset", "Read Array", "Read Element", "Write Element", "Write Array"] ("Action")
                                n267 = case shown="False" w679 {
                                tunnel: [w700 w713] -> w680
                                tunnel: [w697 w712] -> w686
                                frame False {
                                n268 = local read "Thresholds"() -> (w699:T1)
                                n269 = Unbundle By Name(w699) -> ("Current [nA]"=w698:dbl)
                                n270 = case shown="True" "Rolling\nCurrent Readout" {
                                tunnel: [w705 w707] -> w700
                                tunnel: w698 -> [w701 w710]
                                tunnel: [w704 w709] -> w697
                                tunnel: [w703 w708] -> w696
                                tunnel: "settling\ndelay [ms]" -> [w702 w706]
                                frame False {
                                n271 = call "Pinholes.vi"("Current Threshold [nA]"=w701, "settling\ndelay"=w702) -> ("excluded channels"=w703:i32[], "Current [nA]"=w705:dbl[], "Flag"=w704:i32[])  [unwired: 3 in]
                                }
                                frame True {
                                n272 = call "PinholesRolling.vi"("Current Threshold [nA]"=w710, "settling\ndelay"=w706) -> ("excluded channels"=w708:i32[], "Current [nA]"=w707:dbl[], "Flag"=w709:i32[])  [unwired: 3 in]
                                }
                                }
                                "disabled channels" <- w696
                                }
                                frame True {
                                n273 = local read "Probe Card Channels"() -> (w711:i32)
                                n274 = for {
                                N: w711 -> [_]
                                tunnel: [w715] -> w713 mode=indexing
                                tunnel: [w714] -> w712 mode=indexing
                                # "Simulate"
                                n275 = Random Number (0-1)() -> (number: 0 to 1=w718:dbl)
                                n276 = Greater?(x=w718, y=0.95) -> (0:w719:bool)
                                n277 = case shown="True" w719 {
                                tunnel: [w723 5000.0] -> w715
                                tunnel: w718 -> [w723 _]
                                frame False {
                                }
                                frame True {
                                }
                                }
                                n278 = Greater?(x=w715, y=50.0) -> (0:w716:bool)
                                n279 = case shown="True" w716 {
                                tunnel: [0 1] -> w714
                                frame False {
                                }
                                frame True {
                                }
                                }
                                }
                                }
                                }
                                n280 = Get Date/Time String(want seconds? (F)=TRUE) -> (time string=→"Last Probe at:":string)  [unwired: 2 in, 1 out]
                                n281 = local write "Status"("Measuring Ipinhole") -> ()
                                n282 = Index Array(array=w680, index=0) -> (element=→"Current [nA]:":dbl)
                                n283 = To Double Precision Float(number=w686) -> (double precision float=w683:dbl[])
                                n284 = call "MultiRegionData.vi"("Action"=w684, "Array No."=1, "Array Size / Index"=w687, "Array IN"=w680, "Region index"=w688) -> ()  [unwired: 1 in, 2 out]
                                n285 = call "MultiRegionData.vi"("Action"=w685, "Array No."=2, "Array Size / Index"=w687, "Array IN"=w683, "Region index"=w688) -> ()  [unwired: 1 in, 2 out]
                                }
                                frame True {
                                }
                                }
                                }
                                }
                                }
                              }
                              n286 = Get Date/Time In Seconds() -> (seconds since 1Jan1904=w656:timestamp)
                              n287 = To Double Precision Float(number=w656) -> (double precision float=w654:dbl)
                              n288 = To Double Precision Float(number=timestamp(2082841200 s since 1904-01-01) ("current time")) -> (double precision float=w653:dbl)
                              n289 = Subtract(x=w654, y=w653) -> (x-y=w652:dbl)
                              n290 = call "MultiRegionData.vi"("Action"=T7."Write Element", "Array No."=u32 9, "Array Size / Index"=w657, "Data IN"=w652, "Region index"=w659) -> ()  [unwired: 1 in, 2 out]
                            }
                            frame #2 {
                              # "Probestation temperature"
                              # "Capacitance and Resistance"
                              n291 = local read "Simulation?"() -> (w786:bool)
                              n292 = call <instrlib>:"GetHeaterTemp.vi"("Unit"=enum16{"Celcius", "Fahrenheit", "Kelvin"}."Celcius") -> ("Actual Temperature"=w778:dbl, "Error Out"=w779:errorcluster)  [unwired: 10 in, 3 out]
                              n293 = case shown="Error" w779 {
                                tunnel: w778 -> [w787 _]
                                tunnel: [w787 nan ("Actual Temperature")] -> w777
                                frame No Error {
                                }
                                frame Error {
                                }
                              }
                              n294 = stacked-sequence {
                                seq-local: [_ _ w818 _] -> [_ _ _ w879]
                                tunnel: w780 -> [_ _ w828 _]
                                tunnel: w781 -> [_ _ w827 _]
                                tunnel: w786 -> [w793 w812 w817 w878]
                                tunnel: w785 -> [w792 w811 w816 w877]
                                tunnel: w780 -> [w791 _ _ _]
                                tunnel: w781 -> [w790 _ _ _]
                                tunnel: w776 -> [w789 _ _ _]
                                frame #0 {
                                n295 = case shown="True" w789 {
                                tunnel: w793 -> [_ w795]
                                tunnel: w792 -> [_ w794]
                                frame False {
                                }
                                frame True {
                                n296 = case shown="False" w795 {
                                tunnel: w794 -> [w797 _]
                                frame False {
                                # "Grounding takes about 500 ms"
                                n297 = call-dynamic "MatrixSwitch.vi"("Action"=T5."Ground", "Switching in"=w797) -> ()  [unwired: 7 in, 3 out]
                                n298 = Wait (ms)(milliseconds to wait=u32 500) -> ()  [unwired: 1 out]
                                }
                                frame True {
                                }
                                }
                                }
                                }
                                n299 = disable-structure shown="Enabled" {
                                disable-tunnel: w791 -> [w801 _]
                                disable-tunnel: w790 -> [w800 _]
                                frame Enabled {
                                # "read the leakage current"
                                n300 = flat-sequence {
                                tunnel: w800 -> [w803]
                                tunnel: [w803] -> w799
                                tunnel: w801 -> [w808]
                                tunnel: w799 -> [w805]
                                frame #0 {
                                n301 = Wait (ms)(milliseconds to wait=u32 100) -> ()  [unwired: 1 out]
                                }
                                frame #1 {
                                n302 = global read "QC_MeasurementSetup.vi" "Striptest Measurement Parameters"() -> (w810:T9)
                                n303 = Unbundle By Name(w810) -> ("Bias Supply"=w809:refnum<class "SupplyControl.lvclass">)
                                n304 = call-dynamic "Supply_ReadCurrent.vi"("SupplyControl in"=w809) -> ("Current in nA"=w804:dbl)  [unwired: 8 in, 2 out]
                                n305 = call "MultiRegionData.vi"("Action"=T7."Write Element", "Array No."=u32 5, "Array Size / Index"=w805, "Data IN"=w804, "Region index"=w808) -> ()  [unwired: 1 in, 2 out]
                                }
                                }
                                }
                                frame Disabled {
                                }
                                }
                                }
                                frame #1 {
                                n306 = case shown="False" w812 {
                                tunnel: w811 -> [w814 _]
                                frame False {
                                n307 = call-dynamic "MatrixSwitch.vi"("Action"=T5."Striptest LCR", "Switching in"=w814) -> ()  [unwired: 7 in, 3 out]
                                }
                                frame True {
                                }
                                }
                                n308 = local write "Status"("Measuring capacitance..." ("STATUS 1")) -> ()
                                }
                                frame #2 {
                                w821 = 0
                                w825 = u32 4 items=["Reset", "Read Array", "Read Element", "Write Element", "Write Array"] ("Action")
                                w826 = u32 4 items=["Reset", "Read Array", "Read Element", "Write Element", "Write Array"] ("Action")
                                n309 = local read "Probe Card Channels"() -> (w818:i32)
                                n310 = local read "disabled channels"() -> (w820:i32[])
                                n311 = for {
                                N: w818 -> [_]
                                tunnel: [w837] -> w819 mode=indexing
                                tunnel: [w836] -> w822 mode=indexing
                                tunnel: w820 -> [w833]
                                tunnel: w818 -> [w835]
                                tunnel: w817 -> [w832]
                                tunnel: w816 -> [w831]
                                i -> [w834]
                                n312 = case shown="False" w832 {
                                tunnel: [w846 w868] -> w837
                                tunnel: [w845 w867] -> w836
                                tunnel: w835 -> [w842 _]
                                tunnel: w834 -> [w840 _]
                                tunnel: w833 -> [w841 _]
                                tunnel: w831 -> [w838 _]
                                frame False {
                                n313 = Increment(x=w840) -> (x+1=w839:i32)
                                n314 = Search 1D Array(1D array=w841, element=w839) -> (index of element=w844:i32)  [unwired: 1 in]
                                n315 = Less Than 0?(x=w844) -> (x < 0?=w843:bool)
                                n316 = case shown="True" w843 {
                                tunnel: [w849 w850] -> w846
                                tunnel: [w847 w855] -> w845
                                tunnel: w842 -> [_ w854]
                                tunnel: w839 -> [_ w853]
                                tunnel: w841 -> [_ w852]
                                tunnel: w838 -> [_ w851]
                                frame False {
                                w849 = -1.0
                                n317 = Divide(x=w849, y=1000000.0) -> (x/y=w847:dbl)
                                }
                                frame True {
                                n318 = stacked-sequence {
                                tunnel: w854 -> [w858 _ _]
                                tunnel: w853 -> [w860 _ _]
                                tunnel: w852 -> [w859 _ _]
                                tunnel: [_ _ w862] -> w850
                                tunnel: [_ _ w866] -> w855
                                tunnel: w851 -> [w857 _ _]
                                frame #0 {
                                n319 = local read "Single Needle"() -> (w856:bool)
                                n320 = call-dynamic "MuxCardSwitch.vi"("Single Needle"=w856, "Probe Card Channels"=w858, "disabled channels"=w859, "Switch to channel"=w860, "Switching in"=w857) -> ()  [unwired: 4 in, 3 out]
                                }
                                frame #1 {
                                n321 = local read "settling\ndelay [ms]"() -> (w861:i32)
                                n322 = Wait (ms)(milliseconds to wait=w861) -> ()  [unwired: 1 out]
                                }
                                frame #2 {
                                n323 = global read "QC_MeasurementSetup.vi" "Striptest Measurement Parameters"() -> (w865:T9)
                                n324 = Unbundle By Name(w865) -> ("LCR"=w864:refnum<class "LCRControl.lvclass">, "AC frequency [Hz]"=w863:i32)
                                n325 = call-dynamic "LCR_Readout.vi"("Frequency in Hz"=w863, "LCRControl in"=w864) -> ("Resistance in MOhm"=w866:dbl, "Capacitance in pF"=w862:dbl)  [unwired: 6 in, 2 out]
                                }
                                }
                                }
                                }
                                }
                                frame True {
                                n326 = Random Number (0-1)() -> (number: 0 to 1=w872:dbl)
                                n327 = Random Number (0-1)() -> (number: 0 to 1=w876:dbl)
                                n328 = Multiply(x=w876, y=18.0) -> (x*y=w874:dbl)
                                n329 = Multiply(x=w872, y=0.6) -> (x*y=w869:dbl)
                                n330 = Add(x=w874, y=64.0) -> (x+y=w868:dbl)
                                n331 = Add(x=1.5 ("Resistance"), y=w869) -> (x+y=w867:dbl)
                                }
                                }
                                }
                                n332 = Index Array(array=w819, index=w821) -> (element=→"Capacitance [pF]:":dbl)
                                n333 = Index Array(array=w822, index=w821) -> (element=→"Reistance [MW]:":dbl)
                                n334 = call "MultiRegionData.vi"("Action"=w826, "Array No."=3, "Array Size / Index"=w827, "Array IN"=w819, "Region index"=w828) -> ()  [unwired: 1 in, 2 out]
                                n335 = call "MultiRegionData.vi"("Action"=w825, "Array No."=4, "Array Size / Index"=w827, "Array IN"=w822, "Region index"=w828) -> ()  [unwired: 1 in, 2 out]
                                }
                                frame #3 {
                                n336 = case shown="False" w878 {
                                tunnel: w879 -> [w882 _]
                                tunnel: w877 -> [w880 _]
                                frame False {
                                n337 = local read "Single Needle"() -> (w881:bool)
                                n338 = call-dynamic "MuxCardSwitch.vi"("Single Needle"=w881, "Probe Card Channels"=w882, "Switch to channel"=-1, "Switching in"=w880) -> ()  [unwired: 5 in, 3 out]
                                }
                                frame True {
                                }
                                }
                                }
                              }
                              n339 = call "MultiRegionData.vi"("Action"=T7."Write Element", "Array No."=u32 8, "Array Size / Index"=w781, "Data IN"=w777, "Region index"=w780) -> ()  [unwired: 1 in, 2 out]
                            }
                            frame #3 {
                              # "display partial results"
                              # "If selected region is CURRENT region being probed,\nuse number probed so far\notherwise total number of probepoints in this region"
                              n340 = local read "Region Indices"() -> (w898:i32[])
                              n341 = property on="Set display for:" class="Ring (strict)"() -> ("RingText.Text"=→"Stats:":string)  [unwired: 2 in, 2 out]
                              n342 = Index Array(array=w898, index="Set display for:") -> (element=w894:i32)
                              n343 = Equal?(x=w894, y=w896) -> (x = y?=w897:bool)
                              n344 = case shown="True" w897 {
                                tunnel: w895 -> [_ w911]
                                tunnel: [w907 w910] -> w893
                                tunnel: w894 -> [w906 _]
                                frame False {
                                n345 = local read "probe points per region"() -> (w908:i32[])
                                n346 = Index Array(array=w908, index=w906) -> (element=w907:i32)
                                }
                                frame True {
                                n347 = local read "Probe Card Channels"() -> (w909:i32)
                                n348 = Add(x=w909, y=w911) -> (x+y=w910:i32)
                                }
                              }
                              n349 = local read "max scale array"() -> (w890:i32[])
                              n350 = local read "min scale array"() -> (w892:i32[])
                              n351 = local read "Thresholds"() -> (w905:T1)
                              n352 = Index Array(array=w890, index="Set display for:") -> (element=w886:i32)
                              n353 = Index Array(array=w892, index="Set display for:") -> (element=w888:i32)
                              n354 = call "DisplayStriptestData.vi"("min scale array"=w892, "max scale array"=w890, "# probed"=w893, "Display Stats?"="Display Stats", "Thresholds"=w905, "Region"=w894) -> ("Defects"=w900:i32[][], "Resistance [MW]"=→"Resistance [MW]":cluster{u32, i32, "Array OUT":dbl[]}, "Capacitance [pF]"=→"Capacitance [pF]":cluster{u32, i32, "Array OUT":dbl[]}, "Current [nA]"=→"Current [nA]":cluster{u32, i32, "Array OUT":dbl[]}, "Strip Quality Data"=w901:T16)
                              n355 = case shown="True" "Display Stats" {
                                tunnel: w901 -> [_ w917]
                                tunnel: w900 -> [_ w916]
                                frame False {
                                }
                                frame True {
                                n356 = Unbundle By Name(w917) -> ("pass Rate in %"=→"% OK:":dbl, "Bad channel list"=→"Bad Strip List":i32[], "No of bad strips"=w915:i32, "Number of defects per category"=→"defect type array":i32[])
                                n357 = local write "# total defects:"(w915) -> ()
                                "Defects" <- w916
                                }
                              }
                              n358 = Increment(x=w886) -> (x+1=w885:i32)
                              n359 = Increment(x=w888) -> (x+1=w887:i32)
                              n360 = Increment(x=w885) -> (x+1=w884:i32)
                              n361 = property on="Capacitance [pF]" class="WFGraph (strict)"("XScale.Minimum"=w887) -> ()  [unwired: 2 in, 2 out]
                              n362 = property on="Resistance [MW]" class="WFGraph (strict)"("XScale.Minimum"=w887) -> ()  [unwired: 2 in, 2 out]
                              n363 = property on="Current [nA]" class="WFGraph (strict)"("XScale.Minimum"=w887) -> ()  [unwired: 2 in, 2 out]
                              n364 = property on="Defects" class="IntGraph (strict)"("XScale.Minimum"=w887) -> ()  [unwired: 2 in, 2 out]
                              n365 = property on="Capacitance [pF]" class="WFGraph (strict)"("XScale.Maximum"=w885) -> ()  [unwired: 2 in, 2 out]
                              n366 = property on="Resistance [MW]" class="WFGraph (strict)"("XScale.Maximum"=w885) -> ()  [unwired: 2 in, 2 out]
                              n367 = property on="Current [nA]" class="WFGraph (strict)"("XScale.Maximum"=w885) -> ()  [unwired: 2 in, 2 out]
                              n368 = property on="Defects" class="IntGraph (strict)"("XScale.Maximum"=w884) -> ()  [unwired: 2 in, 2 out]
                            }
                            frame #4 {
                              # "display stats"
                              # "save image if required"
                              n369 = call "RunTime.vi"("Probing done - new estimation"=TRUE, "Flag"=0) -> ("Estimated Completion Time"=w930:string, "Time so far"=→"Run Duration:":string)  [unwired: 2 in, 2 out]
                              n370 = Greater Or Equal?(x=w921, y=20) -> (x >= y?=w927:bool)
                              n371 = case shown="True" w927 {
                                selector: w927 -> [_ w935]
                                frame False {
                                }
                                frame True {
                                # "Start calculating stats after 20 strips"
                                n372 = local write "Display Stats"(w935) -> ()
                                }
                              }
                              n373 = Scan From String(format string="%s %s", input string=w930) -> (output 2=→"Estimated Completion Time":string)  [unwired: 5 in, 3 out]
                              n374 = local read "Probe Card Channels"() -> (w922:i32)
                              n375 = Quotient & Remainder(x=w921, y=w922) -> (floor(x/y)=w920:i32)  [unwired: 1 out]
                              n376 = Add(x=w922, y=w934) -> (x+y=w924:i32)
                              n377 = local write "# probed"(w924) -> ()
                              n378 = Increment(x=w920) -> (x+1=w919:i32)
                              n379 = call "SaveJPEG.vi"("Picture No."=w919, "Test"="Striptest") -> ()  [unwired: 1 in, 2 out]
                              n380 = Increment(x=w923) -> (x+1=w933:i32)
                            }
                          }
                        }
                      }
                      n381 = Build Array(w324, "Abort", w308) -> (w325:bool[])
                      n382 = Or Array Elements(Boolean array=w325) -> (logical OR=w326:bool)
                    }
                    n383 = Increment(x=w306) -> (x+1=w299:i32)
                  }
                }
              }
              n384 = local write "Temperature Progression"(w266) -> ()
            }
            frame True {
            }
          }
        }
        frame #5 {
          # "5"
          # "Ramp down volts now"
          n385 = case shown="True" w942 {
            tunnel: w941 -> [w963 _]
            frame False {
              w968 = "0"
              n386 = property on="Abort" class="Bool (strict)"("DisabledEnum"=2) -> ()  [unwired: 2 in, 2 out]
              n387 = local read "# probed"() -> (w961:i32)
              n388 = call-dynamic "Prober_ChuckUpDown.vi"("Direction"=enum16{"up", "down"}."down", "ProbeStationControl in"=w963) -> ("error out"=w965:errorcluster, "ProbeStationControl out"=w964:refnum<class "ProbeStationControl.lvclass">)  [unwired: 7 in, 1 out]
              n389 = call "SaveJPEG.vi"("Picture No."=w961, "Test"="Striptest") -> ()  [unwired: 1 in, 2 out]
              n390 = call-dynamic "Prober_MoveToXYZTheta.vi"("Theta location [mdeg]"="none", "ProbeStationControl in"=w964, "error in (no error)"=w965, "Z location [µm]"="down", "Y location [µm]"=w968, "X location [µm]"=w968) -> ()  [unwired: 3 in, 3 out]
            }
            frame True {
            }
          }
          n391 = local read "Abort"() -> (w954:bool)
          n392 = property on="Bias On/Off:" class="Bool (strict)"() -> ("Blinking"=w953:bool)  [unwired: 2 in, 2 out]
          n393 = Not Or(1:w954, 2:w953) -> (0:w952:bool)
          n394 = Build Array(w952, w953, w954) -> (w955:bool[])
          n395 = Search 1D Array(1D array=w955, element=TRUE) -> (index of element=w957:i32)  [unwired: 1 in]
          n396 = Increment(x=w957) -> (x+1=w943:i32)
          n397 = Pick Line(multi-line string=" null\n Run ended normally.\n Compliance exceeded. \n Run aborted early.", line index=w943) -> (output string=w944:string)  [unwired: 1 in]
          n398 = global read "QC_RunInformation.vi" "Run info"() -> (w946:T12)
          n399 = Bundle By Name(cluster=w946, "End of Run comment:"=w944) -> (w945:T12)
          n400 = Concatenate Strings(" End of Run.", "\r\n", w944) -> (w947:string)
          n401 = Concatenate Strings(w944, "\r\n", "RAMPING DOWN VOLTS") -> (w950:string)
          n402 = global write "QC_RunInformation.vi" "Run info"(w945) -> ()
          n403 = stacked-sequence {
            tunnel: w950 -> [w970 _ _ _]
            tunnel: w947 -> [_ _ w974 _]
            frame #0 {
              n404 = local write "Status"(w970) -> ()
            }
            frame #1 {
              n405 = local read "Simulation?"() -> (w971:bool)
              n406 = case shown="False" w971 {
                frame False {
                  n407 = global read "QC_MeasurementSetup.vi" "Striptest Measurement Parameters"() -> (w973:T9)
                  n408 = Unbundle By Name(w973) -> ("SMU"=w972:refnum<class "SupplyControl.lvclass">)
                  n409 = call-dynamic "Supply_Stby.vi"("SupplyControl in"=w972) -> ()  [unwired: 9 in, 2 out]
                }
                frame True {
                }
              }
            }
            frame #2 {
              n410 = local write "Status"(w974) -> ()
            }
            frame #3 {
              w976 = 0
              n411 = disable-structure shown="Disabled" {
                frame Disabled {
                  n412 = property on="Auto ReCheck" class="Bool (strict)"("DisabledEnum"=1) -> ()  [unwired: 2 in, 2 out]
                }
                frame Enabled {
                }
              }
              n413 = property on="Save Data" class="Bool (strict)"("DisabledEnum"=w976) -> ()  [unwired: 2 in, 2 out]
              n414 = property on="Quit w/o saving" class="Bool (strict)"("DisabledEnum"=w976) -> ()  [unwired: 2 in, 2 out]
              n415 = property on="ReCheck" class="Bool"("DisabledEnum"=w976) -> ()  [unwired: 2 in, 2 out]
              n416 = local write "Status"("Run finished. \nSave data?" ("STATUS 1")) -> ()
            }
          }
        }
        frame #6 {
          w991 = ""
          # "6"
          n417 = stacked-sequence {
            tunnel: [w1057 _ _ _] -> w1007
            tunnel: [w1056 _ _ _] -> w1006
            tunnel: w1000 -> [_ w1202 w1217 _]
            tunnel: w999 -> [w1055 _ _ _]
            frame #0 {
              # "saving data"
              # "Loop and await decision on whether to save or junk data"
              n418 = local read "Set display for:"() -> (w1058:u16)
              n419 = while {
                shift-right: [w1067] -> _
                shift-left: w1058 -> [w1068]
                tunnel: ["Save Data"] -> w1056
                tunnel: ["Quit w/o saving"] -> w1057
                tunnel: w1055 -> [w1060]
                stop <- w1071 stop-if-true
                n420 = local read "Set display for:"() -> (w1069:u16)
                n421 = Or(x="Auto ReCheck", y="ReCheck") -> (x .or. y?=w1062:bool)
                n422 = Not Equal?(x=w1069, y=w1068) -> (x != y?=w1070:bool)
                n423 = Wait (ms)(milliseconds to wait=u32 200) -> ()  [unwired: 1 out]
                n424 = case shown="True" w1070 {
                  tunnel: w1069 -> [w1177 w1185]
                  tunnel: [w1177 w1185] -> w1067
                  frame False {
                  }
                  frame True {
                    # "display data if selected region changes"
                    n425 = local read "Thresholds"() -> (w1200:T1)
                    n426 = local read "Region Indices"() -> (w1186:i32[])
                    n427 = local read "probe points per region"() -> (w1195:i32[])
                    n428 = local read "min scale array"() -> (w1197:i32[])
                    n429 = property on="Set display for:" class="Ring (strict)"() -> ("RingText.Text"=w1183:string)  [unwired: 2 in, 2 out]
                    n430 = Index Array(array=w1186, index=w1185) -> (element=w1184:i32)
                    n431 = Index Array(array=w1195, index=w1185) -> (element=w1201:i32)
                    n432 = local read "max scale array"() -> (w1196:i32[])
                    n433 = call "DisplayStriptestData.vi"("min scale array"=w1197, "max scale array"=w1196, "# probed"=w1201, "Display Stats?"=TRUE, "Thresholds"=w1200, "Region"=w1184) -> ("Defects"=w1198:i32[][], "Resistance [MW]"=w1192:cluster{u32, i32, "Array OUT":dbl[]}, "Capacitance [pF]"=w1193:cluster{u32, i32, "Array OUT":dbl[]}, "Current [nA]"=w1194:cluster{u32, i32, "Array OUT":dbl[]}, "Strip Quality Data"=w1199:T16)
                    n434 = Unbundle By Name(w1199) -> ("pass Rate in %"=w1189:dbl, "Bad channel list"=w1187:i32[], "No of bad strips"=w1190:i32, "Number of defects per category"=w1188:i32[])
                    n435 = local write "Capacitance [pF]"(w1193) -> ()
                    n436 = local write "Resistance [MW]"(w1192) -> ()
                    n437 = local write "Stats:"(w1183) -> ()
                    n438 = local write "Current [nA]"(w1194) -> ()
                    n439 = local write "% OK:"(w1189) -> ()
                    n440 = local write "Bad Strip List"(w1187) -> ()
                    n441 = local write "# total defects:"(w1190) -> ()
                    n442 = local write "defect type array"(w1188) -> ()
                    n443 = Index Array(array=w1196, index=w1185) -> (element=w1182:i32)
                    n444 = Index Array(array=w1197, index=w1185) -> (element=w1181:i32)
                    n445 = local write "Defects"(w1198) -> ()
                    n446 = Increment(x=w1182) -> (x+1=w1179:i32)
                    n447 = Increment(x=w1179) -> (x+1=w1178:i32)
                    n448 = property on="Defects" class="IntGraph (strict)"("XScale.Maximum"=w1178) -> ()  [unwired: 2 in, 2 out]
                    n449 = Increment(x=w1181) -> (x+1=w1180:i32)
                    n450 = property on="Current [nA]" class="WFGraph (strict)"("XScale.Maximum"=w1179) -> ()  [unwired: 2 in, 2 out]
                    n451 = property on="Capacitance [pF]" class="WFGraph (strict)"("XScale.Maximum"=w1179) -> ()  [unwired: 2 in, 2 out]
                    n452 = property on="Current [nA]" class="WFGraph (strict)"("XScale.Minimum"=w1180) -> ()  [unwired: 2 in, 2 out]
                    n453 = property on="Capacitance [pF]" class="WFGraph (strict)"("XScale.Minimum"=w1180) -> ()  [unwired: 2 in, 2 out]
                    n454 = property on="Defects" class="IntGraph (strict)"("XScale.Minimum"=w1180) -> ()  [unwired: 2 in, 2 out]
                    n455 = property on="Resistance [MW]" class="WFGraph (strict)"("XScale.Minimum"=w1180) -> ()  [unwired: 2 in, 2 out]
                    n456 = property on="Resistance [MW]" class="WFGraph (strict)"("XScale.Maximum"=w1179) -> ()  [unwired: 2 in, 2 out]
                  }
                }
                n457 = case shown="True" w1062 {
                  tunnel: "Auto ReCheck" -> [_ w1111]
                  tunnel: w1060 -> [_ w1110]
                  frame False {
                  }
                  frame True {
                    n458 = case shown="True" w1111 {
                      tunnel: w1110 -> [_ w1142]
                      frame False {
                        n459 = local read "probe points per region"() -> (w1118:i32[])
                        n460 = local read "Region Indices"() -> (w1119:i32[])
                        n461 = local read "Set display for:"() -> (w1117:u16)
                        n462 = Index Array(array=w1119, index=w1117) -> (element=w1116:i32)
                        n463 = Index Array(array=w1118, index=w1117) -> (element=w1115:i32)
                        n464 = flat-sequence {
                          tunnel: w1116 -> [w1121]
                          tunnel: w1115 -> [w1125]
                          tunnel: [w1121] -> w1114
                          tunnel: [w1125] -> w1113
                          tunnel: [w1124] -> w1112
                          tunnel: w1114 -> [w1141]
                          tunnel: w1113 -> [w1138]
                          tunnel: w1112 -> [w1127]
                          frame #0 {
                            n465 = local read "Probe Card Channels"() -> (w1122:i32)
                            n466 = local read "Auto ReCheck"() -> (w1123:bool)
                            n467 = local read "Thresholds"() -> (w1126:T1)
                            n468 = call "ReCheckStrips.vi"("Probe Card Channels"=w1122, "Auto Re-Check"=w1123, "Thresholds"=w1126, "Bias ramp up&down"=FALSE, "region in"=w1121, "Number of strips probed"=w1125) -> ("Thresholds copy"=w1124:T17)  [unwired: 5 in]
                            n469 = local write "Thresholds"(w1124) -> ()
                          }
                          frame #1 {
                            n470 = local read "max scale array"() -> (w1140:i32[])
                            n471 = local read "min scale array"() -> (w1139:i32[])
                            n472 = call "DisplayStriptestData.vi"("min scale array"=w1139, "max scale array"=w1140, "# probed"=w1138, "Display Stats?"=TRUE, "Thresholds"=w1127, "Region"=w1141) -> ("Defects"=w1133:i32[][], "Resistance [MW]"=w1134:cluster{u32, i32, "Array OUT":dbl[]}, "Capacitance [pF]"=w1136:cluster{u32, i32, "Array OUT":dbl[]}, "Current [nA]"=w1135:cluster{u32, i32, "Array OUT":dbl[]}, "Strip Quality Data"=w1132:T16)
                            n473 = local write "Defects"(w1133) -> ()
                            n474 = local write "Current [nA]"(w1135) -> ()
                            n475 = local write "Capacitance [pF]"(w1136) -> ()
                            n476 = local write "Resistance [MW]"(w1134) -> ()
                            n477 = Unbundle By Name(w1132) -> ("pass Rate in %"=w1131:dbl, "Bad channel list"=w1130:i32[], "No of bad strips"=w1129:i32, "Defect description list"=w1128:i32[])
                            n478 = local write "% OK:"(w1131) -> ()
                            n479 = local write "Bad Strip List"(w1130) -> ()
                            n480 = local write "# total defects:"(w1129) -> ()
                            n481 = local write "defect type array"(w1128) -> ()
                          }
                        }
                      }
                      frame True {
                        n482 = flat-sequence {
                          tunnel: w1142 -> [w1143]
                          frame #0 {
                            n483 = local read "Region Indices"() -> (w1144:i32[])
                            n484 = Array Size(array=w1144) -> (size(s)=w1145:i32)
                            n485 = for {
                              N: w1145 -> [_]
                              tunnel: w1144 -> [w1147] mode=indexing
                              tunnel: w1143 -> [w1146] mode=indexing
                              n486 = case shown="True" w1146 {
                                tunnel: w1147 -> [_ w1151]
                                frame False {
                                }
                                frame True {
                                n487 = local read "probe points per region"() -> (w1153:i32[])
                                n488 = Index Array(array=w1153, index=w1151) -> (element=w1152:i32)
                                n489 = flat-sequence {
                                tunnel: w1151 -> [w1159]
                                tunnel: w1152 -> [w1158]
                                tunnel: [w1159] -> w1150
                                tunnel: [w1158] -> w1149
                                tunnel: [w1157] -> w1148
                                tunnel: w1150 -> [w1175]
                                tunnel: w1149 -> [w1172]
                                tunnel: w1148 -> [w1161]
                                frame #0 {
                                n490 = local read "Probe Card Channels"() -> (w1155:i32)
                                n491 = local read "Auto ReCheck"() -> (w1156:bool)
                                n492 = local read "Thresholds"() -> (w1160:T1)
                                n493 = call "ReCheckStrips.vi"("Probe Card Channels"=w1155, "Auto Re-Check"=w1156, "Thresholds"=w1160, "Bias ramp up&down"=FALSE, "region in"=w1159, "Number of strips probed"=w1158) -> ("Thresholds copy"=w1157:T17)  [unwired: 5 in]
                                n494 = local write "Thresholds"(w1157) -> ()
                                }
                                frame #1 {
                                n495 = local read "max scale array"() -> (w1174:i32[])
                                n496 = local read "min scale array"() -> (w1173:i32[])
                                n497 = call "DisplayStriptestData.vi"("min scale array"=w1173, "max scale array"=w1174, "# probed"=w1172, "Display Stats?"=TRUE, "Thresholds"=w1161, "Region"=w1175) -> ("Defects"=w1167:i32[][], "Resistance [MW]"=w1168:cluster{u32, i32, "Array OUT":dbl[]}, "Capacitance [pF]"=w1170:cluster{u32, i32, "Array OUT":dbl[]}, "Current [nA]"=w1169:cluster{u32, i32, "Array OUT":dbl[]}, "Strip Quality Data"=w1166:T16)
                                n498 = local write "Defects"(w1167) -> ()
                                n499 = local write "Current [nA]"(w1169) -> ()
                                n500 = local write "Capacitance [pF]"(w1170) -> ()
                                n501 = local write "Resistance [MW]"(w1168) -> ()
                                n502 = Unbundle By Name(w1166) -> ("pass Rate in %"=w1165:dbl, "Bad channel list"=w1164:i32[], "No of bad strips"=w1163:i32, "Number of defects per category"=w1162:i32[])
                                n503 = local write "% OK:"(w1165) -> ()
                                n504 = local write "Bad Strip List"(w1164) -> ()
                                n505 = local write "# total defects:"(w1163) -> ()
                                n506 = local write "defect type array"(w1162) -> ()
                                }
                                }
                                }
                              }
                            }
                          }
                          frame #1 {
                            n507 = local write "Auto ReCheck"(FALSE) -> ()
                          }
                        }
                      }
                    }
                  }
                }
                n508 = Or(x="Save Data", y="Quit w/o saving") -> (x .or. y?=w1071:bool)
                n509 = case shown="True" "PreSave Data" {
                  frame False {
                  }
                  frame True {
                    n510 = local write "PreSave Data"(FALSE ("PresaSave Data")) -> ()
                    n511 = global read "ProbePlanParams.vi" "ProbePlan Parameters IN"() -> (w1074:T10)
                    n512 = Unbundle By Name(w1074) -> ("Test ProbePoints.Regions Enabled"=w1076:bool[], "ProbePlan array"=w1077:T11)
                    n513 = Array Size(array=w1076) -> (size(s)=w1075:i32)
                    n514 = case shown="True" FALSE {
                      tunnel: w1075 -> [_ w1080]
                      tunnel: w1076 -> [_ w1079]
                      tunnel: w1077 -> [_ w1078]
                      frame False {
                      }
                      frame True {
                        n515 = for {
                          N: w1080 -> [_]
                          tunnel: w1079 -> [w1083] mode=indexing
                          tunnel: w1078 -> [w1082] mode=indexing
                          i -> [w1081]
                          n516 = case shown="True" w1083 {
                            tunnel: w1081 -> [_ w1085]
                            tunnel: w1082 -> [_ w1084]
                            frame False {
                            }
                            frame True {
                              n517 = flat-sequence {
                                tunnel: w1085 -> [w1092]
                                tunnel: w1084 -> [w1087]
                                frame #0 {
                                w1088 = 10  # No. of columns
                                (unwired) "%016.6f" ("Arrays format")
                                n518 = local read "Temperature Progression"() -> (w1096:T3)
                                n519 = local read "probe points per region"() -> (w1104:i32[])
                                n520 = Initialize Array(1.0 ("element"), w1088) -> (w1089:dbl[])
                                n521 = Unbundle By Name(w1087) -> ("Region"=w1086:string)
                                n522 = for {
                                N: w1088 -> [_]
                                tunnel: w1092 -> [w1107]
                                tunnel: [w1106] -> w1091 mode=indexing
                                tunnel: w1089 -> [w1105] mode=indexing
                                i -> [w1109]
                                n523 = call "MultiRegionData.vi"("Action"=T7."Read Array", "Array No."=w1109, "Region index"=w1107) -> ("Array OUT"=w1106:dbl[])  [unwired: 3 in, 1 out]
                                n524 = Multiply(x=w1106, y=w1105) -> ()  [unwired: 1 out]
                                }
                                n525 = Concatenate Strings("Saving data for " ("string"), w1086) -> (w1103:string)
                                n526 = local write "Status"(w1103) -> ()
                                n527 = Unbundle By Name(w1096) -> ("Temperature Array [°C]"=w1095:dbl[], "Humidity Array [RH %]"=w1094:dbl[])
                                n528 = Index Array(array=w1104, index=w1092) -> (element=w1100:i32)
                                n529 = Transpose 2D Array(2D array=w1091) -> (transposed array=w1093:dbl[][])
                                n530 = call <vilib>:"Std Deviation and Variance.vi"("X"=w1095) -> ("mean"=w1098:dbl)  [unwired: 1 in, 2 out]
                                n531 = call <vilib>:"Std Deviation and Variance.vi"("X"=w1094) -> ("mean"=w1097:dbl)  [unwired: 1 in, 2 out]
                                n532 = call "SaveDataFile.vi"("Data Array"=w1093, "Temperature"=w1098, "Humidity"=w1097, "no. of arrays"=w1088, "Actual array lengths"=w1100, "Array Titles"="ProbeplanIndex\tCurrent[nA] PinholeFlag\tCapacitance[pF]\tResistance[MOhm]\tLeakage[nA]\tTemperature[DegC]\tHumidity[%]\tChutckTemp[DegC]\tTimestamp[Unix]", "Strip Segment"=w1086, "Arrays format"="%^g") -> ()  [unwired: 4 in, 4 out]
                                }
                              }
                            }
                          }
                        }
                      }
                    }
                  }
                }
              }
              n533 = local write "Save Data"("Auto quit &\nswitch off bias") -> ()
            }
            frame #1 {
              n534 = case shown="False" w1202 {
                frame False {
                  # "supply to standby"
                  n535 = global read "QC_MeasurementSetup.vi" "Striptest Measurement Parameters"() -> (w1214:T9)
                  n536 = Unbundle By Name(w1214) -> ("Bias Supply"=w1203:refnum<class "SupplyControl.lvclass">, "Switching"=w1213:refnum<class "Switching.lvclass">)
                  n537 = local read "Current Bias Voltage [V]"() -> (w1207:dbl)
                  n538 = call-dynamic "MatrixSwitch.vi"("Action"=T5."Reset", "Switching in"=w1213) -> ("error out"=w1212:errorcluster)  [unwired: 7 in, 2 out]
                  n539 = call "SupplyRamp.vi"("error in"=w1212, "Requested Voltage"=0.0, "Step Size"=10.0, "Step Delay"=1000, "Supply IN"=w1203, "Starting Voltage"=w1207) -> ("error out"=w1210:errorcluster, "Supply OUT"=w1209:refnum<class "SupplyControl.lvclass">, "Current Voltage"=w1208:dbl)  [unwired: 2 in, 1 out]
                  n540 = call-dynamic "Supply_Stby.vi"("error in (no error)"=w1210, "SupplyControl in"=w1209) -> ()  [unwired: 8 in, 2 out]
                  n541 = local write "Current Bias Voltage [V]"(w1208) -> ()
                }
                frame True {
                }
              }
            }
            frame #2 {
              n542 = case shown="False" w1217 {
                frame False {
                  n543 = global read "QC_MeasurementSetup.vi" "Striptest Measurement Parameters"() -> (w1223:T9)
                  n544 = Unbundle By Name(w1223) -> ("Arduino"=w1227:refnum<class "ArduinoControl.lvclass">)
                  n545 = local read "Temperature Progression"() -> (w1232:T3)
                  n546 = local read "Run Duration:"() -> (w1229:string)
                  n547 = call "ArduinoRead.vi"("Arduino function"=enum16{"T/RH", "Interlock", "Edgesense"}."T/RH", "ArduinoControl in"=w1227) -> ("error out"=w1233:errorcluster, "rel. Humidity [%]"=w1220:dbl, "Temperature [°C]"=w1224:dbl, "ArduinoControl out"=w1234:refnum<class "ArduinoControl.lvclass">)  [unwired: 4 in, 2 out]
                  "Last Temperature [°C]" <- w1224
                  n548 = call "ArduinoClose.vi"("error in (no error)"=w1233, "ArduinoControl in"=w1234) -> ()  [unwired: 8 in, 2 out]
                  n549 = Unbundle(w1232) -> ("Time Array"=w1230:string[], "Temperature Array [°C]"=w1225:dbl[], "Humidity Array [RH %]"=w1221:dbl[])
                  n550 = Build Array (concatenate)(w1230, w1229) -> (w1228:string[])
                  n551 = Build Array (concatenate)(w1225, w1224) -> (w1222:dbl[])
                  n552 = Build Array (concatenate)(w1221, w1220) -> (w1219:dbl[])
                  n553 = Bundle(cluster=w1232, "Time Array"=w1228, "Temperature Array [°C]"=w1222, "Humidity Array [RH %]"=w1219) -> (w1231:T3)
                  n554 = local write "Temperature Progression"(w1231) -> ()
                }
                frame True {
                }
              }
              n555 = local read "# probed"() -> (w1216:i32)
              n556 = call "SaveJPEG.vi"("Picture No."=w1216, "Test"="Striptest") -> ()  [unwired: 1 in, 2 out]
              n557 = One Button Dialog(message="Please switch bias off NOW and then open\nprobestation enclosure and raise needle.") -> ()  [unwired: 1 in, 1 out]
            }
            frame #3 {
              n558 = One Button Dialog(message="Please ensure detector bias is OFF!") -> ()  [unwired: 1 in, 1 out]
            }
          }
          n559 = global read "ProbePlanParams.vi" "ProbePlan Parameters IN"() -> (w1004:T10)
          n560 = case shown="True" w1007 {
            tunnel: [FALSE w1336] -> w1005
            frame False {
            }
            frame True {
              n561 = Two Button Dialog(message="Are you sure you don't want to save the data?", 1:"Quit" ("F button name (\"Cancel\")"), 2:"Save data" ("T button name (\"OK\")")) -> (T button?=w1336:bool)
            }
          }
          n562 = Unbundle By Name(w1004) -> ("Test ProbePoints.Regions Enabled"=w1002:bool[], "ProbePlan array"=w1001:T11)
          n563 = Or(x=w1006, y=w1005) -> (x .or. y?=w978:bool)
          n564 = Array Size(array=w1002) -> (size(s)=w1003:i32)
          n565 = case shown="False" w978 {
            tunnel: w1003 -> [w1242 w1270]
            tunnel: w1002 -> [w1241 w1269]
            tunnel: w1001 -> [_ w1268]
            tunnel: [w1237 w1266] -> w980
            tunnel: [w1239 w1264] -> w998
            tunnel: ["" w1261] -> w997
            frame False {
              n566 = for {
                N: w1242 -> [_]
                tunnel: w1241 -> [w1246] mode=indexing
                tunnel: [w1245] -> w1240 mode=indexing
                tunnel: [w1244] -> w1238 mode=indexing
                i -> [w1243]
                n567 = case shown="True" w1246 {
                  tunnel: [100.0 w1251] -> w1245
                  tunnel: [TRUE w1250] -> w1244
                  tunnel: w1243 -> [_ w1249]
                  frame False {
                  }
                  frame True {
                    n568 = local read "probe points per region"() -> (w1257:i32[])
                    n569 = local read "max scale array"() -> (w1256:i32[])
                    n570 = local read "min scale array"() -> (w1255:i32[])
                    n571 = local read "Thresholds"() -> (w1259:T1)
                    n572 = Index Array(array=w1257) -> (element=w1253:i32)  [unwired: 1 in]
                    n573 = call "DisplayStriptestData.vi"("min scale array"=w1255, "max scale array"=w1256, "# probed"=w1253, "Display Stats?"=TRUE, "Thresholds"=w1259, "Region"=w1249) -> ("Strip Quality Data"=w1254:T16)  [unwired: 4 out]
                    n574 = Unbundle By Name(w1254) -> ("pass Rate in %"=w1251:dbl)
                    n575 = Greater?(x=w1251, y=98.0) -> (0:w1250:bool)
                  }
                }
              }
              n576 = And Array Elements(Boolean array=w1238) -> (logical AND=w1237:bool)
              n577 = Array Max & Min(array=w1240) -> (min value=w1239:dbl)  [unwired: 3 out]
            }
            frame True {
              n578 = for {
                N: w1270 -> [_]
                tunnel: w1269 -> [w1280] mode=indexing
                tunnel: w1268 -> [w1279] mode=indexing
                tunnel: [w1277] -> w1267 mode=indexing
                tunnel: [w1276] -> w1265 mode=indexing
                tunnel: [w1275] -> w1263
                shift-right: [w1274] -> w1260
                shift-left: _ -> [w1271]
                i -> [w1278]
                n579 = case shown="True" w1280 {
                  tunnel: w1278 -> [_ w1293]
                  tunnel: w1279 -> [_ w1292]
                  tunnel: [TRUE w1289] -> w1277
                  tunnel: [100.0 w1287] -> w1276
                  tunnel: [w1281 w1286] -> w1275
                  tunnel: [w1281 w1285] -> w1272
                  frame False {
                    w1281 = ""
                  }
                  frame True {
                    n580 = Unbundle By Name(w1292) -> ("Region"=w1291:string)
                    n581 = flat-sequence {
                      tunnel: w1293 -> [w1298]
                      tunnel: w1291 -> [w1300]
                      tunnel: [w1298] -> w1290
                      tunnel: [w1308] -> w1288
                      tunnel: [w1302] -> w1286
                      tunnel: [w1301] -> w1285
                      tunnel: [w1300] -> w1284
                      tunnel: w1290 -> [w1323]
                      tunnel: [w1325] -> w1289
                      tunnel: w1288 -> [w1321]
                      tunnel: [w1322] -> w1287
                      tunnel: w1284 -> [w1320]
                      frame #0 {
                        w1294 = 10  # No. of columns
                        (unwired) "%016.6f" ("Arrays format")
                        n582 = Initialize Array(1.0 ("element"), w1294) -> (w1295:dbl[])
                        n583 = for {
                          N: w1294 -> [_]
                          tunnel: w1298 -> [w1317]
                          tunnel: [w1316] -> w1297 mode=indexing
                          tunnel: w1295 -> [w1315] mode=indexing
                          i -> [w1319]
                          n584 = call "MultiRegionData.vi"("Action"=T7."Read Array", "Array No."=w1319, "Region index"=w1317) -> ("Array OUT"=w1316:dbl[])  [unwired: 3 in, 1 out]
                          n585 = Multiply(x=w1316, y=w1315) -> ()  [unwired: 1 out]
                        }
                        n586 = Concatenate Strings("Saving data for " ("string"), w1300) -> (w1313:string)
                        n587 = local write "Status"(w1313) -> ()
                        n588 = local read "Temperature Progression"() -> (w1305:T3)
                        n589 = local read "probe points per region"() -> (w1314:i32[])
                        n590 = Transpose 2D Array(2D array=w1297) -> (transposed array=w1299:dbl[][])
                        n591 = Unbundle By Name(w1305) -> ("Temperature Array [°C]"=w1304:dbl[], "Humidity Array [RH %]"=w1303:dbl[])
                        n592 = Index Array(array=w1314, index=w1298) -> (element=w1310:i32)
                        n593 = call <vilib>:"Std Deviation and Variance.vi"("X"=w1304) -> ("mean"=w1307:dbl)  [unwired: 1 in, 2 out]
                        n594 = call <vilib>:"Std Deviation and Variance.vi"("X"=w1303) -> ("mean"=w1306:dbl)  [unwired: 1 in, 2 out]
                        n595 = call "SaveDataFile.vi"("Data Array"=w1299, "Temperature"=w1307, "Humidity"=w1306, "no. of arrays"=w1294, "Actual array lengths"=w1310, "Array Titles"="ProbeplanIndex\tCurrent[nA] PinholeFlag\tCapacitance[pF]\tResistance[MOhm]\tLeakage[nA]\tTemperature[DegC]\tHumidity[%]\tChutckTemp[DegC]\tTimestamp[Unix]", "Strip Segment"=w1300, "Arrays format"="%^g") -> ("Filename OUT"=w1301:string, "Pathname OUT"=w1302:string, "Path + Filename OUT"=w1308:string)  [unwired: 4 in, 1 out]
                      }
                      frame #1 {
                        n596 = local read "probe points per region"() -> (w1332:i32[])
                        n597 = local read "max scale array"() -> (w1331:i32[])
                        n598 = local read "min scale array"() -> (w1330:i32[])
                        n599 = local read "Thresholds"() -> (w1334:T1)
                        n600 = Index Array(array=w1332, index=w1323) -> (element=w1324:i32)
                        n601 = call "DisplayStriptestData.vi"("min scale array"=w1330, "max scale array"=w1331, "# probed"=w1324, "Display Stats?"=TRUE, "Thresholds"=w1334, "Region"=w1323) -> ("Strip Quality Data"=w1329:T16)  [unwired: 4 out]
                        n602 = Unbundle By Name(w1329) -> ("pass Rate in %"=w1322:dbl, "Bad channel list"=w1328:i32[], "No of bad strips"=w1327:i32, "Defect description list"=w1326:i32[])
                        n603 = call "CreateDefectFile.vi"("Segment:"=w1320, "Pass rate"=w1322, "Defect description list"=w1326, "Bad channel array"=w1328, "No of bad strips"=w1327, "Filename IN"=w1321) -> ("passed"=w1325:bool)  [unwired: 3 in, 2 out]
                      }
                    }
                  }
                }
                n604 = call <vilib>:"Space Constant.vi"() -> ("String"=w1273:string)
                n605 = Concatenate Strings(w1271, w1273, w1272) -> (w1274:string)
              }
              n606 = Array Max & Min(array=w1265) -> (min value=w1264:dbl)  [unwired: 3 out]
              n607 = And Array Elements(Boolean array=w1267) -> (logical AND=w1266:bool)
              "Module failed/passed" <- w1266
              n608 = call <vilib>:"Space Constant.vi"() -> ("String"=w1262:string)
              n609 = Concatenate Strings(w1263, w1262, w1260) -> (w1261:string)
            }
          }
          n610 = case shown="True" w978 {
            tunnel: w980 -> [w1008 w1010]
            tunnel: [w1008 w1009] -> w979
            frame False {
            }
            frame True {
              n611 = flat-sequence {
                tunnel: [w1011] -> w1009
                tunnel: w1010 -> [w1011]
                frame #0 {
                  w1019 = "_"
                  w1016 = "\\"
                  # "log the temperature file"
                  n612 = global read "QC_RunInformation.vi" "Run info"() -> (w1035:T12)
                  n613 = Unbundle By Name(w1035) -> ("Device Category:"=w1037:string, "Batch:"=w1038:string, "Wafer Serial No.:"=w1039:string, "Sensor Serial No.:"=w1040:string, "Test"=w1043:string)
                  n614 = global read "QC_RunInformation.vi" "LocalConfiguration"() -> (w1034:T18)
                  n615 = Unbundle By Name(w1034) -> ("Data directory"=w1036:string)
                  n616 = Concatenate Strings(w1039, "-", w1040) -> (w1042:string)
                  n617 = Concatenate Strings(w1042, w1019, w1043, w1019, "temperature.log" ("string")) -> (w1044:string)
                  n618 = Concatenate Strings(w1036, w1016, w1037, w1016, w1038, w1016, w1039, w1016, w1042, w1016, w1043, w1016) -> (w1041:string)
                  n619 = Concatenate Strings(w1041, w1044) -> (w1020:string)
                  n620 = String To Path(string=w1020) -> (path=w1021:path)
                  n621 = Open/Create/Replace File(file path (use dialog)=w1021, operation (0:open)=T8."open or create", access (0:read/write)=enum16{"read/write", "read-only", "write-only"}."write-only") -> (refnum out=w1022:refnum<file>, error out=w1029:errorcluster)  [unwired: 3 in, 1 out]
                  n622 = Set File Position(offset (in bytes) (0)=i64 0, refnum=w1022, from (0:start)=enum16{"start", "end", "current"}."end", error in=w1029) -> (refnum out=w1028:refnum<file>, error out=w1030:errorcluster)
                  n623 = local read "Temperature Progression"() -> (w1023:T3)
                  n624 = Unbundle By Name(w1023) -> ("Time Array"=w1024:string[], "Temperature Array [°C]"=w1025:dbl[], "Humidity Array [RH %]"=w1026:dbl[])
                  n625 = for {
                    tunnel: w1024 -> [w1053] mode=indexing
                    tunnel: w1025 -> [w1052] mode=indexing
                    tunnel: w1026 -> [w1049] mode=indexing
                    tunnel: [w1045] -> w1027 mode=indexing
                    w1047 = FALSE ("use system decimal point (T)")
                    w1050 = "\t"
                    n626 = Number To Engineering String(1:w1047, 4:w1052) -> (0:w1051:string)  [unwired: 2 in]
                    n627 = Number To Engineering String(1:w1047, 4:w1049) -> (0:w1048:string)  [unwired: 2 in]
                    n628 = Concatenate Strings(w1053, w1050, w1051, w1050, w1048, "\r\n") -> (w1045:string)
                  }
                  n629 = Concatenate Strings(w1027) -> (w1031:string)
                  n630 = Write to Text File(file (use dialog)=w1028, text=w1031, error in=w1030) -> (refnum out=w1032:refnum<file>, error out=w1033:errorcluster)  [unwired: 1 in, 1 out]
                  n631 = Close File(refnum=w1032, error in=w1033) -> ()  [unwired: 2 out]
                }
              }
            }
          }
          n632 = local read "Temperature Progression"() -> (w996:T3)
          n633 = Unbundle By Name(w996) -> ("Temperature Array [°C]"=w994:dbl[], "Humidity Array [RH %]"=w995:dbl[])
          n634 = call <vilib>:"Std Deviation and Variance.vi"("X"=w994) -> ("standard deviation"=w988:dbl)  [unwired: 1 in, 2 out]
          n635 = call <vilib>:"Std Deviation and Variance.vi"("X"=w995) -> ("standard deviation"=w987:dbl)  [unwired: 1 in, 2 out]
          n636 = Greater?(x=w988, y=5) -> (0:w985:bool)
          n637 = Greater?(x=w987, y=10) -> (0:w986:bool)
          n638 = Select(t="large temperature fluctuations", s=w985, f=w991) -> (s? t:f=w982:string)
          n639 = Select(t="large humidity fluctuations", s=w986, f=w991) -> (s? t:f=w983:string)
          n640 = Concatenate Strings(w982, "\t", w983) -> (w981:string)
          n641 = call "WriteLogFile.vi"("Automatic warning"=w981, "Data File"=w997, "DUT passed?"=w979, "Value TechSpec criteria"=w998, "Files saved?"=w978) -> ()  [unwired: 6 in, 1 out]
        }
      }
    }
  }
